vi "PRCBE 2600B Test Software V1.0.vi"() -> ()   [LabVIEW 2017]
doc: "Configures a sweep and takes voltage and current readings at each point."
uses:
  <vilib>/Platform/TimedLoop/XDataNode/timing_clust.ctl
  <vilib>/Platform/TimedLoop/XDataNode/nitl_modes.ctl
  <vilib>/Platform/TimedLoop/XDataNode/wakeup.ctl
  <vilib>/Utility/miscctls.llb/LVForegroundBackgroundColorsTypeDef.ctl
  <vilib>/Utility/miscctls.llb/LVSelectionTypeDef.ctl
  <vilib>/Utility/miscctls.llb/LVRowAndColumnUnsignedTypeDef.ctl
  SubVI/Global 1.vi
  <vilib>/Platform/TimedLoop/XDataNode/XDataNode.xnode
  <vilib>/Platform/TimedLoop/XDataNode/XDNodeRunTimeDep.lvlib
  <instrlib>/Keithley 2600 Series/Keithley 2600 Series.lvlib
panel:
  out "XY图":cluster{dbl[], dbl[]}(graph)
  in  "Channel":u16(ring) items=["Channel A", "Channel B"]
  in  "MOSFET CLUS":T1={"StepUnit"=1, "Gate Step"=1.0, "StoptUnit"=1, "StartUnit"=1, "Gate Stop"=10.0, "Gate Start"=-10.0, "Compliance"=0.1, "CompliancetUnit "=2, "Drain "=10.0} {"Drain" min=-200.0 max=200.0 step=0.001 format="%#.3f"; "CompliancetUnit" items=["μA", "mA", "A"]; "StepUnit" items=["mV", "V"]; "Gate Step" min=0.001 max=200.0 step=0.001 format="%#.3f"; "StoptUnit" items=["mV", "V"]; "StartUnit" items=["mV", "V"]; "Gate Stop" min=-200.0 max=200.0 step=0.001 format="%#.3f"; "Gate Start" min=-200.0 max=200.0 step=0.001 format="%#.3f"; "Compliance" min=0.1 max=10 step=1 format="%#.3f"}
  out "RES 4":dbl
  out "RES 3":dbl
  in  "pointsIT 2":u32=10 caption="DataPoints" min=3 max=50000 step=1
  in  "Delay time IT 2":u32=10 caption="Interval time" min=1 max=100000 step=1
  in  "delaytimeUnit IT 2":u16(ring) items=["μs", "ms", "s"]
  out "Sheet 23":string[][](table)
  in  "delaytimeUnit IT":u16(ring) items=["μs", "ms", "s"]
  in  "Delay time IT":u32=10 caption="Interval time" min=1 max=100000 step=1
  in  "pointsIT":u32=10 caption="DataPoints" min=3 max=50000 step=1
  in  "DataPoints":u32=21
  out "Sheet 22":string[][](table)
  out "RES 2":dbl
  in  "Vt CLUS":T2={"Current VT"=-10.0, "CurrUnit VT"=2, "Compliance"=0.1, "CompUnit VT"=1} {"CompUnit VT" items=["mV", "V"]; "Compliance" min=0.001 max=200 step=0.1 format="%#.3f"; "CurrUnit VT" items=["μA", "mA", "A"]; "Current VT" min=0.10000000149011612 max=10.0 step=0.001 format="%#.3f"}
  in  "It CLUS":T3={"VoltageUnit IT"=1, "Voltage IT"=-10.0, "CompCurrIT"=0.1, "CompUnit-IT"=2} {"CompUnit-IT" items=["μA", "mA", "A"]; "VoltageUnit IT" items=["mV", "V"]; "Voltage IT" min=0.001 max=200.0 step=0.001 format="%#.3f"; "CompCurrIT" min=0.1 max=10 step=0.001 format="%#.3f"}
  in  "IV CLUS":T4={"StepUnit"=1, "Step"=1.0, "StoptUnit"=1, "StartUnit"=1, "Stop"=10.0, "Start "=-10.0, "Compliance"=0.1, "CompliancetUnit "=2} {"CompliancetUnit" items=["μA", "mA", "A"]; "StepUnit" items=["mV", "V"]; "Step" min=0.001 max=200.0 step=0.001 format="%#.3f"; "StoptUnit" items=["mV", "V"]; "StartUnit" items=["mV", "V"]; "Stop" min=-200.0 max=200.0 step=0.001 format="%#.3f"; "Start" min=-200.0 max=200.0 step=0.001 format="%#.3f"; "Compliance" min=0.1 max=10 step=1 format="%#.3f"}
  in  "Test Type":enum32{"IV", "IT", "VT", "MOSFET"}(radio)
  in  "Series 2600B":u16(ring) items=["2601B  40V, 10A,100fA", "2602B  40V, 10A,100fA", "2604B  40V, 10A,100fA", "2611B  200V, 10A,100fA", "2612B  200V, 10A,100fA", "2614B  200V, 10A,100fA", "2634B  200V, 10A,1fA", "2635B  200V, 10A,0.1fA", "2636B  200V, 10A,0.1fA"]
  in  "Move All":bool
  in  "Save All":bool
  in  "Clear":bool
  in  "Append":bool
  in  "Stop But":bool
  in  "Repeat":bool
  in  "Save":bool
  in  "SetOK":bool
  in  "Tab Control":T5(tab)
  out "Sheet":string[][](table)
  out "Sheet 2":string[][](table) caption="Sheet"
  out "Sheet 3":string[][](table) caption="Sheet"
  out "Sheet 4":string[][](table) caption="Sheet"
  out "Sheet 5":string[][](table) caption="Sheet"
  out "Sheet 6":string[][](table) caption="Sheet"
  out "Sheet 7":string[][](table) caption="Sheet"
  out "Sheet 8":string[][](table) caption="Sheet"
  out "Sheet 9":string[][](table) caption="Sheet"
  out "Sheet 10":string[][](table) caption="Sheet"
  out "Sheet 11":string[][](table) caption="Sheet"
  out "Sheet 12":string[][](table) caption="Sheet"
  out "Sheet 13":string[][](table) caption="Sheet"
  out "Sheet 14":string[][](table) caption="Sheet"
  out "Sheet 15":string[][](table) caption="Sheet"
  out "Sheet 16":string[][](table) caption="Sheet"
  out "Sheet 17":string[][](table) caption="Sheet"
  out "Sheet 18":string[][](table) caption="Sheet"
  out "Sheet 19":string[][](table) caption="Sheet"
  out "Sheet 20":string[][](table) caption="Sheet"
  out "Sheet 21":string[][](table) caption="Sheet"
  out "RunState":cluster{"Boolean":bool}
  in  "XYConvert":bool
  out "test time":string
  out "Chart":cluster{dbl[], dbl[]}[](graph)
  in  "Source Mode  (0: Voltage)":u16(ring) items=["Voltage", "Current"]
  out "TempChart":cluster{sgl[], dbl[]}[](array[cluster])
  out "AppArray":bool[](array[boolean])
  out "test time":timestamp
  out "RES":dbl
  in  "EXIT":bool
  # "Test Function Parameters"
  # "Chart"
  # "PRCBE  2600B - I-V/I-t/V-t Test Software"
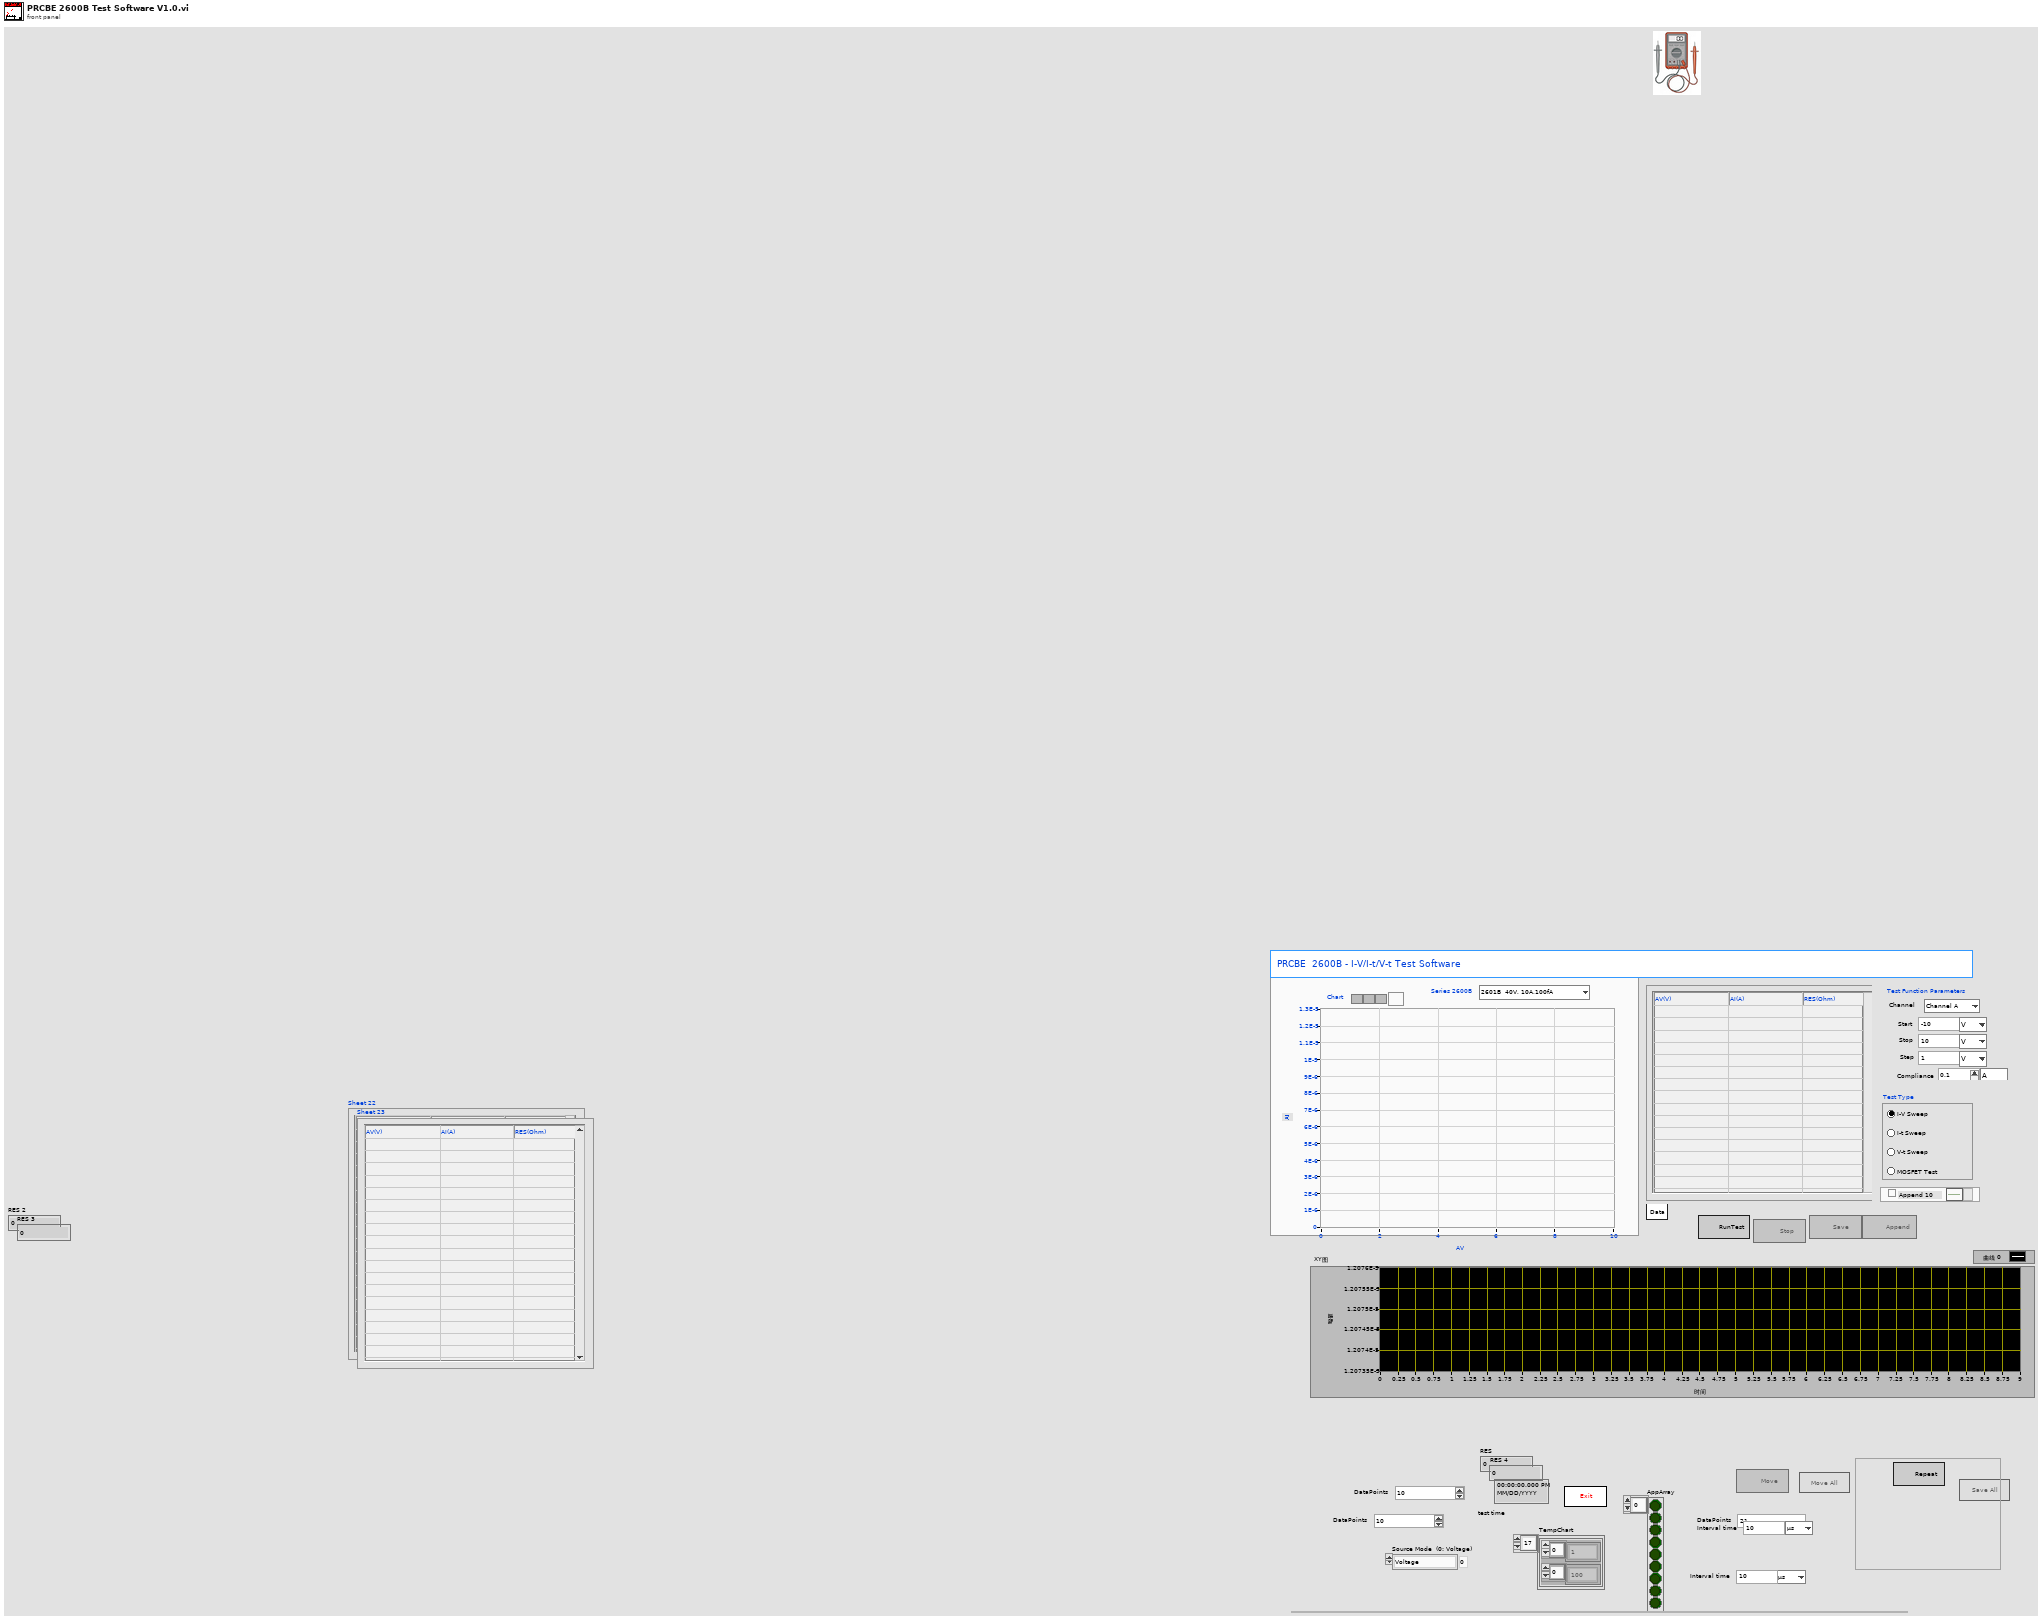
[diagram p1: front panel]
types:
  T1 = cluster{"StepUnit":u16, "Gate Step":dbl, "StoptUnit":u16, "StartUnit":u16, "Gate Stop":dbl, "Gate Start":dbl, "Compliance":sgl, "CompliancetUnit ":u16, "Drain ":dbl}
  T2 = cluster{"Current VT":dbl, "CurrUnit VT":u16, "Compliance":sgl, "CompUnit VT":u16}
  T3 = cluster{"VoltageUnit IT":u16, "Voltage IT":dbl, "CompCurrIT":sgl, "CompUnit-IT":u16}
  T4 = cluster{"StepUnit":u16, "Step":dbl, "StoptUnit":u16, "StartUnit":u16, "Stop":dbl, "Start ":dbl, "Compliance":sgl, "CompliancetUnit ":u16}
  T5 = enum32{"Data", "Append 1", "Append 2", "Append 3", "Append 4", "Append 5", "Append 6", "Append 7", "Append 8", "Append 9", "Append 10", "Append 11", "Append 12", "Append 13", "Append 14", "Append 15", "Append 16", "Append 17", "Append 18", "Append 19", "Append 20"}
  T6 = cluster{"Baud Rate":u32, "Parity":u16, "Data Bits":u16, "Stop Bits":u16, "Flow Control":u16}
  T7 = enum8{"Enabled", "Disabled", "Disabled and Grayed Out"}
  T8 = typedef "XDNodeRunTimeDep.lvlib/timing_clust.ctl" = cluster{"Expected End [f-1]":u64, "Actual End [f-1]":u64, "Finished Late? [f-1]":bool, "Expected End [i-1]":u64, "Actual End [i-1]":u64, "Finished Late? [i-1]":bool, "Expected Start [i]":u64, "Actual Start [i]":u64, "Expected Start [f]":u64, "Actual Start [f]":u64, "Source Name":string, "Structure Name":string, "Period":i64, "Deadline":i64, "Offset":i64, "Start":i64, "Priority":i32, "Timeout":i32, "Mode":T9, "Wakeup Reason":T10, "Error":errorcluster, "Source Type":string, "Secondary Source Type":string, "Global End Time":u64, "Global Start Time":u64, "Frame Duration":u64, "Iteration Duration":u64, "Assigned CPU":i32, "I/O Scan Engine Mode":u32}
  T9 = typedef "XDNodeRunTimeDep.lvlib/nitl_modes.ctl" = enum32{"No Change", "Process missed periods, maintain original phase", "Discard missed periods, maintain original phase", "Process missed periods, ignore original phase", "Discard missed periods, ignore original phase"}
  T10 = typedef "XDNodeRunTimeDep.lvlib/wakeup.ctl" = enum32{"Normal", "Aborted", "Asynchronous wakeup", "Timing source error", "Timed loop error", "Timeout"}
  T11 = cluster{"A 3":string[][], "A 4":string[][], "A 5":string[][], "A 6":string[][], "A 7":string[][], "A 8":string[][], "A 9":string[][], "A 10":string[][], "A 11":string[][], "A 12":string[][], "A 13":string[][], "A 14":string[][], "A 15":string[][], "A 16":string[][], "A 17":string[][], "A 18":string[][], "A 19":string[][], "A 20":string[][], "A 1":string[][], "A 2":string[][]}
  T12 = typedef "LVForegroundBackgroundColorsTypeDef.ctl" = cluster{"Foreground Color":u32, "Background Color":u32}
  T13 = typedef "LVSelectionTypeDef.ctl" = cluster{"Selection Start":u32, "Selection End":u32}
  T14 = enum32{"Current", "Voltage", "IV", "Resistance", "Power"}
  T15 = typedef "LVRowAndColumnUnsignedTypeDef.ctl" = cluster{"Row":u32, "Column":u32}
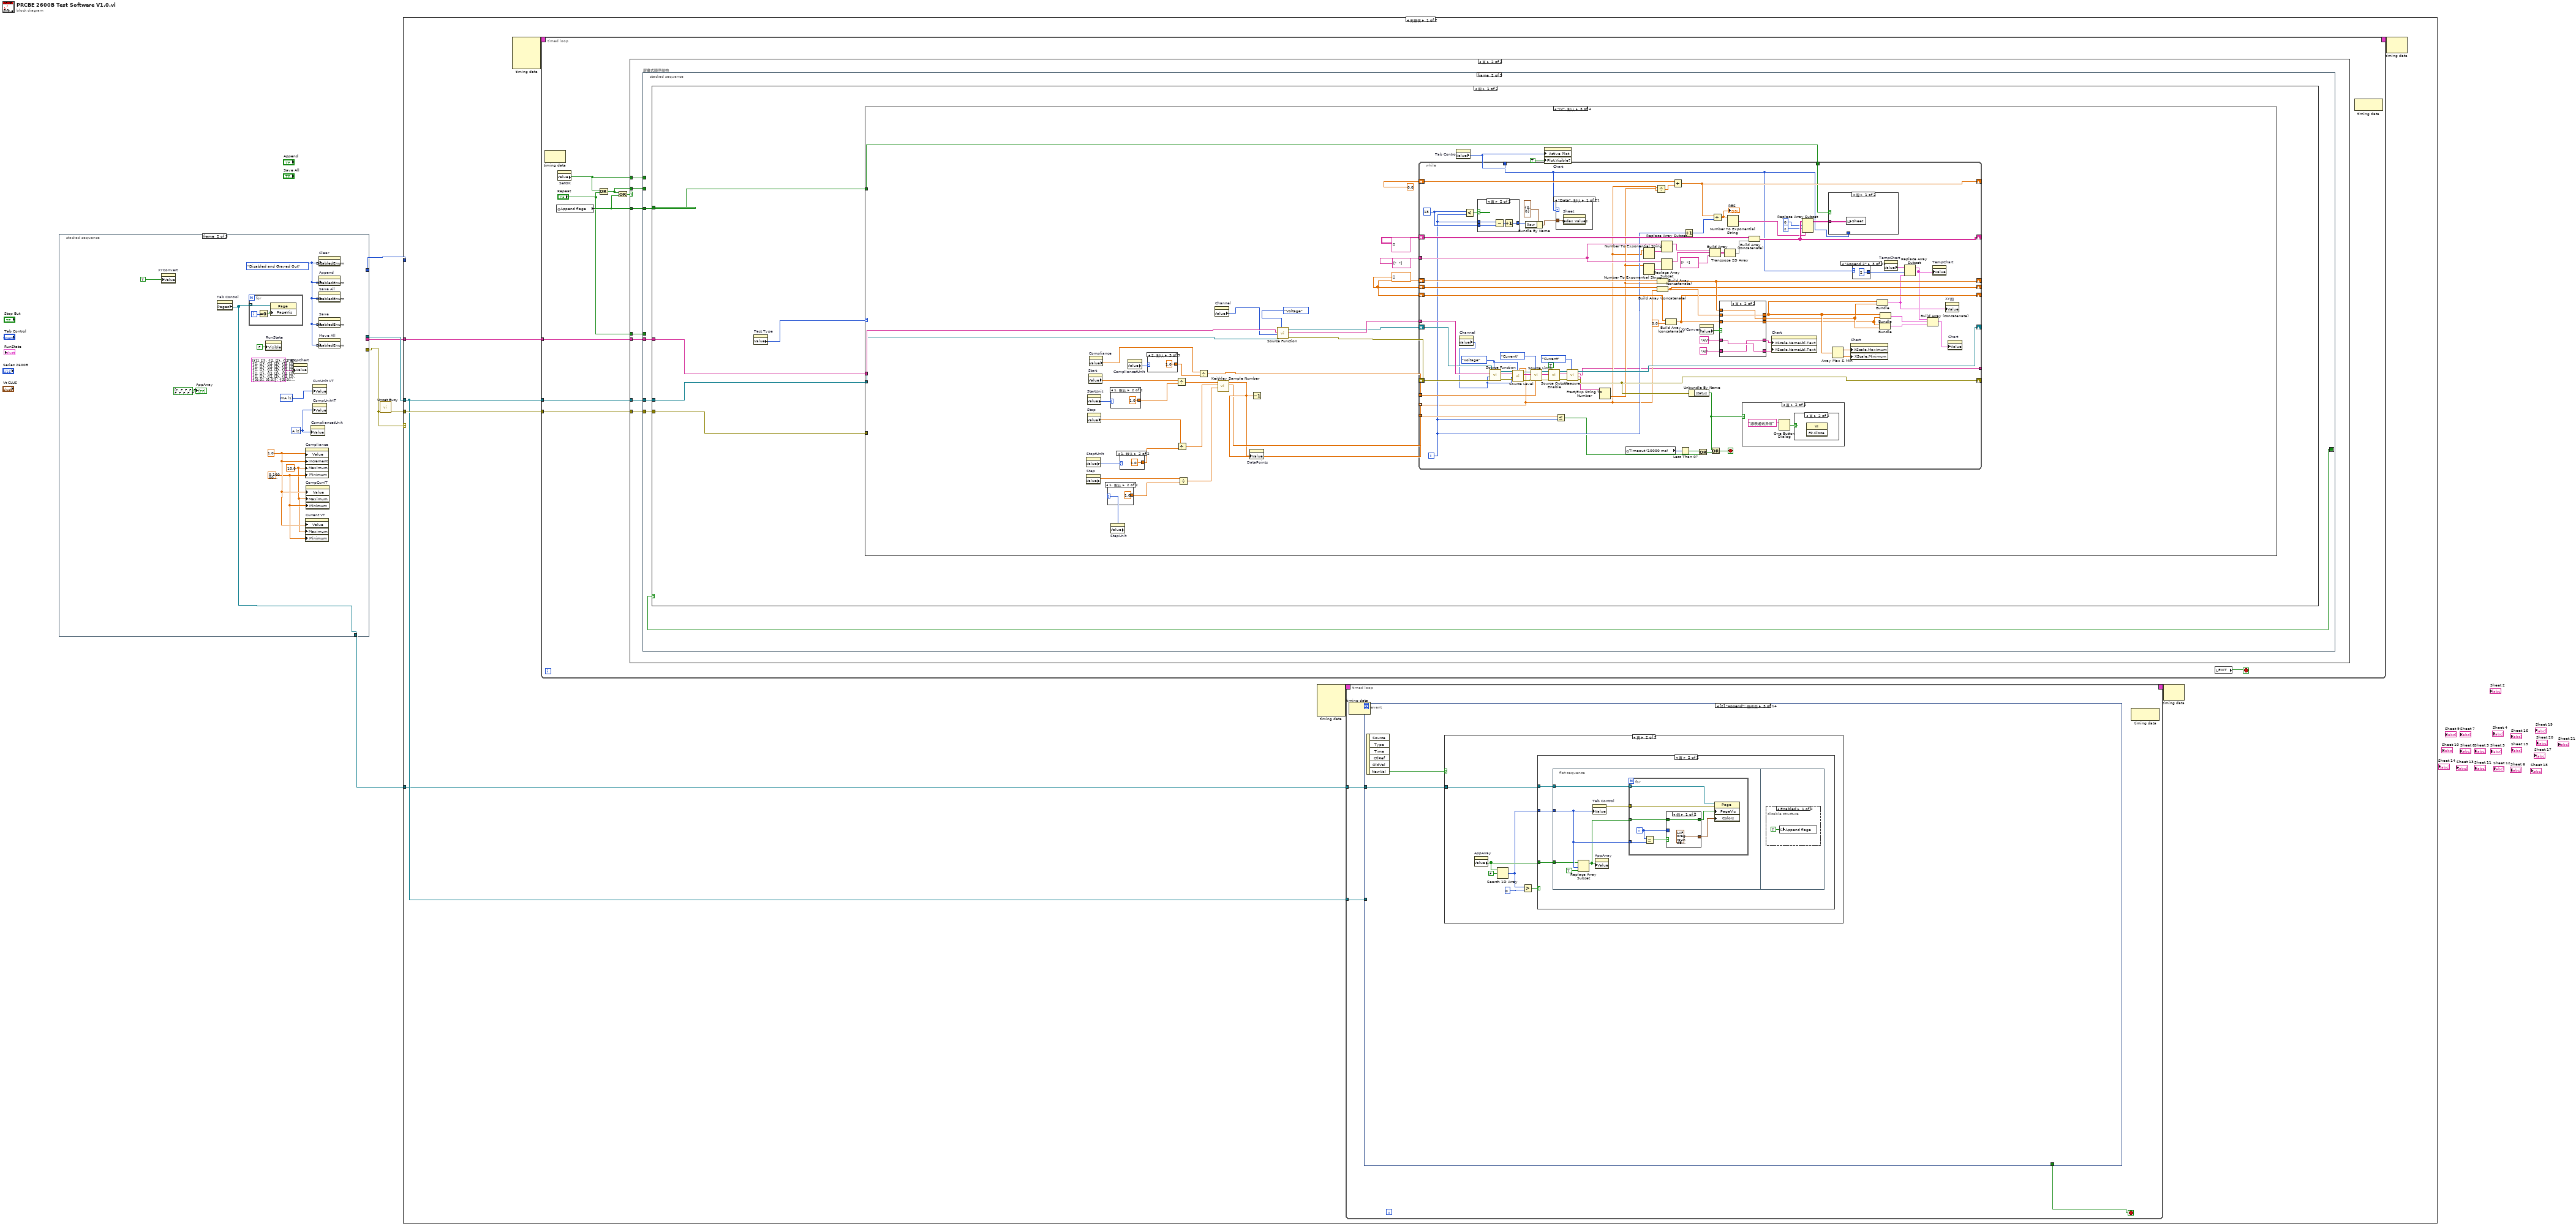
[diagram p0: block diagram]
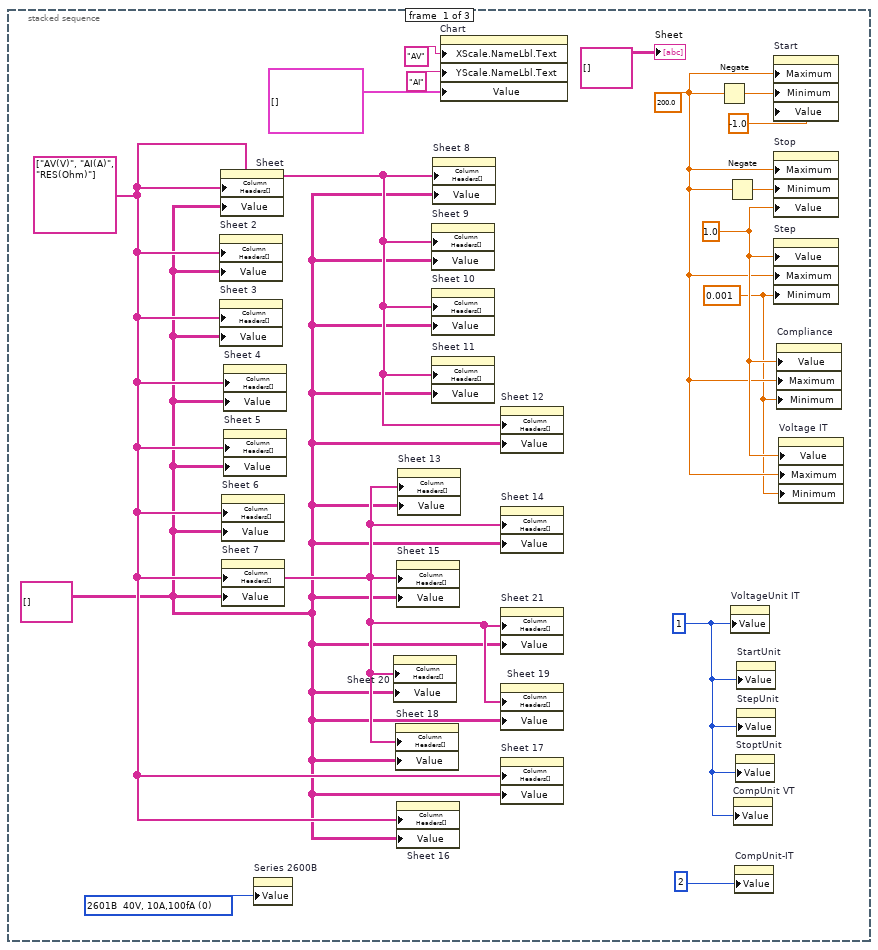
[diagram p2: hidden frame]
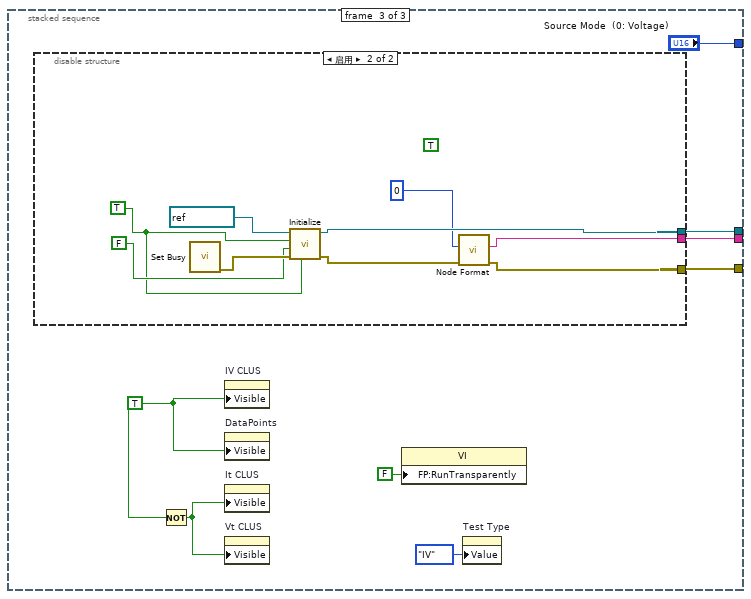
[diagram p3: hidden frame]
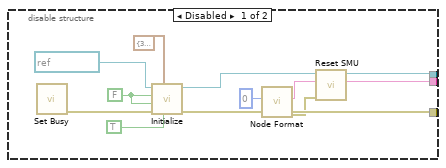
[diagram p4: hidden frame]
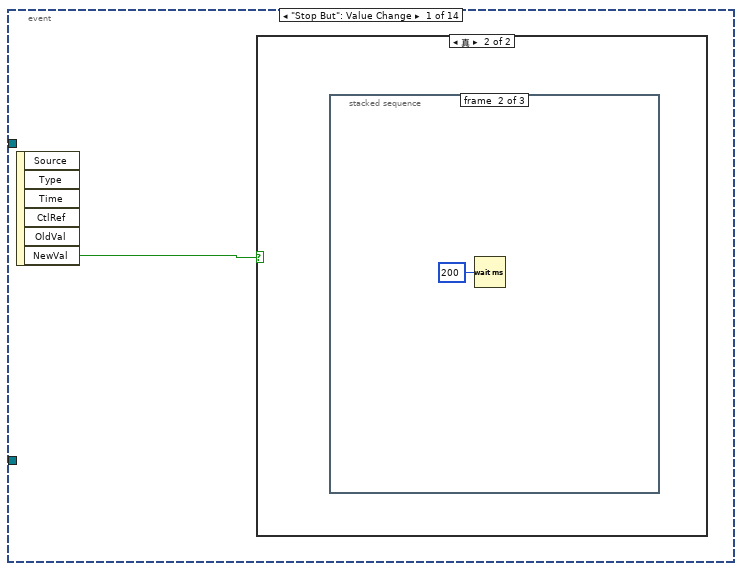
[diagram p5: hidden frame]
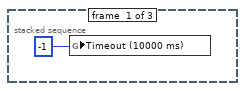
[diagram p7: hidden frame]
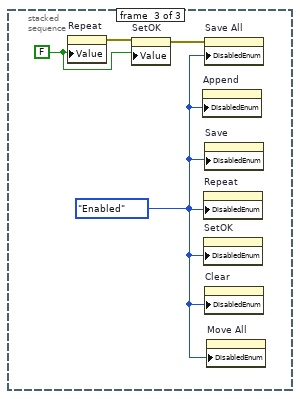
[diagram p8: hidden frame]
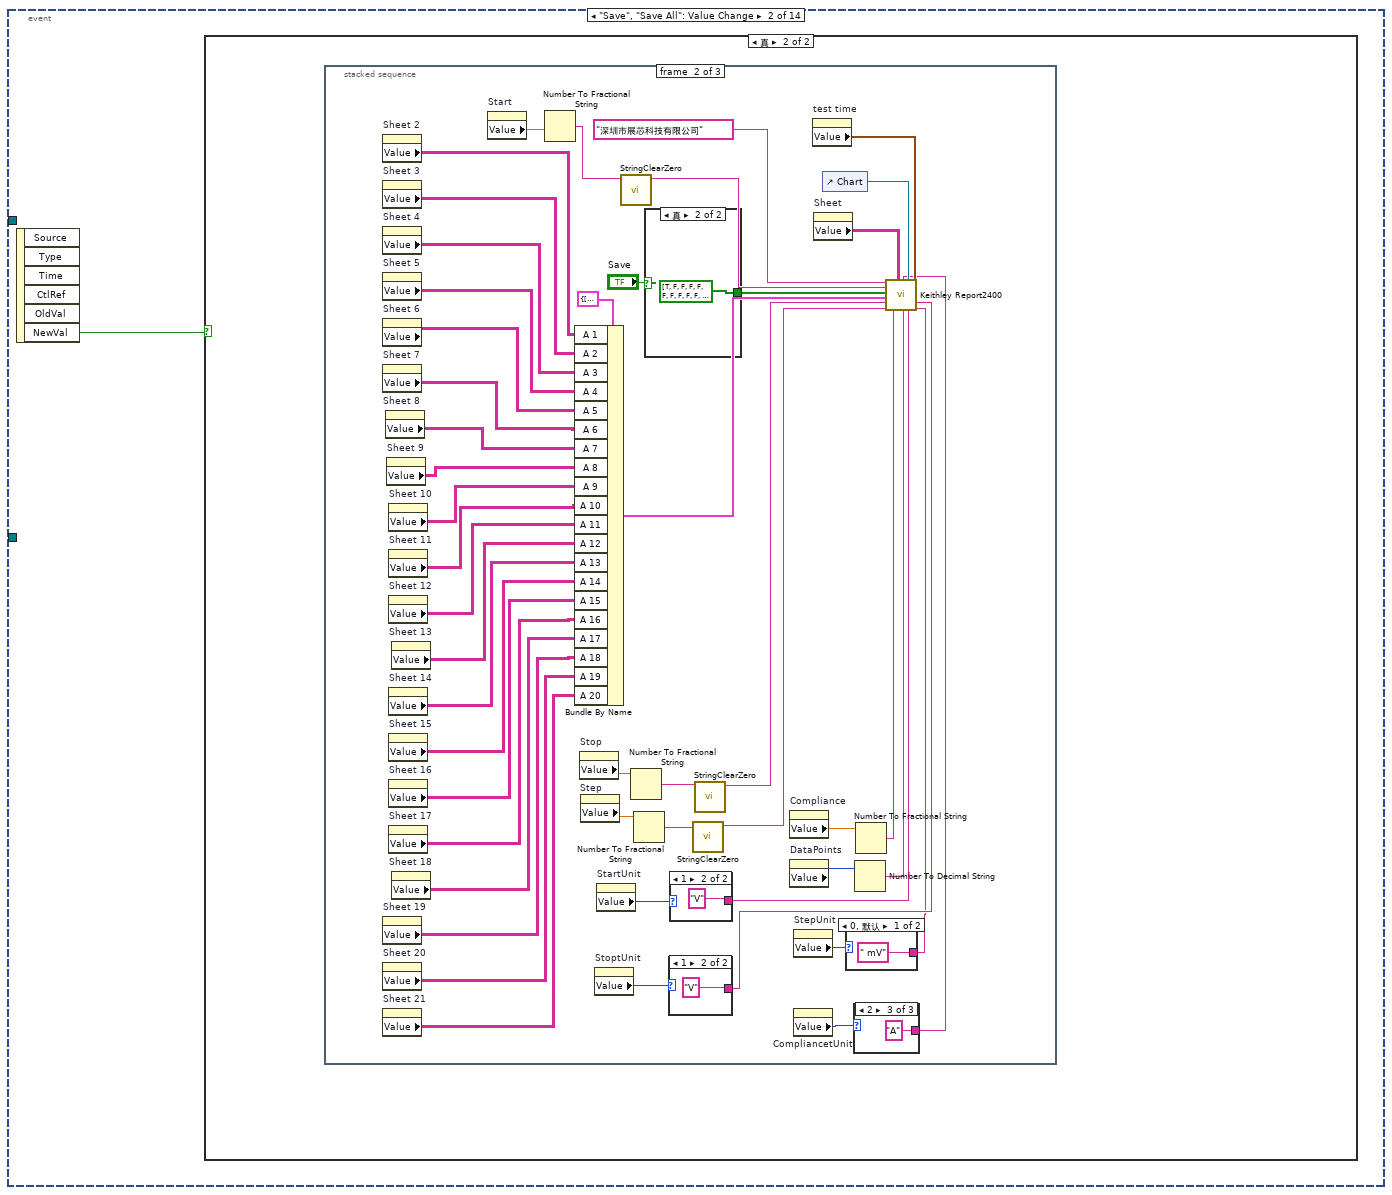
[diagram p9: hidden frame]
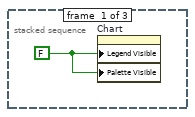
[diagram p11: hidden frame]
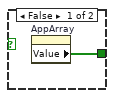
[diagram p12: hidden frame]
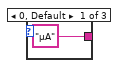
[diagram p13: hidden frame]
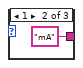
[diagram p14: hidden frame]
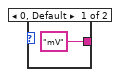
[diagram p15: hidden frame]
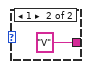
[diagram p16: hidden frame]
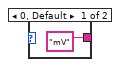
[diagram p17: hidden frame]
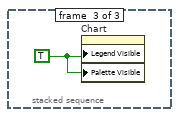
[diagram p18: hidden frame]
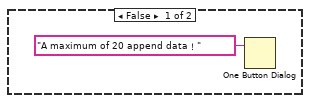
[diagram p20: hidden frame]
diagram:
  n1 = stacked-sequence {
    tunnel: [_ _ "Source Mode  (0: Voltage)"] -> w6
    tunnel: [_ _ w42] -> w5
    tunnel: [_ _ w41] -> w1
    tunnel: [_ w23 _] -> w3
    tunnel: [_ _ w39] -> w2
    frame #0 {
      w8 = u16 1 ("Value")
      w9 = u16 0 items=["2601B  40V, 10A,100fA", "2602B  40V, 10A,100fA", "2604B  40V, 10A,100fA", "2611B  200V, 10A,100fA", "2612B  200V, 10A,100fA", "2614B  200V, 10A,100fA", "2634B  200V, 10A,1fA", "2635B  200V, 10A,0.1fA", "2636B  200V, 10A,0.1fA"] ("Series 2600A")
      w13 = string[][] [] ("Sheet 7")
      w14 = string[] ["AV(V)", "AI(A)", "RES(Ohm)"] ("Column Header Strings[]")
      w10 = 0.001 ("Data Entry Limits:Minimum")
      w11 = 200.0 ("Data Entry Limits:Maximum")
      w12 = 1.0 ("Start")
      n2 = property on="Sheet 2" class="Tbl (严格)"("Column Headers[]"=w14, "Value"=w13) -> ()  [unwired: 2 in, 2 out]
      n3 = property on="Sheet 3" class="Tbl (严格)"("Column Headers[]"=w14, "Value"=w13) -> ()  [unwired: 2 in, 2 out]
      n4 = property on="Sheet" class="Tbl (严格)"("Column Headers[]"=w14, "Value"=w13) -> ()  [unwired: 2 in, 2 out]
      n5 = property on="Sheet 6" class="Tbl (严格)"("Column Headers[]"=w14, "Value"=w13) -> ()  [unwired: 2 in, 2 out]
      n6 = property on="Sheet 7" class="Tbl (严格)"("Column Headers[]"=w14, "Value"=w13) -> ()  [unwired: 2 in, 2 out]
      n7 = property on="Sheet 4" class="Tbl (严格)"("Column Headers[]"=w14, "Value"=w13) -> ()  [unwired: 2 in, 2 out]
      n8 = property on="Sheet 5" class="Tbl (严格)"("Column Headers[]"=w14, "Value"=w13) -> ()  [unwired: 2 in, 2 out]
      n9 = property on="Series 2600B" class="Ring (严格)"("Value"=w9) -> ()  [unwired: 2 in, 2 out]
      n10 = property on="Sheet 20" class="Tbl (严格)"("Column Headers[]"=w14, "Value"=w13) -> ()  [unwired: 2 in, 2 out]
      n11 = property on="Sheet 18" class="Tbl (严格)"("Column Headers[]"=w14, "Value"=w13) -> ()  [unwired: 2 in, 2 out]
      n12 = property on="Sheet 15" class="Tbl (严格)"("Column Headers[]"=w14, "Value"=w13) -> ()  [unwired: 2 in, 2 out]
      n13 = property on="Sheet 16" class="Tbl (严格)"("Column Headers[]"=w14, "Value"=w13) -> ()  [unwired: 2 in, 2 out]
      n14 = property on="Sheet 13" class="Tbl (严格)"("Column Headers[]"=w14, "Value"=w13) -> ()  [unwired: 2 in, 2 out]
      n15 = property on="Sheet 9" class="Tbl (严格)"("Column Headers[]"=w14, "Value"=w13) -> ()  [unwired: 2 in, 2 out]
      n16 = property on="Sheet 10" class="Tbl (严格)"("Column Headers[]"=w14, "Value"=w13) -> ()  [unwired: 2 in, 2 out]
      n17 = property on="Sheet 11" class="Tbl (严格)"("Column Headers[]"=w14, "Value"=w13) -> ()  [unwired: 2 in, 2 out]
      n18 = property on="Sheet 8" class="Tbl (严格)"("Column Headers[]"=w14, "Value"=w13) -> ()  [unwired: 2 in, 2 out]
      n19 = property on="Chart" class="XYGraph (严格)"("XScale.NameLbl.Text"="AV" ("X Scale.Name Label.Text"), "YScale.NameLbl.Text"="AI" ("Y Scale.Name Label.Text"), "Value"=cluster{dbl[], dbl[]}[] [] ("Chart")) -> ()  [unwired: 2 in, 2 out]
      n20 = property on="Sheet 12" class="Tbl (严格)"("Column Headers[]"=w14, "Value"=w13) -> ()  [unwired: 2 in, 2 out]
      n21 = property on="Sheet 14" class="Tbl (严格)"("Column Headers[]"=w14, "Value"=w13) -> ()  [unwired: 2 in, 2 out]
      n22 = property on="Sheet 21" class="Tbl (严格)"("Column Headers[]"=w14, "Value"=w13) -> ()  [unwired: 2 in, 2 out]
      n23 = property on="Sheet 19" class="Tbl (严格)"("Column Headers[]"=w14, "Value"=w13) -> ()  [unwired: 2 in, 2 out]
      n24 = property on="Sheet 17" class="Tbl (严格)"("Column Headers[]"=w14, "Value"=w13) -> ()  [unwired: 2 in, 2 out]
      n25 = Negate(x=w11) -> (-x=w19:dbl)
      n26 = Negate(x=w11) -> (-x=w18:dbl)
      n27 = property on="VoltageUnit IT" class="Ring (严格)"("Value"=w8) -> ()  [unwired: 2 in, 2 out]
      n28 = property on="CompUnit VT" class="Ring (严格)"("Value"=w8) -> ()  [unwired: 2 in, 2 out]
      n29 = property on="CompUnit-IT" class="Ring (严格)"("Value"=u16 2) -> ()  [unwired: 2 in, 2 out]
      n30 = property on="StoptUnit" class="Ring (严格)"("Value"=w8) -> ()  [unwired: 2 in, 2 out]
      n31 = property on="StartUnit" class="Ring (严格)"("Value"=w8) -> ()  [unwired: 2 in, 2 out]
      n32 = property on="StepUnit" class="Ring (严格)"("Value"=w8) -> ()  [unwired: 2 in, 2 out]
      n33 = property on="Start" class="DigNum (严格)"("Maximum"=w11, "Minimum"=w19, "Value"=-1.0 ("Start")) -> ()  [unwired: 2 in, 2 out]
      n34 = property on="Stop" class="DigNum (严格)"("Maximum"=w11, "Minimum"=w18, "Value"=w12) -> ()  [unwired: 2 in, 2 out]
      n35 = property on="Step" class="DigNum (严格)"("Value"=w12, "Maximum"=w11, "Minimum"=w10) -> ()  [unwired: 2 in, 2 out]
      n36 = property on="Compliance" class="DigNum (严格)"("Value"=w12, "Maximum"=w11, "Minimum"=w10) -> ()  [unwired: 2 in, 2 out]
      n37 = property on="Voltage IT" class="DigNum (严格)"("Value"=w12, "Maximum"=w11, "Minimum"=w10) -> ()  [unwired: 2 in, 2 out]
      "Sheet" <- string[][] [] ("Sheet")
    }
    frame #1 {
      w22 = u16 1 items=["μA", "mA", "A"] ("CompliancetUnit")
      w26 = sgl 0.1 ("Compliance")
      w25 = 10.0 ("Data Entry Limits:Maximum")
      w27 = sgl 1.0 ("Compliance")
      w28 = u16 2 items=["μA", "mA", "A"] ("CompliancetUnit")
      w29 = T7."Disabled and Grayed Out" ("Disabled")
      n38 = property on="XYConvert" class="Bool (严格)"("Value"=TRUE) -> ()  [unwired: 2 in, 2 out]
      n39 = property on="Tab Control" class="TabCtl (严格)"() -> ("Pages"=w23:refnum<vi>[])  [unwired: 2 in, 2 out]
      n40 = for {
        tunnel: w23 -> [w34] mode=indexing
        i -> [w35]
        n41 = Equal To 0?(x=w35) -> (x = 0?=w33:bool)
        n42 = property class="Page"(reference=w34, "PageVis"=w33) -> ()  [unwired: 1 in, 2 out]
      }
      n43 = property on="RunState" class="Clust (严格)"("Visible"=FALSE) -> ()  [unwired: 2 in, 2 out]
      n44 = property on="TempChart" class="Arr (严格)"("Value"=cluster{dbl[], sgl[]}[] [{[], []}, {[], []}, {[], []}, {[], []}, {[], []}, {[], []}, {[], []}, {[], []}, {[], []}, {[], []}, {[], []}, {[], []}, {[], []}, {[], []}, {[], []}, {[], []}, {[], []}, {[], []}, {[0.0], [0.0]}, {[0.0], [0.0]}, {[0.0], [0.0]}] ("TempChart")) -> ()  [unwired: 2 in, 2 out]
      n45 = property on="Compliance" class="DigNum (严格)"("Value"=w27, "Increment"=w27, "Maximum"=w25, "Minimum"=w26) -> ()  [unwired: 2 in, 2 out]
      n46 = property on="Current VT" class="DigNum (严格)"("Value"=w27, "Maximum"=w25, "Minimum"=w26) -> ()  [unwired: 2 in, 2 out]
      n47 = property on="CompCurrIT" class="DigNum (严格)"("Value"=w27, "Maximum"=w25, "Minimum"=w26) -> ()  [unwired: 2 in, 2 out]
      n48 = property on="CompliancetUnit" class="Ring (严格)"("Value"=w28) -> ()  [unwired: 2 in, 2 out]
      n49 = property on="CurrUnit VT" class="Ring (严格)"("Value"=w22) -> ()  [unwired: 2 in, 2 out]
      n50 = property on="CompUnit-IT" class="Ring (严格)"("Value"=w28) -> ()  [unwired: 2 in, 2 out]
      n51 = property on="Clear" class="Bool (严格)"("DisabledEnum"=w29) -> ()  [unwired: 2 in, 2 out]
      n52 = property on="Append" class="Bool (严格)"("DisabledEnum"=w29) -> ()  [unwired: 2 in, 2 out]
      n53 = property on="Save All" class="Bool (严格)"("DisabledEnum"=w29) -> ()  [unwired: 2 in, 2 out]
      n54 = property on="Save" class="Bool (严格)"("DisabledEnum"=w29) -> ()  [unwired: 2 in, 2 out]
      n55 = property on="Move All" class="Bool (严格)"("DisabledEnum"=w29) -> ()  [unwired: 2 in, 2 out]
      "AppArray" <- bool[] [TRUE, FALSE, FALSE, FALSE, FALSE, FALSE, FALSE, FALSE, FALSE, FALSE, FALSE, FALSE, FALSE, FALSE, FALSE, FALSE, FALSE, FALSE, FALSE, FALSE, FALSE] ("AppArray")
    }
    frame #2 {
      w36 = TRUE ("Visible")
      n56 = disable-structure shown="启用" {
        disable-tunnel: [w45 w61] -> w42
        disable-tunnel: [w50 w58] -> w41
        disable-tunnel: [w44 w59] -> w39
        frame Disabled {
          w53 = FALSE ("ID Query (True)")
          n57 = call <vilib>:"Set Busy.vi"() -> ("error out"=w55:errorcluster)  [unwired: 10 in, 1 out]
          n58 = call <instrlib>:"Initialize.vi"("Reset (True)"=TRUE, 7:T6 {"Baud Rate"=38400, "Parity"=0, "Data Bits"=7, "Stop Bits"=10, "Flow Control"=0} ("Serial Configuration"), "error in (no error)"=w55, "Error Query (False)"=w53, "ID Query (True)"=w53, "VISA resource name"=refnum<visa-resource-name> "COM1") -> ("error out"=w50:errorcluster, "VISA resource name out"=w47:refnum<visa-resource-name>)  [unwired: 4 out]
          n59 = call <instrlib>:"Node Format.vi"("Node (0-64)"=i8 0) -> ("error out"=w49:errorcluster, "Formatted Node"=w48:string)  [unwired: 1 in, 8 out]
          n60 = call <instrlib>:"Reset SMU.vi"("error in (no error)"=w49, "Node In"=w48, "VISA resource name"=w47) -> ("Node Out"=w44:string, "VISA resource name out"=w45:refnum<visa-resource-name>)  [unwired: 2 in, 5 out]
        }
        frame Enabled {
          w56 = TRUE
          (unwired) TRUE
          n61 = call <vilib>:"Set Busy.vi"() -> ("error out"=w64:errorcluster)  [unwired: 10 in, 1 out]
          n62 = call <instrlib>:"Initialize.vi"("Reset (True)"=w56, "error in (no error)"=w64, "Error Query (False)"=FALSE, "ID Query (True)"=w56, "VISA resource name"=refnum<visa-resource-name> "COM1") -> ("error out"=w62:errorcluster, "VISA resource name out"=w61:refnum<visa-resource-name>)  [unwired: 5 out]
          n63 = call <instrlib>:"Node Format.vi"("error in"=w62, "Node (0-64)"=0) -> ("error out"=w58:errorcluster, "Formatted Node"=w59:string)  [unwired: 8 in]
        }
      }
      n64 = Not(x=w36) -> (.not. x?=w37:bool)
      n65 = property on="IV CLUS" class="Clust (严格)"("Visible"=w36) -> ()  [unwired: 2 in, 2 out]
      n66 = property on="DataPoints" class="DigNum (严格)"("Visible"=w36) -> ()  [unwired: 2 in, 2 out]
      n67 = property on="It CLUS" class="Clust (严格)"("Visible"=w37) -> ()  [unwired: 2 in, 2 out]
      n68 = property on="Vt CLUS" class="Clust (严格)"("Visible"=w37) -> ()  [unwired: 2 in, 2 out]
      n69 = property class="VI"("FP:RunTransparently"=FALSE ("Front Panel Window:Run VI Transparently")) -> ()  [unwired: 2 in, 2 out]
      n70 = property on="Test Type" class="RadioBtnsControl (严格)"("Value"=enum32{"IV", "IT", "VT", "MOSFET"}."IV" ("Test Type")) -> ()  [unwired: 2 in, 2 out]
    }
  }
  n71 = call <vilib>:"Unset Busy.vi"("error in (no error)"=w1) -> ("error out"=w4:errorcluster)  [unwired: 10 in]
  n72 = case shown="无错误" w1 {
    tunnel: w6 -> [_ _]
    tunnel: w4 -> [w72 _]
    tunnel: w5 -> [w71 _]
    tunnel: w3 -> [w70 _]
    tunnel: w2 -> [w65 _]
    frame No Error {
      n73 = node-c288() -> (w69:T8)  [unwired: 4 in]
      n74 = timed-loop {
        tunnel: w71 -> [w632]
        tunnel: w72 -> [w631]
        timing: w69 -> [_]
        timing-out: [_] -> w68
        tunnel: w65 -> [w624]
        stop <- w630 stop-if-true
        n75 = node-c288() -> ()  [unwired: 1 in, 1 out]
        n76 = global read "Global 1.vi" "Append flage"() -> (w629:bool)
        n77 = property on="SetOK" class="Bool (严格)"() -> ("Value"=w625:bool)  [unwired: 2 in, 2 out]
        n78 = Compound Arithmetic op=OR(w625, "Repeat") -> (w627:bool)
        n79 = Compound Arithmetic op=OR(w627, w629) -> (w628:bool)
        n80 = case shown="真" w628 {
          tunnel: w632 -> [_ w646]
          tunnel: w631 -> [_ w645]
          tunnel: w625 -> [_ w644]
          tunnel: w629 -> [_ w643]
          tunnel: w627 -> [_ w642]
          tunnel: "Repeat" -> [_ w641]
          tunnel: w624 -> [_ w640]
          frame False {
            n81 = global read "Global 1.vi" "Timeout (10000 ms)"() -> (w636:i32)
            n82 = Greater Than 0?(x=w636) -> (x > 0?=w635:bool)
            n83 = case shown="真" w635 {
              frame False {
                w639 = T7."Enabled" ("Disabled")
                n84 = global write "Global 1.vi" "Timeout (10000 ms)"(100000 ("Timeout (10000 ms)")) -> ()
                n85 = property on="Append" class="Bool (严格)"("DisabledEnum"=w639) -> ()  [unwired: 2 in, 2 out]
                n86 = property on="Repeat" class="Bool (严格)"("DisabledEnum"=w639) -> ()  [unwired: 2 in, 2 out]
                n87 = property on="SetOK" class="Bool (严格)"("DisabledEnum"=w639) -> ()  [unwired: 2 in, 2 out]
                n88 = property on="Save All" class="Bool (严格)"("DisabledEnum"=w639) -> ()  [unwired: 2 in, 2 out]
                n89 = property on="Save" class="Bool (严格)"("DisabledEnum"=w639) -> ()  [unwired: 2 in, 2 out]
                n90 = property on="Clear" class="Bool (严格)"("DisabledEnum"=w639) -> ()  [unwired: 2 in, 2 out]
                n91 = property on="Move All" class="Bool (严格)"("DisabledEnum"=w639) -> ()  [unwired: 2 in, 2 out]
                n92 = property on="Stop But" class="Bool (严格)"("DisabledEnum"=T7."Disabled and Grayed Out" ("Disabled")) -> ()  [unwired: 2 in, 2 out]
              }
              frame True {
              }
            }
          }
          frame True {
            n93 = stacked-sequence "层叠式顺序结构" {
              seq-local: [w649 _ _] -> [_ w730 _]
              tunnel: w646 -> [_ w732 _]
              tunnel: w645 -> [_ w731 _]
              tunnel: w644 -> [_ _ w1588]
              tunnel: w643 -> [w647 w733 w1586]
              tunnel: w642 -> [w648 _ _]
              tunnel: w641 -> [_ _ w1584]
              tunnel: w640 -> [_ w729 _]
              frame #0 {
                n94 = property on="Start" class="DigNum (严格)"() -> ("Value"=w650:dbl)  [unwired: 2 in, 2 out]
                n95 = property on="StartUnit" class="Ring (严格)"() -> ("Value"=w656:u16)  [unwired: 2 in, 2 out]
                n96 = property on="StoptUnit" class="Ring (严格)"() -> ("Value"=w658:u16)  [unwired: 2 in, 2 out]
                n97 = case shown="1, 默认" w658 {
                  tunnel: [1000.0 ("Start") 1.0 ("Start")] -> w655
                  frame 0 {
                  }
                  frame 1, Default {
                  }
                }
                n98 = case shown="1, 默认" w656 {
                  tunnel: [1000.0 ("Start") 1.0 ("Start")] -> w653
                  frame 0 {
                  }
                  frame 1, Default {
                  }
                }
                n99 = property on="StepUnit" class="Ring (严格)"() -> ("Value"=w657:u16)  [unwired: 2 in, 2 out]
                n100 = property on="Step" class="DigNum (严格)"() -> ("Value"=w652:dbl)  [unwired: 2 in, 2 out]
                n101 = property on="Stop" class="DigNum (严格)"() -> ("Value"=w651:dbl)  [unwired: 2 in, 2 out]
                n102 = Divide(x=w650, y=w653) -> (x/y=w660:dbl)
                n103 = Divide(x=w651, y=w655) -> (x/y=w659:dbl)
                n104 = case shown="1, 默认" w657 {
                  tunnel: [1000.0 ("Start") 1.0 ("Start")] -> w654
                  frame 0 {
                  }
                  frame 1, Default {
                  }
                }
                n105 = Subtract(x=w659, y=w660) -> (x-y=w661:dbl)
                n106 = Divide(x=w652, y=w654) -> (x/y=w663:dbl)
                n107 = Absolute Value(x=w661) -> (abs(x)=w662:dbl)
                n108 = Less?(x=w662, y=w663) -> (x < y?=w664:bool)
                n109 = case shown="假" w664 {
                  selector: w664 -> [_ w721]
                  tunnel: w652 -> [w675 _]
                  tunnel: w651 -> [w674 _]
                  tunnel: w650 -> [w673 _]
                  tunnel: [w667 w721] -> w649
                  tunnel: w648 -> [w666 _]
                  tunnel: w647 -> [w665 _]
                  frame False {
                    n110 = Equal To 0?(x=w674) -> (x = 0?=w672:bool)
                    n111 = Equal To 0?(x=w673) -> (x = 0?=w671:bool)
                    n112 = Equal To 0?(x=w675) -> (x = 0?=w669:bool)
                    n113 = And(x=w672, y=w671) -> (x .and. y?=w670:bool)
                    n114 = Or(x=w670, y=w669) -> (x .or. y?=w668:bool)
                    n115 = case shown="假" w668 {
                      selector: w668 -> [w691 w718]
                      tunnel: [w691 w718] -> w667
                      tunnel: w666 -> [w677 _]
                      tunnel: w665 -> [w678 _]
                      frame False {
                        w676 = string[][] [] ("Sheet")
                        w690 = T7."Disabled and Grayed Out" ("Disabled")
                        n116 = Get Date/Time In Seconds() -> (seconds since 1Jan1904=w685:timestamp)
                        "test time" <- w685
                        n117 = case shown="假" w678 {
                          tunnel: w676 -> [w694 w696]
                          frame False {
                            n118 = local write "Sheet"(w694) -> ()
                          }
                          frame True {
                            n119 = property on="Tab Control" class="TabCtl (严格)"() -> ("Value"=w695:T5)  [unwired: 2 in, 2 out]
                            n120 = case shown="\"Append 3\"" w695 {
                              tunnel: w696 -> [_ w697 w698 w699 w700 w701 w702 w703 w704 w705 w706 w707 w708 w709 w710 w711 w712 w713 w714 w715 w716]
                              frame "Data", Default {
                              }
                              frame "Append 1" {
                                n121 = property on="Sheet 2" class="Tbl (严格)"("Value"=w697) -> ()  [unwired: 2 in, 2 out]
                              }
                              frame "Append 2" {
                                n122 = property on="Sheet 3" class="Tbl (严格)"("Value"=w698) -> ()  [unwired: 2 in, 2 out]
                              }
                              frame "Append 3" {
                                n123 = property on="Sheet 4" class="Tbl (严格)"("Value"=w699) -> ()  [unwired: 2 in, 2 out]
                              }
                              frame "Append 4" {
                                n124 = property on="Sheet 5" class="Tbl (严格)"("Value"=w700) -> ()  [unwired: 2 in, 2 out]
                              }
                              frame "Append 5" {
                                n125 = property on="Sheet 6" class="Tbl (严格)"("Value"=w701) -> ()  [unwired: 2 in, 2 out]
                              }
                              frame "Append 6" {
                                n126 = property on="Sheet 7" class="Tbl (严格)"("Value"=w702) -> ()  [unwired: 2 in, 2 out]
                              }
                              frame "Append 7" {
                                n127 = property on="Sheet 8" class="Tbl (严格)"("Value"=w703) -> ()  [unwired: 2 in, 2 out]
                              }
                              frame "Append 8" {
                                n128 = property on="Sheet 9" class="Tbl (严格)"("Value"=w704) -> ()  [unwired: 2 in, 2 out]
                              }
                              frame "Append 9" {
                                n129 = property on="Sheet 10" class="Tbl (严格)"("Value"=w705) -> ()  [unwired: 2 in, 2 out]
                              }
                              frame "Append 10" {
                                n130 = property on="Sheet 11" class="Tbl (严格)"("Value"=w706) -> ()  [unwired: 2 in, 2 out]
                              }
                              frame "Append 11" {
                                n131 = property on="Sheet 12" class="Tbl (严格)"("Value"=w707) -> ()  [unwired: 2 in, 2 out]
                              }
                              frame "Append 12" {
                                n132 = property on="Sheet 13" class="Tbl (严格)"("Value"=w708) -> ()  [unwired: 2 in, 2 out]
                              }
                              frame "Append 13" {
                                n133 = property on="Sheet 14" class="Tbl (严格)"("Value"=w709) -> ()  [unwired: 2 in, 2 out]
                              }
                              frame "Append 14" {
                                n134 = property on="Sheet 15" class="Tbl (严格)"("Value"=w710) -> ()  [unwired: 2 in, 2 out]
                              }
                              frame "Append 15" {
                                n135 = property on="Sheet 16" class="Tbl (严格)"("Value"=w711) -> ()  [unwired: 2 in, 2 out]
                              }
                              frame "Append 16" {
                                n136 = property on="Sheet 17" class="Tbl (严格)"("Value"=w712) -> ()  [unwired: 2 in, 2 out]
                              }
                              frame "Append 17" {
                                n137 = property on="Sheet 18" class="Tbl (严格)"("Value"=w713) -> ()  [unwired: 2 in, 2 out]
                              }
                              frame "Append 18" {
                                n138 = property on="Sheet 19" class="Tbl (严格)"("Value"=w714) -> ()  [unwired: 2 in, 2 out]
                              }
                              frame "Append 19" {
                                n139 = property on="Sheet 20" class="Tbl (严格)"("Value"=w715) -> ()  [unwired: 2 in, 2 out]
                              }
                              frame "Append 20" {
                                n140 = property on="Sheet 21" class="Tbl (严格)"("Value"=w716) -> ()  [unwired: 2 in, 2 out]
                              }
                            }
                          }
                        }
                        n141 = case shown="真" w677 {
                          tunnel: w676 -> [_ w693]
                          frame False {
                          }
                          frame True {
                            n142 = property on="Sheet" class="Tbl (严格)"("Value"=w693) -> ()  [unwired: 2 in, 2 out]
                            n143 = property on="Tab Control" class="TabCtl (严格)"("Value"=T5."Data" ("Tab Control")) -> ()  [unwired: 2 in, 2 out]
                          }
                        }
                        n144 = Get Date/Time String(date format (0)=enum16{"short", "long", "abbreviated"}."short", seconds (now)=w685, want seconds? (F)=TRUE) -> (date string=w683:string, time string=w687:string)
                        n145 = Concatenate Strings(w683, "  " ("string"), w687) -> (→"test time":string)
                        n146 = property on="Stop But" class="Bool (严格)"("DisabledEnum"=T7."Enabled" ("Disabled")) -> ()  [unwired: 2 in, 2 out]
                        n147 = global write "Global 1.vi" "Timeout (10000 ms)"(100000 ("Timeout (10000 ms)")) -> ()
                        n148 = property on="Clear" class="Bool (严格)"("DisabledEnum"=w690) -> ()  [unwired: 2 in, 2 out]
                        n149 = property on="Repeat" class="Bool (严格)"("DisabledEnum"=w690) -> ()  [unwired: 2 in, 2 out]
                        n150 = property on="SetOK" class="Bool (严格)"("DisabledEnum"=w690) -> ()  [unwired: 2 in, 2 out]
                        n151 = property on="Save" class="Bool (严格)"("DisabledEnum"=w690) -> ()  [unwired: 2 in, 2 out]
                        n152 = property on="Save All" class="Bool (严格)"("DisabledEnum"=w690) -> ()  [unwired: 2 in, 2 out]
                        n153 = property on="Append" class="Bool (严格)"("DisabledEnum"=w690) -> ()  [unwired: 2 in, 2 out]
                        n154 = property on="Move All" class="Bool (严格)"("DisabledEnum"=w690) -> ()  [unwired: 2 in, 2 out]
                        n155 = property on="Chart" class="XYGraph (严格)"("Value"=cluster{"Voltage":dbl[], "Current":dbl[]}[] [] ("Graph")) -> ()  [unwired: 2 in, 2 out]
                        n156 = property on="RunState" class="Clust (严格)"("Visible"=TRUE) -> ()  [unwired: 2 in, 2 out]
                      }
                      frame True {
                        w717 = FALSE ("Repeat")
                        n157 = property on="Repeat" class="Bool (严格)"("Value"=w717) -> ()  [unwired: 2 in, 2 out]
                        n158 = property on="SetOK" class="Bool (严格)"("Value"=w717) -> ()  [unwired: 2 in, 2 out]
                        n159 = One Button Dialog(message="Step is not zero or Start and Stop cannot both be zero ！") -> ()  [unwired: 1 in, 1 out]
                      }
                    }
                  }
                  frame True {
                    w720 = FALSE ("Repeat")
                    n160 = One Button Dialog(message="Value out of scan range!") -> ()  [unwired: 1 in, 1 out]
                    n161 = property on="Repeat" class="Bool (严格)"("Value"=w720) -> ()  [unwired: 2 in, 2 out]
                    n162 = property on="SetOK" class="Bool (严格)"("Value"=w720) -> ()  [unwired: 2 in, 2 out]
                  }
                }
              }
              frame #1 {
                n163 = case shown="假" w730 {
                  tunnel: w733 -> [w738 _]
                  tunnel: w732 -> [w736 _]
                  tunnel: w731 -> [w735 _]
                  tunnel: w729 -> [w737 _]
                  frame False {
                    n164 = property on="Test Type" class="RadioBtnsControl (严格)"() -> ("Value"=w734:enum32{"IV", "IT", "VT", "MOSFET"})  [unwired: 2 in, 2 out]
                    n165 = case shown="\"IV\", 默认" w734 {
                      tunnel: w738 -> [w773 w974 w1165 w1382]
                      tunnel: w737 -> [w763 w967 w1139 w1358]
                      tunnel: w736 -> [w764 w968 w1138 w1353]
                      tunnel: w735 -> [w762 w966 _ w1356]
                      frame "IT" {
                        w761 = TRUE
                        w772 = enum32{"Current", "Voltage"}."Voltage" ("Function (Current)")
                        w778 = sgl[] []
                        n166 = call <instrlib>:"Reset SMU.vi"("SMU B (No)"=w761, "SMU A (No)"=w761, "error in (no error)"=w762, "Node In"=w763, "VISA resource name"=w764) -> ("error out"=w758:errorcluster, "Node Out"=w759:string, "VISA resource name out"=w760:refnum<visa-resource-name>)  [unwired: 3 in, 1 out]
                        n167 = property on="Channel" class="Ring (严格)"() -> ("Value"=w739:u16)  [unwired: 2 in, 2 out]
                        n168 = property on="CompCurrIT" class="DigNum (严格)"() -> ("Value"=w752:sgl)  [unwired: 2 in, 2 out]
                        n169 = property on="CompUnit-IT" class="Ring (严格)"() -> ("Value"=w774:u16)  [unwired: 2 in, 2 out]
                        n170 = case shown="1, 默认" w774 {
                          tunnel: [1000000.0 ("Start") 1.0 ("Start") 1000.0 ("Start")] -> w775
                          frame 0 {
                          }
                          frame 1, Default {
                          }
                          frame 2 {
                          }
                        }
                        n171 = Divide(x=w752, y=w775) -> (x/y=w743:dbl)
                        n172 = property on="Voltage IT" class="DigNum (严格)"() -> ("Value"=w767:dbl)  [unwired: 2 in, 2 out]
                        n173 = property on="VoltageUnit IT" class="Ring (严格)"() -> ("Value"=w766:u16)  [unwired: 2 in, 2 out]
                        n174 = case shown="0" w766 {
                          tunnel: [1000.0 ("Start") 1.0 ("Start")] -> w768
                          frame 0 {
                          }
                          frame 1, Default {
                          }
                        }
                        n175 = call <instrlib>:"Source Function.vi"("Function (Current)"=w772, "error in (no error)"=w758, "Channel (Channel A)"=w739, "Node In"=w759, "VISA resource name"=w760) -> ("error out"=w771:errorcluster, "Node Out"=w770:string, "VISA resource name out"=w769:refnum<visa-resource-name>)  [unwired: 4 out]
                        n176 = Divide(x=w767, y=w768) -> (x/y=w765:dbl)
                        n177 = call <instrlib>:"Source Level.vi"("Level (0.000)"=w765, "Function (Current)"=w772, "error in (no error)"=w771, "Channel (Channel A)"=w739, "Node In"=w770, "VISA resource name"=w769) -> ("error out"=w744:errorcluster, "Node Out"=w745:string, "VISA resource name out"=w746:refnum<visa-resource-name>)  [unwired: 3 out]
                        n178 = call <instrlib>:"Source Limit.vi"("Limit (0.000)"=w743, "Function (Current)"=enum32{"Current", "Voltage"}."Current", "error in (no error)"=w744, "Channel (Channel A)"=w739, "Node In"=w745, "VISA resource name"=w746) -> ("error out"=w750:errorcluster, "Node Out"=w749:string, "VISA resource name out"=w748:refnum<visa-resource-name>)  [unwired: 3 out]
                        n179 = call <instrlib>:"Source Output Enable.vi"("Output (Off)"=TRUE, "error in (no error)"=w750, "Channel (Channel A)"=w739, "Node In"=w749, "VISA resource name"=w748) -> ("error out"=w740:errorcluster, "Node Out"=w742:string, "VISA resource name out"=w741:refnum<visa-resource-name>)  [unwired: 4 out]
                        n180 = property on="Tab Control" class="TabCtl (严格)"() -> ("Value"=w777:T5)  [unwired: 2 in, 2 out]
                        n181 = while {
                          tunnel: string[] ["  "] ("transposed array") -> [w803]
                          shift-right: [w804] -> _
                          shift-left: string[][] [] ("transposed array") -> [w850]
                          shift-right: [w843] -> _
                          shift-left: 0.0 ("Y") -> [w846]
                          shift-right: [w832] -> _
                          shift-left: w778 -> [w837]
                          shift-right: [w830] -> _
                          shift-left: w778 -> [w835]
                          shift-right: [w831] -> _
                          shift-left: w778 -> [w836]
                          tunnel: w773 -> [w819]
                          tunnel: w777 -> [w816]
                          tunnel: [w799] -> w756
                          tunnel: w765 -> [w798]
                          tunnel: [w797] -> w757
                          tunnel: [w796] -> w753
                          shift-right: [w795] -> _
                          shift-left: w743 -> [w795]
                          tunnel: w742 -> [w794]
                          tunnel: w741 -> [w793]
                          tunnel: w740 -> [w792]
                          i -> [w807]
                          stop <- w821 stop-if-true
                          w841 = 18 ("x")
                          n182 = property on="Channel" class="Ring (严格)"() -> ("Value"=w791:u16)  [unwired: 2 in, 2 out]
                          n183 = Equal?(x=0, y=w807) -> (x = y?=w806:bool)
                          n184 = Less?(x=w841, y=w807) -> (x < y?=w838:bool)
                          n185 = case shown="真" w838 {
                            tunnel: w807 -> [_ w937]
                            tunnel: w841 -> [_ w936]
                            tunnel: [0 w934] -> w839
                            frame False {
                            }
                            frame True {
                              n186 = Subtract(x=w937, y=w936) -> (x-y=w935:i32)
                              n187 = Increment(x=w935) -> (x+1=w934:i32)
                            }
                          }
                          n188 = call <instrlib>:"Measure.vi"("Function (Current)"=T14."Current", "error in (no error)"=w792, "Channel (Channel A)"=w791, "Node In"=w794, "VISA resource name"=w793) -> ("error out"=w799:errorcluster, "Output"=w811:string, "Node Out"=w797:string, "VISA resource name out"=w796:refnum<visa-resource-name>)  [unwired: 2 in, 1 out]
                          n189 = call "已用时间"("Reset"=w806) -> ("Elapsed Time (s)"=w805:dbl)  [unwired: 11 in, 7 out]
                          n190 = Bundle By Name(cluster=T15 {"Row"=0, "Column"=0} ("Index Values"), "Row"=w839) -> (w815:T15)
                          n191 = Fract/Exp String To Number(string=w811) -> (number=w810:dbl)  [unwired: 3 in, 1 out]
                          n192 = case shown="\"Data\", 默认" w816 {
                            tunnel: w815 -> [w856 w857 w858 w859 w860 w861 w862 w863 w864 w865 w866 w867 w868 w869 w870 w871 w872 w873 w874 w875 w876]
                            frame "Data", Default {
                              n193 = property on="Sheet" class="Tbl (严格)"("Index Values"=w856) -> ()  [unwired: 2 in, 2 out]
                            }
                            frame "Append 1" {
                              n194 = property on="Sheet 2" class="Tbl (严格)"("Index Values"=w857) -> ()  [unwired: 2 in, 2 out]
                            }
                            frame "Append 2" {
                              n195 = property on="Sheet 3" class="Tbl (严格)"("Index Values"=w858) -> ()  [unwired: 2 in, 2 out]
                            }
                            frame "Append 3" {
                              n196 = property on="Sheet 4" class="Tbl (严格)"("Index Values"=w859) -> ()  [unwired: 2 in, 2 out]
                            }
                            frame "Append 4" {
                              n197 = property on="Sheet 5" class="Tbl (严格)"("Index Values"=w860) -> ()  [unwired: 2 in, 2 out]
                            }
                            frame "Append 5" {
                              n198 = property on="Sheet 6" class="Tbl (严格)"("Index Values"=w861) -> ()  [unwired: 2 in, 2 out]
                            }
                            frame "Append 6" {
                              n199 = property on="Sheet 7" class="Tbl (严格)"("Index Values"=w862) -> ()  [unwired: 2 in, 2 out]
                            }
                            frame "Append 7" {
                              n200 = property on="Sheet 8" class="Tbl (严格)"("Index Values"=w863) -> ()  [unwired: 2 in, 2 out]
                            }
                            frame "Append 8" {
                              n201 = property on="Sheet 9" class="Tbl (严格)"("Index Values"=w864) -> ()  [unwired: 2 in, 2 out]
                            }
                            frame "Append 9" {
                              n202 = property on="Sheet 10" class="Tbl (严格)"("Index Values"=w865) -> ()  [unwired: 2 in, 2 out]
                            }
                            frame "Append 10" {
                              n203 = property on="Sheet 11" class="Tbl (严格)"("Index Values"=w866) -> ()  [unwired: 2 in, 2 out]
                            }
                            frame "Append 11" {
                              n204 = property on="Sheet 12" class="Tbl (严格)"("Index Values"=w867) -> ()  [unwired: 2 in, 2 out]
                            }
                            frame "Append 12" {
                              n205 = property on="Sheet 13" class="Tbl (严格)"("Index Values"=w868) -> ()  [unwired: 2 in, 2 out]
                            }
                            frame "Append 13" {
                              n206 = property on="Sheet 14" class="Tbl (严格)"("Index Values"=w869) -> ()  [unwired: 2 in, 2 out]
                            }
                            frame "Append 14" {
                              n207 = property on="Sheet 15" class="Tbl (严格)"("Index Values"=w870) -> ()  [unwired: 2 in, 2 out]
                            }
                            frame "Append 15" {
                              n208 = property on="Sheet 16" class="Tbl (严格)"("Index Values"=w871) -> ()  [unwired: 2 in, 2 out]
                            }
                            frame "Append 16" {
                              n209 = property on="Sheet 17" class="Tbl (严格)"("Index Values"=w872) -> ()  [unwired: 2 in, 2 out]
                            }
                            frame "Append 17" {
                              n210 = property on="Sheet 18" class="Tbl (严格)"("Index Values"=w873) -> ()  [unwired: 2 in, 2 out]
                            }
                            frame "Append 18" {
                              n211 = property on="Sheet 19" class="Tbl (严格)"("Index Values"=w874) -> ()  [unwired: 2 in, 2 out]
                            }
                            frame "Append 19" {
                              n212 = property on="Sheet 20" class="Tbl (严格)"("Index Values"=w875) -> ()  [unwired: 2 in, 2 out]
                            }
                            frame "Append 20" {
                              n213 = property on="Sheet 21" class="Tbl (严格)"("Index Values"=w876) -> ()  [unwired: 2 in, 2 out]
                            }
                          }
                          n214 = global read "Global 1.vi" "Timeout (10000 ms)"() -> (w848:i32)
                          n215 = Number To Exponential String(number=w810) -> (E-format string=w854:string)  [unwired: 3 in]
                          n216 = Number To Exponential String(number=w805) -> (E-format string=w855:string)  [unwired: 3 in]
                          n217 = Divide(x=w798, y=w810) -> (x/y=w845:dbl)
                          n218 = Build Array (concatenate)(w837, w810) -> (w832:dbl[])
                          n219 = Build Array (concatenate)(w836, w805) -> (w831:dbl[])
                          n220 = Replace Array Subset(array=w803, new element=w855) -> (w853:string[])  [unwired: 1 in]
                          n221 = Replace Array Subset(array=w803, new element=w854) -> (w852:string[])  [unwired: 1 in]
                          n222 = Build Array (concatenate)(w835, 0.0 ("Y")) -> (w830:dbl[])
                          n223 = property on="XYConvert" class="Bool (严格)"() -> ("Value"=w833:bool)  [unwired: 2 in, 2 out]
                          n224 = Add(x=w846, y=w845) -> (x+y=w843:dbl)
                          n225 = Less Than 0?(x=w848) -> (x < 0?=w847:bool)
                          n226 = Increment(x=w807) -> (x+1=w844:i32)
                          n227 = Unbundle By Name(w799) -> ("status"=w820:bool)
                          n228 = Or(x=w847, y=FALSE) -> (x .or. y?=w822:bool)
                          n229 = Divide(x=w843, y=w844) -> (x/y=w842:dbl)
                          "RES 2" <- w842
                          n230 = Or(x=w820, y=w822) -> (x .or. y?=w821:bool)
                          n231 = Number To Exponential String(number=w842) -> (E-format string=w802:string)  [unwired: 3 in]
                          n232 = case shown="真" w833 {
                            tunnel: w832 -> [w927 w931]
                            tunnel: w831 -> [w926 w932]
                            tunnel: w830 -> [w925 w930]
                            tunnel: [w927 w932] -> w823
                            tunnel: [w926 w931] -> w814
                            tunnel: [w925 w930] -> w813
                            tunnel: [w924 w928] -> w829
                            tunnel: [w923 w929] -> w828
                            tunnel: "AI" ("X Scale.Name Label.Text") -> [w924 w929]
                            tunnel: "t" ("X Scale.Name Label.Text") -> [w923 w928]
                            frame False {
                            }
                            frame True {
                            }
                          }
                          n233 = Replace Array Subset(array=w803, new element=w802) -> (w801:string[])  [unwired: 1 in]
                          n234 = Build Array(w853, w852, w801) -> (w851:string[][])
                          n235 = Transpose 2D Array(2D array=w851) -> (transposed array=w849:string[][])
                          n236 = case shown="真" w820 {
                            frame False {
                            }
                            frame True {
                              n237 = One Button Dialog(message="源表通讯异常") -> (true=w921:bool)  [unwired: 1 in]
                              n238 = case shown="真" w921 {
                                frame False {
                                }
                                frame True {
                                n239 = invoke class="VI" method="FP.Close"() -> ()  [unwired: 3 in, 3 out]
                                }
                              }
                            }
                          }
                          n240 = Build Array (concatenate)(w850, w849) -> (w804:string[][])
                          n241 = property on="Chart" class="XYGraph (严格)"("XScale.NameLbl.Text"=w829, "YScale.NameLbl.Text"=w828) -> ()  [unwired: 2 in, 2 out]
                          n242 = case shown="假" w819 {
                            tunnel: w804 -> [w898 w900]
                            tunnel: w816 -> [_ w899]
                            frame False {
                              n243 = local write "Sheet"(w898) -> ()
                            }
                            frame True {
                              n244 = case shown="\"Append 20\"" w899 {
                                tunnel: w900 -> [_ w901 w902 w903 w904 w905 w906 w907 w908 w909 w910 w911 w912 w913 w914 w915 w916 w917 w918 w919 w920]
                                frame "Data", Default {
                                }
                                frame "Append 1" {
                                n245 = property on="Sheet 2" class="Tbl (严格)"("Value"=w901) -> ()  [unwired: 2 in, 2 out]
                                }
                                frame "Append 2" {
                                n246 = property on="Sheet 3" class="Tbl (严格)"("Value"=w902) -> ()  [unwired: 2 in, 2 out]
                                }
                                frame "Append 3" {
                                n247 = property on="Sheet 4" class="Tbl (严格)"("Value"=w903) -> ()  [unwired: 2 in, 2 out]
                                }
                                frame "Append 4" {
                                n248 = property on="Sheet 5" class="Tbl (严格)"("Value"=w904) -> ()  [unwired: 2 in, 2 out]
                                }
                                frame "Append 5" {
                                n249 = property on="Sheet 6" class="Tbl (严格)"("Value"=w905) -> ()  [unwired: 2 in, 2 out]
                                }
                                frame "Append 6" {
                                n250 = property on="Sheet 7" class="Tbl (严格)"("Value"=w906) -> ()  [unwired: 2 in, 2 out]
                                }
                                frame "Append 7" {
                                n251 = property on="Sheet 8" class="Tbl (严格)"("Value"=w907) -> ()  [unwired: 2 in, 2 out]
                                }
                                frame "Append 8" {
                                n252 = property on="Sheet 9" class="Tbl (严格)"("Value"=w908) -> ()  [unwired: 2 in, 2 out]
                                }
                                frame "Append 9" {
                                n253 = property on="Sheet 10" class="Tbl (严格)"("Value"=w909) -> ()  [unwired: 2 in, 2 out]
                                }
                                frame "Append 10" {
                                n254 = property on="Sheet 11" class="Tbl (严格)"("Value"=w910) -> ()  [unwired: 2 in, 2 out]
                                }
                                frame "Append 11" {
                                n255 = property on="Sheet 12" class="Tbl (严格)"("Value"=w911) -> ()  [unwired: 2 in, 2 out]
                                }
                                frame "Append 12" {
                                n256 = property on="Sheet 13" class="Tbl (严格)"("Value"=w912) -> ()  [unwired: 2 in, 2 out]
                                }
                                frame "Append 13" {
                                n257 = property on="Sheet 14" class="Tbl (严格)"("Value"=w913) -> ()  [unwired: 2 in, 2 out]
                                }
                                frame "Append 14" {
                                n258 = property on="Sheet 15" class="Tbl (严格)"("Value"=w914) -> ()  [unwired: 2 in, 2 out]
                                }
                                frame "Append 15" {
                                n259 = property on="Sheet 16" class="Tbl (严格)"("Value"=w915) -> ()  [unwired: 2 in, 2 out]
                                }
                                frame "Append 16" {
                                n260 = property on="Sheet 17" class="Tbl (严格)"("Value"=w916) -> ()  [unwired: 2 in, 2 out]
                                }
                                frame "Append 17" {
                                n261 = property on="Sheet 18" class="Tbl (严格)"("Value"=w917) -> ()  [unwired: 2 in, 2 out]
                                }
                                frame "Append 18" {
                                n262 = property on="Sheet 19" class="Tbl (严格)"("Value"=w918) -> ()  [unwired: 2 in, 2 out]
                                }
                                frame "Append 19" {
                                n263 = property on="Sheet 20" class="Tbl (严格)"("Value"=w919) -> ()  [unwired: 2 in, 2 out]
                                }
                                frame "Append 20" {
                                n264 = property on="Sheet 21" class="Tbl (严格)"("Value"=w920) -> ()  [unwired: 2 in, 2 out]
                                }
                              }
                            }
                          }
                          n265 = Array Max & Min(array=w823) -> (max value=w825:dbl, min value=w824:dbl)  [unwired: 2 out]
                          n266 = property on="Chart" class="XYGraph (严格)"("XScale.Maximum"=w825, "XScale.Minimum"=w824) -> ()  [unwired: 2 in, 2 out]
                          n267 = case shown="\"Data\", 默认" w816 {
                            tunnel: [0 ("disabled index (row)") 1 ("disabled index (row)") 2 ("disabled index (row)") 3 ("disabled index (row)") 4 ("disabled index (row)") 5 ("disabled index (row)") 6 ("disabled index (row)") 7 ("disabled index (row)") 8 ("disabled index (row)") 9 ("disabled index (row)") 10 ("disabled index (row)") 11 ("disabled index (row)") 12 ("disabled index (row)") 13 ("disabled index (row)") 14 ("disabled index (row)") 15 ("disabled index (row)") 16 ("disabled index (row)") 17 ("disabled index (row)") 18 ("disabled index (row)") 19 ("disabled index (row)") 20 ("disabled index (row)")] -> w817
                            frame "Data", Default {
                            }
                            frame "Append 1" {
                            }
                            frame "Append 2" {
                            }
                            frame "Append 3" {
                            }
                            frame "Append 4" {
                            }
                            frame "Append 5" {
                            }
                            frame "Append 6" {
                            }
                            frame "Append 7" {
                            }
                            frame "Append 8" {
                            }
                            frame "Append 9" {
                            }
                            frame "Append 10" {
                            }
                            frame "Append 11" {
                            }
                            frame "Append 12" {
                            }
                            frame "Append 13" {
                            }
                            frame "Append 14" {
                            }
                            frame "Append 15" {
                            }
                            frame "Append 16" {
                            }
                            frame "Append 17" {
                            }
                            frame "Append 18" {
                            }
                            frame "Append 19" {
                            }
                            frame "Append 20" {
                            }
                          }
                          n268 = Bundle(w823, w814) -> (w787:cluster{dbl[], dbl[]})  [unwired: 1 in]
                          n269 = Bundle(w813, w814) -> (w812:cluster{dbl[], dbl[]})  [unwired: 1 in]
                          n270 = Bundle(w823, w813) -> (w788:cluster{dbl[], dbl[]})  [unwired: 1 in]
                          n271 = property on="TempChart" class="Arr (严格)"() -> ("Value"=w818:cluster{sgl[], dbl[]}[])  [unwired: 2 in, 2 out]
                          n272 = Replace Array Subset(array=w818, new element=w787, index=w817) -> (w789:cluster{sgl[], dbl[]}[])
                          n273 = Build Array (concatenate)(w789, w788, w812) -> (w790:cluster{dbl[], dbl[]}[])
                          n274 = property on="XY图" class="XYGraph (严格)"("Value"=w787) -> ()  [unwired: 2 in, 2 out]
                          n275 = property on="TempChart" class="Arr (严格)"("Value"=w789) -> ()  [unwired: 2 in, 2 out]
                          n276 = property on="Chart" class="XYGraph (严格)"("Value"=w790) -> ()  [unwired: 2 in, 2 out]
                        }
                        n277 = property on="Chart" class="XYGraph (严格)"("Active Plot"=w777, "Plot.Visible?"=TRUE ("Plot.Visible")) -> ()  [unwired: 2 in, 2 out]
                        n278 = property on="Channel" class="Ring (严格)"() -> ("Value"=w754:u16)  [unwired: 2 in, 2 out]
                        n279 = call <instrlib>:"Source Output Enable.vi"("Output (Off)"=FALSE, "error in (no error)"=w756, "Channel (Channel A)"=w754, "Node In"=w757, "VISA resource name"=w753) -> ()  [unwired: 7 out]
                      }
                      frame "VT" {
                        w942 = enum32{"Current", "Voltage"}."Current" ("Function (Current)")
                        w965 = TRUE
                        w977 = sgl[] []
                        n280 = call <instrlib>:"Reset SMU.vi"("SMU B (No)"=w965, "SMU A (No)"=w965, "error in (no error)"=w966, "Node In"=w967, "VISA resource name"=w968) -> ("error out"=w962:errorcluster, "Node Out"=w963:string, "VISA resource name out"=w964:refnum<visa-resource-name>)  [unwired: 3 in, 1 out]
                        n281 = property on="Channel" class="Ring (严格)"() -> ("Value"=w944:u16)  [unwired: 2 in, 2 out]
                        n282 = property on="Compliance" class="DigNum (严格)"() -> ("Value"=w956:sgl)  [unwired: 2 in, 2 out]
                        n283 = property on="CompUnit VT" class="Ring (严格)"() -> ("Value"=w939:u16)  [unwired: 2 in, 2 out]
                        n284 = case shown="1, 默认" w939 {
                          tunnel: [1000.0 ("Start") 1.0 ("Start")] -> w938
                          frame 0 {
                          }
                          frame 1, Default {
                          }
                        }
                        n285 = Divide(x=w956, y=w938) -> (x/y=w948:dbl)
                        n286 = property on="Current VT" class="DigNum (严格)"() -> ("Value"=w970:dbl)  [unwired: 2 in, 2 out]
                        n287 = property on="CurrUnit VT" class="Ring (严格)"() -> ("Value"=w941:u16)  [unwired: 2 in, 2 out]
                        n288 = call <instrlib>:"Source Function.vi"("Function (Current)"=w942, "error in (no error)"=w962, "Channel (Channel A)"=w944, "Node In"=w963, "VISA resource name"=w964) -> ("error out"=w973:errorcluster, "Node Out"=w972:string, "VISA resource name out"=w971:refnum<visa-resource-name>)  [unwired: 4 out]
                        n289 = case shown="0" w941 {
                          tunnel: [1000000.0 ("Start") 1.0 ("Start") 1000.0 ("Start")] -> w940
                          frame 0 {
                          }
                          frame 1 {
                          }
                          frame 2, Default {
                          }
                        }
                        n290 = Divide(x=w970, y=w940) -> (x/y=w969:dbl)
                        n291 = call <instrlib>:"Source Level.vi"("Level (0.000)"=w969, "Function (Current)"=w942, "error in (no error)"=w973, "Channel (Channel A)"=w944, "Node In"=w972, "VISA resource name"=w971) -> ("error out"=w949:errorcluster, "Node Out"=w950:string, "VISA resource name out"=w951:refnum<visa-resource-name>)  [unwired: 3 out]
                        n292 = call <instrlib>:"Source Limit.vi"("Limit (0.000)"=w948, "Function (Current)"=enum32{"Current", "Voltage"}."Voltage", "error in (no error)"=w949, "Channel (Channel A)"=w944, "Node In"=w950, "VISA resource name"=w951) -> ("error out"=w955:errorcluster, "Node Out"=w954:string, "VISA resource name out"=w953:refnum<visa-resource-name>)  [unwired: 3 out]
                        n293 = call <instrlib>:"Source Output Enable.vi"("Output (Off)"=TRUE, "error in (no error)"=w955, "Channel (Channel A)"=w944, "Node In"=w954, "VISA resource name"=w953) -> ("error out"=w945:errorcluster, "Node Out"=w947:string, "VISA resource name out"=w946:refnum<visa-resource-name>)  [unwired: 4 out]
                        n294 = property on="Tab Control" class="TabCtl (严格)"() -> ("Value"=w976:T5)  [unwired: 2 in, 2 out]
                        n295 = while {
                          tunnel: string[] ["  "] ("transposed array") -> [w999]
                          shift-right: [w1000] -> _
                          shift-left: string[][] [] ("transposed array") -> [w1049]
                          shift-right: [w1042] -> _
                          shift-left: 0.0 ("Y") -> [w1045]
                          shift-right: [w1030] -> _
                          shift-left: w977 -> [w1036]
                          shift-right: [w1028] -> _
                          shift-left: w977 -> [w1034]
                          shift-right: [w1029] -> _
                          shift-left: w977 -> [w1035]
                          tunnel: w974 -> [w1017]
                          tunnel: w976 -> [w1013]
                          tunnel: [w996] -> w960
                          tunnel: w969 -> [w995]
                          tunnel: [w994] -> w961
                          tunnel: [w993] -> w957
                          shift-right: [w992] -> _
                          shift-left: w948 -> [w992]
                          tunnel: w947 -> [w991]
                          tunnel: w946 -> [w990]
                          tunnel: w945 -> [w989]
                          i -> [w1003]
                          stop <- w1019 stop-if-true
                          w1040 = 18 ("x")
                          n296 = property on="Channel" class="Ring (严格)"() -> ("Value"=w988:u16)  [unwired: 2 in, 2 out]
                          n297 = Equal?(x=0, y=w1003) -> (x = y?=w1002:bool)
                          n298 = Less?(x=w1040, y=w1003) -> (x < y?=w1037:bool)
                          n299 = case shown="真" w1037 {
                            tunnel: w1003 -> [_ w1136]
                            tunnel: w1040 -> [_ w1135]
                            tunnel: [0 w1133] -> w1038
                            frame False {
                            }
                            frame True {
                              n300 = Subtract(x=w1136, y=w1135) -> (x-y=w1134:i32)
                              n301 = Increment(x=w1134) -> (x+1=w1133:i32)
                            }
                          }
                          n302 = call <instrlib>:"Measure.vi"("Function (Current)"=enum32{"Current", "Voltage"}."Voltage", "error in (no error)"=w989, "Channel (Channel A)"=w988, "Node In"=w991, "VISA resource name"=w990) -> ("error out"=w996:errorcluster, "Output"=w1007:string, "Node Out"=w994:string, "VISA resource name out"=w993:refnum<visa-resource-name>)  [unwired: 2 in, 1 out]
                          n303 = call "已用时间2"("Reset"=w1002) -> ("Elapsed Time (s)"=w1001:dbl)  [unwired: 11 in, 7 out]
                          n304 = Bundle By Name(cluster=T15 {"Row"=0, "Column"=0} ("Index Values"), "Row"=w1038) -> (w1012:T15)
                          n305 = Fract/Exp String To Number(string=w1007) -> (number=w1006:dbl)  [unwired: 3 in, 1 out]
                          n306 = case shown="\"Data\", 默认" w1013 {
                            tunnel: w1012 -> [w1055 w1056 w1057 w1058 w1059 w1060 w1061 w1062 w1063 w1064 w1065 w1066 w1067 w1068 w1069 w1070 w1071 w1072 w1073 w1074 w1075]
                            frame "Data", Default {
                              n307 = property on="Sheet" class="Tbl (严格)"("Index Values"=w1055) -> ()  [unwired: 2 in, 2 out]
                            }
                            frame "Append 1" {
                              n308 = property on="Sheet 2" class="Tbl (严格)"("Index Values"=w1056) -> ()  [unwired: 2 in, 2 out]
                            }
                            frame "Append 2" {
                              n309 = property on="Sheet 3" class="Tbl (严格)"("Index Values"=w1057) -> ()  [unwired: 2 in, 2 out]
                            }
                            frame "Append 3" {
                              n310 = property on="Sheet 4" class="Tbl (严格)"("Index Values"=w1058) -> ()  [unwired: 2 in, 2 out]
                            }
                            frame "Append 4" {
                              n311 = property on="Sheet 5" class="Tbl (严格)"("Index Values"=w1059) -> ()  [unwired: 2 in, 2 out]
                            }
                            frame "Append 5" {
                              n312 = property on="Sheet 6" class="Tbl (严格)"("Index Values"=w1060) -> ()  [unwired: 2 in, 2 out]
                            }
                            frame "Append 6" {
                              n313 = property on="Sheet 7" class="Tbl (严格)"("Index Values"=w1061) -> ()  [unwired: 2 in, 2 out]
                            }
                            frame "Append 7" {
                              n314 = property on="Sheet 8" class="Tbl (严格)"("Index Values"=w1062) -> ()  [unwired: 2 in, 2 out]
                            }
                            frame "Append 8" {
                              n315 = property on="Sheet 9" class="Tbl (严格)"("Index Values"=w1063) -> ()  [unwired: 2 in, 2 out]
                            }
                            frame "Append 9" {
                              n316 = property on="Sheet 10" class="Tbl (严格)"("Index Values"=w1064) -> ()  [unwired: 2 in, 2 out]
                            }
                            frame "Append 10" {
                              n317 = property on="Sheet 11" class="Tbl (严格)"("Index Values"=w1065) -> ()  [unwired: 2 in, 2 out]
                            }
                            frame "Append 11" {
                              n318 = property on="Sheet 12" class="Tbl (严格)"("Index Values"=w1066) -> ()  [unwired: 2 in, 2 out]
                            }
                            frame "Append 12" {
                              n319 = property on="Sheet 13" class="Tbl (严格)"("Index Values"=w1067) -> ()  [unwired: 2 in, 2 out]
                            }
                            frame "Append 13" {
                              n320 = property on="Sheet 14" class="Tbl (严格)"("Index Values"=w1068) -> ()  [unwired: 2 in, 2 out]
                            }
                            frame "Append 14" {
                              n321 = property on="Sheet 15" class="Tbl (严格)"("Index Values"=w1069) -> ()  [unwired: 2 in, 2 out]
                            }
                            frame "Append 15" {
                              n322 = property on="Sheet 16" class="Tbl (严格)"("Index Values"=w1070) -> ()  [unwired: 2 in, 2 out]
                            }
                            frame "Append 16" {
                              n323 = property on="Sheet 17" class="Tbl (严格)"("Index Values"=w1071) -> ()  [unwired: 2 in, 2 out]
                            }
                            frame "Append 17" {
                              n324 = property on="Sheet 18" class="Tbl (严格)"("Index Values"=w1072) -> ()  [unwired: 2 in, 2 out]
                            }
                            frame "Append 18" {
                              n325 = property on="Sheet 19" class="Tbl (严格)"("Index Values"=w1073) -> ()  [unwired: 2 in, 2 out]
                            }
                            frame "Append 19" {
                              n326 = property on="Sheet 20" class="Tbl (严格)"("Index Values"=w1074) -> ()  [unwired: 2 in, 2 out]
                            }
                            frame "Append 20" {
                              n327 = property on="Sheet 21" class="Tbl (严格)"("Index Values"=w1075) -> ()  [unwired: 2 in, 2 out]
                            }
                          }
                          n328 = global read "Global 1.vi" "Timeout (10000 ms)"() -> (w1047:i32)
                          n329 = Number To Exponential String(number=w1006) -> (E-format string=w1053:string)  [unwired: 3 in]
                          n330 = Number To Exponential String(number=w1001) -> (E-format string=w1054:string)  [unwired: 3 in]
                          n331 = Divide(x=w995, y=w1006) -> (x/y=w1044:dbl)
                          n332 = Build Array (concatenate)(w1036, w1006) -> (w1030:dbl[])
                          n333 = Build Array (concatenate)(w1035, w1001) -> (w1029:dbl[])
                          n334 = Replace Array Subset(array=w999, new element=w1054) -> (w1052:string[])  [unwired: 1 in]
                          n335 = Replace Array Subset(array=w999, new element=w1053) -> (w1051:string[])  [unwired: 1 in]
                          n336 = Build Array (concatenate)(w1034, 0.0 ("Y")) -> (w1028:dbl[])
                          n337 = property on="XYConvert" class="Bool (严格)"() -> ("Value"=w1031:bool)  [unwired: 2 in, 2 out]
                          n338 = Add(x=w1045, y=w1044) -> (x+y=w1042:dbl)
                          n339 = Less Than 0?(x=w1047) -> (x < 0?=w1046:bool)
                          n340 = Increment(x=w1003) -> (x+1=w1043:i32)
                          n341 = Unbundle By Name(w996) -> ("status"=w1018:bool)
                          n342 = Or(x=w1046, y=FALSE) -> (x .or. y?=w1020:bool)
                          n343 = Divide(x=w1042, y=w1043) -> (x/y=w1041:dbl)
                          "RES 3" <- w1041
                          n344 = Or(x=w1018, y=w1020) -> (x .or. y?=w1019:bool)
                          n345 = Number To Exponential String(number=w1041) -> (E-format string=w998:string)  [unwired: 3 in]
                          n346 = case shown="真" w1031 {
                            tunnel: w1030 -> [w1126 w1130]
                            tunnel: w1029 -> [w1125 w1131]
                            tunnel: w1028 -> [w1124 w1129]
                            tunnel: [w1126 w1131] -> w1021
                            tunnel: [w1125 w1130] -> w1011
                            tunnel: [w1124 w1129] -> w1010
                            tunnel: [w1123 w1127] -> w1027
                            tunnel: [w1122 w1128] -> w1026
                            tunnel: "AV" ("X Scale.Name Label.Text") -> [w1123 w1128]
                            tunnel: "t" ("X Scale.Name Label.Text") -> [w1122 w1127]
                            frame False {
                            }
                            frame True {
                            }
                          }
                          n347 = Replace Array Subset(array=w999, new element=w998) -> (w997:string[])  [unwired: 1 in]
                          n348 = Build Array(w1052, w1051, w997) -> (w1050:string[][])
                          n349 = Transpose 2D Array(2D array=w1050) -> (transposed array=w1048:string[][])
                          n350 = case shown="真" w1018 {
                            frame False {
                            }
                            frame True {
                              n351 = One Button Dialog(message="源表通讯异常") -> (true=w1120:bool)  [unwired: 1 in]
                              n352 = case shown="真" w1120 {
                                frame False {
                                }
                                frame True {
                                n353 = invoke class="VI" method="FP.Close"() -> ()  [unwired: 3 in, 3 out]
                                }
                              }
                            }
                          }
                          n354 = Build Array (concatenate)(w1049, w1048) -> (w1000:string[][])
                          n355 = property on="Chart" class="XYGraph (严格)"("XScale.NameLbl.Text"=w1027, "YScale.NameLbl.Text"=w1026) -> ()  [unwired: 2 in, 2 out]
                          n356 = case shown="真" w1017 {
                            tunnel: w1000 -> [w1097 w1099]
                            tunnel: w1013 -> [_ w1098]
                            frame False {
                              n357 = local write "Sheet"(w1097) -> ()
                            }
                            frame True {
                              n358 = case shown="\"Append 20\"" w1098 {
                                tunnel: w1099 -> [_ w1100 w1101 w1102 w1103 w1104 w1105 w1106 w1107 w1108 w1109 w1110 w1111 w1112 w1113 w1114 w1115 w1116 w1117 w1118 w1119]
                                frame "Data", Default {
                                }
                                frame "Append 1" {
                                n359 = property on="Sheet 2" class="Tbl (严格)"("Value"=w1100) -> ()  [unwired: 2 in, 2 out]
                                }
                                frame "Append 2" {
                                n360 = property on="Sheet 3" class="Tbl (严格)"("Value"=w1101) -> ()  [unwired: 2 in, 2 out]
                                }
                                frame "Append 3" {
                                n361 = property on="Sheet 4" class="Tbl (严格)"("Value"=w1102) -> ()  [unwired: 2 in, 2 out]
                                }
                                frame "Append 4" {
                                n362 = property on="Sheet 5" class="Tbl (严格)"("Value"=w1103) -> ()  [unwired: 2 in, 2 out]
                                }
                                frame "Append 5" {
                                n363 = property on="Sheet 6" class="Tbl (严格)"("Value"=w1104) -> ()  [unwired: 2 in, 2 out]
                                }
                                frame "Append 6" {
                                n364 = property on="Sheet 7" class="Tbl (严格)"("Value"=w1105) -> ()  [unwired: 2 in, 2 out]
                                }
                                frame "Append 7" {
                                n365 = property on="Sheet 8" class="Tbl (严格)"("Value"=w1106) -> ()  [unwired: 2 in, 2 out]
                                }
                                frame "Append 8" {
                                n366 = property on="Sheet 9" class="Tbl (严格)"("Value"=w1107) -> ()  [unwired: 2 in, 2 out]
                                }
                                frame "Append 9" {
                                n367 = property on="Sheet 10" class="Tbl (严格)"("Value"=w1108) -> ()  [unwired: 2 in, 2 out]
                                }
                                frame "Append 10" {
                                n368 = property on="Sheet 11" class="Tbl (严格)"("Value"=w1109) -> ()  [unwired: 2 in, 2 out]
                                }
                                frame "Append 11" {
                                n369 = property on="Sheet 12" class="Tbl (严格)"("Value"=w1110) -> ()  [unwired: 2 in, 2 out]
                                }
                                frame "Append 12" {
                                n370 = property on="Sheet 13" class="Tbl (严格)"("Value"=w1111) -> ()  [unwired: 2 in, 2 out]
                                }
                                frame "Append 13" {
                                n371 = property on="Sheet 14" class="Tbl (严格)"("Value"=w1112) -> ()  [unwired: 2 in, 2 out]
                                }
                                frame "Append 14" {
                                n372 = property on="Sheet 15" class="Tbl (严格)"("Value"=w1113) -> ()  [unwired: 2 in, 2 out]
                                }
                                frame "Append 15" {
                                n373 = property on="Sheet 16" class="Tbl (严格)"("Value"=w1114) -> ()  [unwired: 2 in, 2 out]
                                }
                                frame "Append 16" {
                                n374 = property on="Sheet 17" class="Tbl (严格)"("Value"=w1115) -> ()  [unwired: 2 in, 2 out]
                                }
                                frame "Append 17" {
                                n375 = property on="Sheet 18" class="Tbl (严格)"("Value"=w1116) -> ()  [unwired: 2 in, 2 out]
                                }
                                frame "Append 18" {
                                n376 = property on="Sheet 19" class="Tbl (严格)"("Value"=w1117) -> ()  [unwired: 2 in, 2 out]
                                }
                                frame "Append 19" {
                                n377 = property on="Sheet 20" class="Tbl (严格)"("Value"=w1118) -> ()  [unwired: 2 in, 2 out]
                                }
                                frame "Append 20" {
                                n378 = property on="Sheet 21" class="Tbl (严格)"("Value"=w1119) -> ()  [unwired: 2 in, 2 out]
                                }
                              }
                            }
                          }
                          n379 = Array Max & Min(array=w1021) -> (max value=w1023:dbl, min value=w1022:dbl)  [unwired: 2 out]
                          n380 = property on="Chart" class="XYGraph (严格)"("XScale.Maximum"=w1023, "XScale.Minimum"=w1022) -> ()  [unwired: 2 in, 2 out]
                          n381 = case shown="\"Data\", 默认" w1013 {
                            tunnel: [0 ("disabled index (row)") 1 ("disabled index (row)") 2 ("disabled index (row)") 3 ("disabled index (row)") 4 ("disabled index (row)") 5 ("disabled index (row)") 6 ("disabled index (row)") 7 ("disabled index (row)") 8 ("disabled index (row)") 9 ("disabled index (row)") 10 ("disabled index (row)") 11 ("disabled index (row)") 12 ("disabled index (row)") 13 ("disabled index (row)") 14 ("disabled index (row)") 15 ("disabled index (row)") 16 ("disabled index (row)") 17 ("disabled index (row)") 18 ("disabled index (row)") 19 ("disabled index (row)") 20 ("disabled index (row)")] -> w1014
                            frame "Data", Default {
                            }
                            frame "Append 1" {
                            }
                            frame "Append 2" {
                            }
                            frame "Append 3" {
                            }
                            frame "Append 4" {
                            }
                            frame "Append 5" {
                            }
                            frame "Append 6" {
                            }
                            frame "Append 7" {
                            }
                            frame "Append 8" {
                            }
                            frame "Append 9" {
                            }
                            frame "Append 10" {
                            }
                            frame "Append 11" {
                            }
                            frame "Append 12" {
                            }
                            frame "Append 13" {
                            }
                            frame "Append 14" {
                            }
                            frame "Append 15" {
                            }
                            frame "Append 16" {
                            }
                            frame "Append 17" {
                            }
                            frame "Append 18" {
                            }
                            frame "Append 19" {
                            }
                            frame "Append 20" {
                            }
                          }
                          n382 = Bundle(w1021, w1011) -> (w986:cluster{dbl[], dbl[]})  [unwired: 1 in]
                          n383 = Bundle(w1010, w1011) -> (w1009:cluster{dbl[], dbl[]})  [unwired: 1 in]
                          n384 = Bundle(w1021, w1010) -> (w1032:cluster{dbl[], dbl[]})  [unwired: 1 in]
                          n385 = property on="TempChart" class="Arr (严格)"() -> ("Value"=w1016:cluster{sgl[], dbl[]}[])  [unwired: 2 in, 2 out]
                          n386 = Replace Array Subset(array=w1016, new element=w986, index=w1014) -> (w1015:cluster{sgl[], dbl[]}[])
                          n387 = Build Array (concatenate)(w1015, w1032, w1009) -> (w1008:cluster{dbl[], dbl[]}[])
                          n388 = property on="TempChart" class="Arr (严格)"("Value"=w1015) -> ()  [unwired: 2 in, 2 out]
                          n389 = property on="Chart" class="XYGraph (严格)"("Value"=w1008) -> ()  [unwired: 2 in, 2 out]
                          n390 = property on="XY图" class="XYGraph (严格)"("Value"=w986) -> ()  [unwired: 2 in, 2 out]
                        }
                        n391 = property on="Chart" class="XYGraph (严格)"("Active Plot"=w976, "Plot.Visible?"=TRUE ("Plot.Visible")) -> ()  [unwired: 2 in, 2 out]
                        n392 = property on="Channel" class="Ring (严格)"() -> ("Value"=w958:u16)  [unwired: 2 in, 2 out]
                        n393 = call <instrlib>:"Source Output Enable.vi"("Output (Off)"=FALSE, "error in (no error)"=w960, "Channel (Channel A)"=w958, "Node In"=w961, "VISA resource name"=w957) -> ()  [unwired: 7 out]
                      }
                      frame "IV", Default {
                        w1166 = sgl[] []
                        n394 = property on="StoptUnit" class="Ring (严格)"() -> ("Value"=w1152:u16)  [unwired: 2 in, 2 out]
                        n395 = property on="Step" class="DigNum (严格)"() -> ("Value"=w1154:dbl)  [unwired: 2 in, 2 out]
                        n396 = property on="StartUnit" class="Ring (严格)"() -> ("Value"=w1150:u16)  [unwired: 2 in, 2 out]
                        n397 = property on="Stop" class="DigNum (严格)"() -> ("Value"=w1151:dbl)  [unwired: 2 in, 2 out]
                        n398 = property on="Start" class="DigNum (严格)"() -> ("Value"=w1149:dbl)  [unwired: 2 in, 2 out]
                        n399 = property on="Compliance" class="DigNum (严格)"() -> ("Value"=w1155:sgl)  [unwired: 2 in, 2 out]
                        n400 = case shown="1, 默认" w1150 {
                          tunnel: [1000.0 ("Start") 1.0 ("Start")] -> w1140
                          frame 0 {
                          }
                          frame 1, Default {
                          }
                        }
                        n401 = property on="StepUnit" class="Ring (严格)"() -> ("Value"=w1153:u16)  [unwired: 2 in, 2 out]
                        n402 = case shown="1, 默认" w1153 {
                          tunnel: [1000.0 ("Start") 1.0 ("Start")] -> w1144
                          frame 0 {
                          }
                          frame 1, Default {
                          }
                        }
                        n403 = case shown="1, 默认" w1152 {
                          tunnel: [1000.0 ("Start") 1.0 ("Start")] -> w1142
                          frame 0 {
                          }
                          frame 1, Default {
                          }
                        }
                        n404 = property on="CompliancetUnit" class="Ring (严格)"() -> ("Value"=w1145:u16)  [unwired: 2 in, 2 out]
                        n405 = case shown="2, 默认" w1145 {
                          tunnel: [1000000.0 ("Start") 1000.0 ("Start") 1.0 ("Start")] -> w1146
                          frame 0 {
                          }
                          frame 1 {
                          }
                          frame 2, Default {
                          }
                        }
                        n406 = Divide(x=w1149, y=w1140) -> (x/y=w1141:dbl)
                        n407 = Divide(x=w1151, y=w1142) -> (x/y=w1143:dbl)
                        n408 = Divide(x=w1154, y=w1144) -> (x/y=w1148:dbl)
                        n409 = Divide(x=w1155, y=w1146) -> (x/y=w1158:dbl)
                        n410 = property on="Channel" class="Ring (严格)"() -> ("Value"=w1137:u16)  [unwired: 2 in, 2 out]
                        n411 = call "Keithley Sample Number.vi"("Step"=w1148, "Stop"=w1143, "Start"=w1141) -> ("Array"=w1157:dbl[], "pointnumber"=w1147:dbl)  [unwired: 7 in]
                        n412 = property on="DataPoints" class="DigNum (严格)"("Value"=w1147) -> ()  [unwired: 2 in, 2 out]
                        n413 = Decrement(x=w1147) -> (x-1=w1159:dbl)
                        n414 = call <instrlib>:"Source Function.vi"("Function (Current)"=enum32{"Current", "Voltage"}."Voltage", "Channel (Channel A)"=w1137, "Node In"=w1139, "VISA resource name"=w1138) -> ("error out"=w1160:errorcluster, "Node Out"=w1162:string, "VISA resource name out"=w1161:refnum<visa-resource-name>)  [unwired: 1 in, 4 out]
                        n415 = property on="Tab Control" class="TabCtl (严格)"() -> ("Value"=w1164:T5)  [unwired: 2 in, 2 out]
                        n416 = while {
                          tunnel: w1158 -> [w1208]
                          shift-right: [w1205] -> _
                          shift-left: w1161 -> [w1209]
                          shift-right: [w1206] -> _
                          shift-left: w1160 -> [w1207]
                          tunnel: w1157 -> [w1182] mode=indexing
                          tunnel: string[] ["  "] ("transposed array") -> [w1262]
                          shift-right: [w1248] -> _
                          shift-left: string[][] [] ("transposed array") -> [w1257]
                          tunnel: w1159 -> [w1204]
                          shift-right: [w1250] -> _
                          shift-left: 0.0 ("Y") -> [w1253]
                          shift-right: [w1232] -> _
                          shift-left: w1166 -> [w1238]
                          shift-right: [w1230] -> _
                          shift-left: w1166 -> [w1236]
                          shift-right: [w1231] -> _
                          shift-left: w1166 -> [w1237]
                          tunnel: w1165 -> [w1219]
                          tunnel: w1164 -> [w1215]
                          tunnel: w1162 -> [w1210]
                          tunnel: [w1180] -> _
                          i -> [w1203]
                          stop <- w1221 stop-if-true
                          w1197 = enum32{"Current", "Voltage"}."Voltage" ("Function (Current)")
                          w1242 = 18 ("x")
                          n417 = property on="Channel" class="Ring (严格)"() -> ("Value"=w1181:u16)  [unwired: 2 in, 2 out]
                          n418 = Less?(x=w1242, y=w1203) -> (x < y?=w1239:bool)
                          n419 = case shown="真" w1239 {
                            tunnel: w1203 -> [_ w1345]
                            tunnel: w1242 -> [_ w1344]
                            tunnel: [0 w1342] -> w1240
                            frame False {
                            }
                            frame True {
                              n420 = Subtract(x=w1345, y=w1344) -> (x-y=w1343:i32)
                              n421 = Increment(x=w1343) -> (x+1=w1342:i32)
                            }
                          }
                          n422 = call <instrlib>:"Source Function.vi"("Function (Current)"=w1197, "error in (no error)"=w1207, "Channel (Channel A)"=w1181, "Node In"=w1210, "VISA resource name"=w1209) -> ("error out"=w1198:errorcluster, "Node Out"=w1199:string, "VISA resource name out"=w1200:refnum<visa-resource-name>)  [unwired: 4 out]
                          n423 = call <instrlib>:"Source Level.vi"("Level (0.000)"=w1182, "Function (Current)"=w1197, "error in (no error)"=w1198, "Channel (Channel A)"=w1181, "Node In"=w1199, "VISA resource name"=w1200) -> ("error out"=w1195:errorcluster, "Node Out"=w1194:string, "VISA resource name out"=w1196:refnum<visa-resource-name>)  [unwired: 3 out]
                          n424 = Bundle By Name(cluster=T15 {"Row"=0, "Column"=0} ("Index Values"), "Row"=w1240) -> (w1214:T15)
                          n425 = call <instrlib>:"Source Limit.vi"("Limit (0.000)"=w1208, "Function (Current)"=enum32{"Current", "Voltage"}."Current", "error in (no error)"=w1195, "Node In"=w1194, "VISA resource name"=w1196) -> ("error out"=w1192:errorcluster, "Node Out"=w1191:string, "VISA resource name out"=w1190:refnum<visa-resource-name>)  [unwired: 1 in, 3 out]
                          n426 = call <instrlib>:"Source Output Enable.vi"("Output (Off)"=TRUE, "error in (no error)"=w1192, "Node In"=w1191, "VISA resource name"=w1190) -> ("error out"=w1188:errorcluster, "Node Out"=w1187:string, "VISA resource name out"=w1189:refnum<visa-resource-name>)  [unwired: 1 in, 4 out]
                          n427 = Less Or Equal?(x=w1204, y=w1203) -> (x <= y?=w1202:bool)
                          n428 = case shown="\"Data\", 默认" w1215 {
                            tunnel: w1214 -> [w1264 w1265 w1266 w1267 w1268 w1269 w1270 w1271 w1272 w1273 w1274 w1275 w1276 w1277 w1278 w1279 w1280 w1281 w1282 w1283 w1284]
                            frame "Data", Default {
                              n429 = property on="Sheet" class="Tbl (严格)"("Index Values"=w1264) -> ()  [unwired: 2 in, 2 out]
                            }
                            frame "Append 1" {
                              n430 = property on="Sheet 2" class="Tbl (严格)"("Index Values"=w1265) -> ()  [unwired: 2 in, 2 out]
                            }
                            frame "Append 2" {
                              n431 = property on="Sheet 3" class="Tbl (严格)"("Index Values"=w1266) -> ()  [unwired: 2 in, 2 out]
                            }
                            frame "Append 3" {
                              n432 = property on="Sheet 4" class="Tbl (严格)"("Index Values"=w1267) -> ()  [unwired: 2 in, 2 out]
                            }
                            frame "Append 4" {
                              n433 = property on="Sheet 5" class="Tbl (严格)"("Index Values"=w1268) -> ()  [unwired: 2 in, 2 out]
                            }
                            frame "Append 5" {
                              n434 = property on="Sheet 6" class="Tbl (严格)"("Index Values"=w1269) -> ()  [unwired: 2 in, 2 out]
                            }
                            frame "Append 6" {
                              n435 = property on="Sheet 7" class="Tbl (严格)"("Index Values"=w1270) -> ()  [unwired: 2 in, 2 out]
                            }
                            frame "Append 7" {
                              n436 = property on="Sheet 8" class="Tbl (严格)"("Index Values"=w1271) -> ()  [unwired: 2 in, 2 out]
                            }
                            frame "Append 8" {
                              n437 = property on="Sheet 9" class="Tbl (严格)"("Index Values"=w1272) -> ()  [unwired: 2 in, 2 out]
                            }
                            frame "Append 9" {
                              n438 = property on="Sheet 10" class="Tbl (严格)"("Index Values"=w1273) -> ()  [unwired: 2 in, 2 out]
                            }
                            frame "Append 10" {
                              n439 = property on="Sheet 11" class="Tbl (严格)"("Index Values"=w1274) -> ()  [unwired: 2 in, 2 out]
                            }
                            frame "Append 11" {
                              n440 = property on="Sheet 12" class="Tbl (严格)"("Index Values"=w1275) -> ()  [unwired: 2 in, 2 out]
                            }
                            frame "Append 12" {
                              n441 = property on="Sheet 13" class="Tbl (严格)"("Index Values"=w1276) -> ()  [unwired: 2 in, 2 out]
                            }
                            frame "Append 13" {
                              n442 = property on="Sheet 14" class="Tbl (严格)"("Index Values"=w1277) -> ()  [unwired: 2 in, 2 out]
                            }
                            frame "Append 14" {
                              n443 = property on="Sheet 15" class="Tbl (严格)"("Index Values"=w1278) -> ()  [unwired: 2 in, 2 out]
                            }
                            frame "Append 15" {
                              n444 = property on="Sheet 16" class="Tbl (严格)"("Index Values"=w1279) -> ()  [unwired: 2 in, 2 out]
                            }
                            frame "Append 16" {
                              n445 = property on="Sheet 17" class="Tbl (严格)"("Index Values"=w1280) -> ()  [unwired: 2 in, 2 out]
                            }
                            frame "Append 17" {
                              n446 = property on="Sheet 18" class="Tbl (严格)"("Index Values"=w1281) -> ()  [unwired: 2 in, 2 out]
                            }
                            frame "Append 18" {
                              n447 = property on="Sheet 19" class="Tbl (严格)"("Index Values"=w1282) -> ()  [unwired: 2 in, 2 out]
                            }
                            frame "Append 19" {
                              n448 = property on="Sheet 20" class="Tbl (严格)"("Index Values"=w1283) -> ()  [unwired: 2 in, 2 out]
                            }
                            frame "Append 20" {
                              n449 = property on="Sheet 21" class="Tbl (严格)"("Index Values"=w1284) -> ()  [unwired: 2 in, 2 out]
                            }
                          }
                          n450 = call <instrlib>:"Measure.vi"("Function (Current)"=T14."Current", "error in (no error)"=w1188, "Node In"=w1187, "VISA resource name"=w1189) -> ("error out"=w1206:errorcluster, "Output"=w1184:string, "Node Out"=w1180:string, "VISA resource name out"=w1205:refnum<visa-resource-name>)  [unwired: 3 in, 1 out]
                          n451 = Fract/Exp String To Number(string=w1184) -> (number=w1183:dbl)  [unwired: 3 in, 1 out]
                          n452 = global read "Global 1.vi" "Timeout (10000 ms)"() -> (w1255:i32)
                          n453 = Number To Exponential String(number=w1183) -> (E-format string=w1261:string)  [unwired: 3 in]
                          n454 = Number To Exponential String(number=w1182) -> (E-format string=w1263:string)  [unwired: 3 in]
                          n455 = Divide(x=w1182, y=w1183) -> (x/y=w1252:dbl)
                          n456 = Build Array (concatenate)(w1238, w1183) -> (w1232:dbl[])
                          n457 = Build Array (concatenate)(w1237, w1182) -> (w1231:dbl[])
                          n458 = Replace Array Subset(array=w1262, new element=w1263) -> (w1260:string[])  [unwired: 1 in]
                          n459 = Replace Array Subset(array=w1262, new element=w1261) -> (w1259:string[])  [unwired: 1 in]
                          n460 = Build Array (concatenate)(w1236, 0.0 ("Y")) -> (w1230:dbl[])
                          n461 = Add(x=w1253, y=w1252) -> (x+y=w1250:dbl)
                          n462 = Less Than 0?(x=w1255) -> (x < 0?=w1254:bool)
                          n463 = Increment(x=w1203) -> (x+1=w1251:i32)
                          n464 = Unbundle By Name(w1206) -> ("status"=w1220:bool)
                          n465 = Or(x=w1254, y=w1202) -> (x .or. y?=w1222:bool)
                          n466 = property on="XYConvert" class="Bool (严格)"() -> ("Value"=w1233:bool)  [unwired: 2 in, 2 out]
                          n467 = Build Array(w1260, w1259, string[] ["  "] ("element")) -> (w1258:string[][])
                          n468 = Or(x=w1220, y=w1222) -> (x .or. y?=w1221:bool)
                          n469 = Divide(x=w1250, y=w1251) -> (x/y=w1249:dbl)
                          "RES" <- w1249
                          n470 = case shown="真" w1233 {
                            tunnel: w1232 -> [w1335 w1339]
                            tunnel: w1231 -> [w1334 w1340]
                            tunnel: w1230 -> [w1333 w1338]
                            tunnel: [w1335 w1340] -> w1223
                            tunnel: [w1334 w1339] -> w1213
                            tunnel: [w1333 w1338] -> w1212
                            tunnel: [w1332 w1336] -> w1229
                            tunnel: [w1331 w1337] -> w1228
                            tunnel: "AV" ("X Scale.Name Label.Text") -> [w1332 w1337]
                            tunnel: "AI" ("X Scale.Name Label.Text") -> [w1331 w1336]
                            frame False {
                            }
                            frame True {
                            }
                          }
                          n471 = Transpose 2D Array(2D array=w1258) -> (transposed array=w1256:string[][])
                          n472 = Number To Exponential String(number=w1249) -> (E-format string=w1243:string)  [unwired: 3 in]
                          n473 = case shown="真" w1220 {
                            frame False {
                            }
                            frame True {
                              n474 = One Button Dialog(message="源表通讯异常") -> (true=w1329:bool)  [unwired: 1 in]
                              n475 = case shown="真" w1329 {
                                frame False {
                                }
                                frame True {
                                n476 = invoke class="VI" method="FP.Close"() -> ()  [unwired: 3 in, 3 out]
                                }
                              }
                            }
                          }
                          n477 = Build Array (concatenate)(w1257, w1256) -> (w1248:string[][])
                          n478 = property on="Chart" class="XYGraph (严格)"("XScale.NameLbl.Text"=w1229, "YScale.NameLbl.Text"=w1228) -> ()  [unwired: 2 in, 2 out]
                          n479 = Replace Array Subset(array=w1248, new element=w1243, index (row)=0 ("disabled index (row)"), index (col)=2 ("disabled index (col)")) -> (w1246:string[][])
                          n480 = case shown="假" w1219 {
                            tunnel: w1246 -> [w1306 w1308]
                            tunnel: w1215 -> [_ w1307]
                            frame False {
                              n481 = local write "Sheet"(w1306) -> ()
                            }
                            frame True {
                              n482 = case shown="\"Data\", 默认" w1307 {
                                tunnel: w1308 -> [_ w1309 w1310 w1311 w1312 w1313 w1314 w1315 w1316 w1317 w1318 w1319 w1320 w1321 w1322 w1323 w1324 w1325 w1326 w1327 w1328]
                                frame "Data", Default {
                                }
                                frame "Append 1" {
                                n483 = property on="Sheet 2" class="Tbl (严格)"("Value"=w1309) -> ()  [unwired: 2 in, 2 out]
                                }
                                frame "Append 2" {
                                n484 = property on="Sheet 3" class="Tbl (严格)"("Value"=w1310) -> ()  [unwired: 2 in, 2 out]
                                }
                                frame "Append 3" {
                                n485 = property on="Sheet 4" class="Tbl (严格)"("Value"=w1311) -> ()  [unwired: 2 in, 2 out]
                                }
                                frame "Append 4" {
                                n486 = property on="Sheet 5" class="Tbl (严格)"("Value"=w1312) -> ()  [unwired: 2 in, 2 out]
                                }
                                frame "Append 5" {
                                n487 = property on="Sheet 6" class="Tbl (严格)"("Value"=w1313) -> ()  [unwired: 2 in, 2 out]
                                }
                                frame "Append 6" {
                                n488 = property on="Sheet 7" class="Tbl (严格)"("Value"=w1314) -> ()  [unwired: 2 in, 2 out]
                                }
                                frame "Append 7" {
                                n489 = property on="Sheet 8" class="Tbl (严格)"("Value"=w1315) -> ()  [unwired: 2 in, 2 out]
                                }
                                frame "Append 8" {
                                n490 = property on="Sheet 9" class="Tbl (严格)"("Value"=w1316) -> ()  [unwired: 2 in, 2 out]
                                }
                                frame "Append 9" {
                                n491 = property on="Sheet 10" class="Tbl (严格)"("Value"=w1317) -> ()  [unwired: 2 in, 2 out]
                                }
                                frame "Append 10" {
                                n492 = property on="Sheet 11" class="Tbl (严格)"("Value"=w1318) -> ()  [unwired: 2 in, 2 out]
                                }
                                frame "Append 11" {
                                n493 = property on="Sheet 12" class="Tbl (严格)"("Value"=w1319) -> ()  [unwired: 2 in, 2 out]
                                }
                                frame "Append 12" {
                                n494 = property on="Sheet 13" class="Tbl (严格)"("Value"=w1320) -> ()  [unwired: 2 in, 2 out]
                                }
                                frame "Append 13" {
                                n495 = property on="Sheet 14" class="Tbl (严格)"("Value"=w1321) -> ()  [unwired: 2 in, 2 out]
                                }
                                frame "Append 14" {
                                n496 = property on="Sheet 15" class="Tbl (严格)"("Value"=w1322) -> ()  [unwired: 2 in, 2 out]
                                }
                                frame "Append 15" {
                                n497 = property on="Sheet 16" class="Tbl (严格)"("Value"=w1323) -> ()  [unwired: 2 in, 2 out]
                                }
                                frame "Append 16" {
                                n498 = property on="Sheet 17" class="Tbl (严格)"("Value"=w1324) -> ()  [unwired: 2 in, 2 out]
                                }
                                frame "Append 17" {
                                n499 = property on="Sheet 18" class="Tbl (严格)"("Value"=w1325) -> ()  [unwired: 2 in, 2 out]
                                }
                                frame "Append 18" {
                                n500 = property on="Sheet 19" class="Tbl (严格)"("Value"=w1326) -> ()  [unwired: 2 in, 2 out]
                                }
                                frame "Append 19" {
                                n501 = property on="Sheet 20" class="Tbl (严格)"("Value"=w1327) -> ()  [unwired: 2 in, 2 out]
                                }
                                frame "Append 20" {
                                n502 = property on="Sheet 21" class="Tbl (严格)"("Value"=w1328) -> ()  [unwired: 2 in, 2 out]
                                }
                              }
                            }
                          }
                          n503 = Array Max & Min(array=w1223) -> (max value=w1225:dbl, min value=w1224:dbl)  [unwired: 2 out]
                          n504 = property on="Chart" class="XYGraph (严格)"("XScale.Maximum"=w1225, "XScale.Minimum"=w1224) -> ()  [unwired: 2 in, 2 out]
                          n505 = case shown="\"Append 2\"" w1215 {
                            tunnel: [0 ("disabled index (row)") 1 ("disabled index (row)") 2 ("disabled index (row)") 3 ("disabled index (row)") 4 ("disabled index (row)") 5 ("disabled index (row)") 6 ("disabled index (row)") 7 ("disabled index (row)") 8 ("disabled index (row)") 9 ("disabled index (row)") 10 ("disabled index (row)") 11 ("disabled index (row)") 12 ("disabled index (row)") 13 ("disabled index (row)") 14 ("disabled index (row)") 15 ("disabled index (row)") 16 ("disabled index (row)") 17 ("disabled index (row)") 18 ("disabled index (row)") 19 ("disabled index (row)") 20 ("disabled index (row)")] -> w1216
                            frame "Data", Default {
                            }
                            frame "Append 1" {
                            }
                            frame "Append 2" {
                            }
                            frame "Append 3" {
                            }
                            frame "Append 4" {
                            }
                            frame "Append 5" {
                            }
                            frame "Append 6" {
                            }
                            frame "Append 7" {
                            }
                            frame "Append 8" {
                            }
                            frame "Append 9" {
                            }
                            frame "Append 10" {
                            }
                            frame "Append 11" {
                            }
                            frame "Append 12" {
                            }
                            frame "Append 13" {
                            }
                            frame "Append 14" {
                            }
                            frame "Append 15" {
                            }
                            frame "Append 16" {
                            }
                            frame "Append 17" {
                            }
                            frame "Append 18" {
                            }
                            frame "Append 19" {
                            }
                            frame "Append 20" {
                            }
                          }
                          n506 = Bundle(w1223, w1213) -> (w1179:cluster{dbl[], dbl[]})  [unwired: 1 in]
                          n507 = Bundle(w1212, w1213) -> (w1211:cluster{dbl[], dbl[]})  [unwired: 1 in]
                          n508 = Bundle(w1223, w1212) -> (w1234:cluster{dbl[], dbl[]})  [unwired: 1 in]
                          n509 = property on="TempChart" class="Arr (严格)"() -> ("Value"=w1218:cluster{sgl[], dbl[]}[])  [unwired: 2 in, 2 out]
                          n510 = Replace Array Subset(array=w1218, new element=w1179, index=w1216) -> (w1217:cluster{sgl[], dbl[]}[])
                          n511 = Build Array (concatenate)(w1217, w1234, w1211) -> (w1201:cluster{dbl[], dbl[]}[])
                          n512 = property on="TempChart" class="Arr (严格)"("Value"=w1217) -> ()  [unwired: 2 in, 2 out]
                          n513 = property on="XY图" class="XYGraph (严格)"("Value"=w1179) -> ()  [unwired: 2 in, 2 out]
                          n514 = property on="Chart" class="XYGraph (严格)"("Value"=w1201) -> ()  [unwired: 2 in, 2 out]
                        }
                        n515 = property on="Chart" class="XYGraph (严格)"("Active Plot"=w1164, "Plot.Visible?"=TRUE ("Plot.Visible")) -> ()  [unwired: 2 in, 2 out]
                      }
                      frame "MOSFET" {
                        w1383 = sgl[] []
                        n516 = property on="StoptUnit" class="Ring (严格)"() -> ("Value"=w1371:u16)  [unwired: 2 in, 2 out]
                        n517 = property on="Gate Step" class="DigNum (严格)"() -> ("Value"=w1373:dbl)  [unwired: 2 in, 2 out]
                        n518 = property on="StartUnit" class="Ring (严格)"() -> ("Value"=w1369:u16)  [unwired: 2 in, 2 out]
                        n519 = property on="Gate Stop" class="DigNum (严格)"() -> ("Value"=w1370:dbl)  [unwired: 2 in, 2 out]
                        n520 = property on="Gate Start" class="DigNum (严格)"() -> ("Value"=w1368:dbl)  [unwired: 2 in, 2 out]
                        n521 = property on="Compliance" class="DigNum (严格)"() -> ("Value"=w1374:sgl)  [unwired: 2 in, 2 out]
                        n522 = case shown="1, 默认" w1369 {
                          tunnel: [1000.0 ("Start") 1.0 ("Start")] -> w1359
                          frame 0 {
                          }
                          frame 1, Default {
                          }
                        }
                        n523 = property on="StepUnit" class="Ring (严格)"() -> ("Value"=w1372:u16)  [unwired: 2 in, 2 out]
                        n524 = case shown="1, 默认" w1372 {
                          tunnel: [1000.0 ("Start") 1.0 ("Start")] -> w1363
                          frame 0 {
                          }
                          frame 1, Default {
                          }
                        }
                        n525 = case shown="1, 默认" w1371 {
                          tunnel: [1000.0 ("Start") 1.0 ("Start")] -> w1361
                          frame 0 {
                          }
                          frame 1, Default {
                          }
                        }
                        n526 = property on="CompliancetUnit" class="Ring (严格)"() -> ("Value"=w1364:u16)  [unwired: 2 in, 2 out]
                        n527 = case shown="2, 默认" w1364 {
                          tunnel: [1000000.0 ("Start") 1000.0 ("Start") 1.0 ("Start")] -> w1365
                          frame 0 {
                          }
                          frame 1 {
                          }
                          frame 2, Default {
                          }
                        }
                        n528 = Divide(x=w1368, y=w1359) -> (x/y=w1360:dbl)
                        n529 = Divide(x=w1370, y=w1361) -> (x/y=w1362:dbl)
                        n530 = Divide(x=w1373, y=w1363) -> (x/y=w1367:dbl)
                        n531 = Divide(x=w1374, y=w1365) -> (x/y=w1346:dbl)
                        n532 = property on="Channel" class="Ring (严格)"() -> ("Value"=w1351:u16)  [unwired: 2 in, 2 out]
                        n533 = call <instrlib>:"Node Format.vi"("error in"=w1356, "Node (0-64)"=1) -> ("error out"=w1354:errorcluster, "Formatted Node"=w1355:string)  [unwired: 8 in]
                        n534 = call "Keithley Sample Number.vi"("Step"=w1367, "Stop"=w1362, "Start"=w1360) -> ("Array"=w1348:dbl[], "pointnumber"=w1366:dbl)  [unwired: 7 in]
                        n535 = Subtract(x=1, y=w1351) -> (x-y=w1350:i32)
                        n536 = Decrement(x=w1366) -> (x-1=w1376:dbl)
                        n537 = call <instrlib>:"Source Function.vi"("error in (no error)"=w1354, "Channel (Channel A)"=w1350, "Node In"=w1355, "VISA resource name"=w1353) -> ("Node Out"=w1349:string)  [unwired: 1 in, 6 out]
                        n538 = call <instrlib>:"Source Function.vi"("Function (Current)"=enum32{"Current", "Voltage"}."Voltage", "error in (no error)"=w1356, "Channel (Channel A)"=w1351, "Node In"=w1358, "VISA resource name"=w1353) -> ("error out"=w1377:errorcluster, "Node Out"=w1379:string, "VISA resource name out"=w1378:refnum<visa-resource-name>)  [unwired: 4 out]
                        n539 = property on="Drain" class="DigNum (严格)"() -> ("Value"=w1347:dbl)  [unwired: 2 in, 2 out]
                        n540 = property on="Tab Control" class="TabCtl (严格)"() -> ("Value"=w1381:T5)  [unwired: 2 in, 2 out]
                        n541 = while {
                          shift-right: [w1437] -> _
                          shift-left: w1378 -> [w1409]
                          shift-right: [w1438] -> _
                          shift-left: w1377 -> [w1410]
                          tunnel: string[] ["  "] ("transposed array") -> [w1491]
                          shift-right: [w1477] -> _
                          shift-left: string[][] [] ("transposed array") -> [w1486]
                          tunnel: w1376 -> [w1408]
                          shift-right: [w1479] -> _
                          shift-left: 0.0 ("Y") -> [w1482]
                          shift-right: [w1461] -> _
                          shift-left: w1383 -> [w1467]
                          shift-right: [w1459] -> _
                          shift-left: w1383 -> [w1465]
                          shift-right: [w1460] -> _
                          shift-left: w1383 -> [w1466]
                          tunnel: w1382 -> [w1448]
                          tunnel: w1381 -> [w1444]
                          tunnel: w1379 -> [w1439]
                          tunnel: [w1416] -> _
                          tunnel: w1349 -> [w1411]
                          tunnel: w1348 -> [w1407] mode=indexing
                          tunnel: w1347 -> [w1406]
                          tunnel: w1346 -> [w1397]
                          i -> [w1436]
                          stop <- w1450 stop-if-true
                          w1398 = enum32{"Current", "Voltage"}."Voltage" ("Function (Current)")
                          w1405 = enum32{"Current", "Voltage"}."Voltage" ("Function (Current)")
                          w1471 = 18 ("x")
                          n542 = property on="Channel" class="Ring (严格)"() -> ("Value"=w1399:u16)  [unwired: 2 in, 2 out]
                          n543 = Less?(x=w1471, y=w1436) -> (x < y?=w1468:bool)
                          n544 = case shown="真" w1468 {
                            tunnel: w1436 -> [_ w1574]
                            tunnel: w1471 -> [_ w1573]
                            tunnel: [0 w1571] -> w1469
                            frame False {
                            }
                            frame True {
                              n545 = Subtract(x=w1574, y=w1573) -> (x-y=w1572:i32)
                              n546 = Increment(x=w1572) -> (x+1=w1571:i32)
                            }
                          }
                          n547 = Subtract(x=1, y=w1399) -> (x-y=w1400:i32)
                          n548 = call <instrlib>:"Source Function.vi"("Function (Current)"=w1405, "error in (no error)"=w1410, "Channel (Channel A)"=w1399, "Node In"=w1439, "VISA resource name"=w1409) -> ("error out"=w1431:errorcluster, "Node Out"=w1432:string, "VISA resource name out"=w1433:refnum<visa-resource-name>)  [unwired: 4 out]
                          n549 = call <instrlib>:"Source Level.vi"("Level (0.000)"=w1406, "Function (Current)"=w1405, "error in (no error)"=w1431, "Channel (Channel A)"=w1399, "Node In"=w1432, "VISA resource name"=w1433) -> ("error out"=w1429:errorcluster, "Node Out"=w1428:string, "VISA resource name out"=w1430:refnum<visa-resource-name>)  [unwired: 3 out]
                          n550 = call <instrlib>:"Source Function.vi"("Function (Current)"=w1398, "error in (no error)"=w1410, "Channel (Channel A)"=w1400, "Node In"=w1411, "VISA resource name"=w1409) -> ("error out"=w1413:errorcluster, "Node Out"=w1414:string, "VISA resource name out"=w1415:refnum<visa-resource-name>)  [unwired: 4 out]
                          n551 = Bundle By Name(cluster=T15 {"Row"=0, "Column"=0} ("Index Values"), "Row"=w1469) -> (w1443:T15)
                          n552 = call <instrlib>:"Source Limit.vi"("Limit (0.000)"=w1397, "Function (Current)"=enum32{"Current", "Voltage"}."Current", "error in (no error)"=w1429, "Node In"=w1428, "VISA resource name"=w1430) -> ("error out"=w1426:errorcluster, "Node Out"=w1425:string, "VISA resource name out"=w1424:refnum<visa-resource-name>)  [unwired: 1 in, 3 out]
                          n553 = call <instrlib>:"Source Level.vi"("Level (0.000)"=w1407, "Function (Current)"=w1398, "error in (no error)"=w1413, "Channel (Channel A)"=w1400, "Node In"=w1414, "VISA resource name"=w1415) -> ("error out"=w1402:errorcluster, "Node Out"=w1403:string, "VISA resource name out"=w1404:refnum<visa-resource-name>)  [unwired: 3 out]
                          n554 = call <instrlib>:"Source Output Enable.vi"("Output (Off)"=TRUE, "error in (no error)"=w1426, "Node In"=w1425, "VISA resource name"=w1424) -> ("error out"=w1422:errorcluster, "Node Out"=w1421:string, "VISA resource name out"=w1423:refnum<visa-resource-name>)  [unwired: 1 in, 4 out]
                          n555 = Less Or Equal?(x=w1408, y=w1436) -> (x <= y?=w1435:bool)
                          n556 = case shown="\"Data\", 默认" w1444 {
                            tunnel: w1443 -> [w1493 w1494 w1495 w1496 w1497 w1498 w1499 w1500 w1501 w1502 w1503 w1504 w1505 w1506 w1507 w1508 w1509 w1510 w1511 w1512 w1513]
                            frame "Data", Default {
                              n557 = property on="Sheet" class="Tbl (严格)"("Index Values"=w1493) -> ()  [unwired: 2 in, 2 out]
                            }
                            frame "Append 1" {
                              n558 = property on="Sheet 2" class="Tbl (严格)"("Index Values"=w1494) -> ()  [unwired: 2 in, 2 out]
                            }
                            frame "Append 2" {
                              n559 = property on="Sheet 3" class="Tbl (严格)"("Index Values"=w1495) -> ()  [unwired: 2 in, 2 out]
                            }
                            frame "Append 3" {
                              n560 = property on="Sheet 4" class="Tbl (严格)"("Index Values"=w1496) -> ()  [unwired: 2 in, 2 out]
                            }
                            frame "Append 4" {
                              n561 = property on="Sheet 5" class="Tbl (严格)"("Index Values"=w1497) -> ()  [unwired: 2 in, 2 out]
                            }
                            frame "Append 5" {
                              n562 = property on="Sheet 6" class="Tbl (严格)"("Index Values"=w1498) -> ()  [unwired: 2 in, 2 out]
                            }
                            frame "Append 6" {
                              n563 = property on="Sheet 7" class="Tbl (严格)"("Index Values"=w1499) -> ()  [unwired: 2 in, 2 out]
                            }
                            frame "Append 7" {
                              n564 = property on="Sheet 8" class="Tbl (严格)"("Index Values"=w1500) -> ()  [unwired: 2 in, 2 out]
                            }
                            frame "Append 8" {
                              n565 = property on="Sheet 9" class="Tbl (严格)"("Index Values"=w1501) -> ()  [unwired: 2 in, 2 out]
                            }
                            frame "Append 9" {
                              n566 = property on="Sheet 10" class="Tbl (严格)"("Index Values"=w1502) -> ()  [unwired: 2 in, 2 out]
                            }
                            frame "Append 10" {
                              n567 = property on="Sheet 11" class="Tbl (严格)"("Index Values"=w1503) -> ()  [unwired: 2 in, 2 out]
                            }
                            frame "Append 11" {
                              n568 = property on="Sheet 12" class="Tbl (严格)"("Index Values"=w1504) -> ()  [unwired: 2 in, 2 out]
                            }
                            frame "Append 12" {
                              n569 = property on="Sheet 13" class="Tbl (严格)"("Index Values"=w1505) -> ()  [unwired: 2 in, 2 out]
                            }
                            frame "Append 13" {
                              n570 = property on="Sheet 14" class="Tbl (严格)"("Index Values"=w1506) -> ()  [unwired: 2 in, 2 out]
                            }
                            frame "Append 14" {
                              n571 = property on="Sheet 15" class="Tbl (严格)"("Index Values"=w1507) -> ()  [unwired: 2 in, 2 out]
                            }
                            frame "Append 15" {
                              n572 = property on="Sheet 16" class="Tbl (严格)"("Index Values"=w1508) -> ()  [unwired: 2 in, 2 out]
                            }
                            frame "Append 16" {
                              n573 = property on="Sheet 17" class="Tbl (严格)"("Index Values"=w1509) -> ()  [unwired: 2 in, 2 out]
                            }
                            frame "Append 17" {
                              n574 = property on="Sheet 18" class="Tbl (严格)"("Index Values"=w1510) -> ()  [unwired: 2 in, 2 out]
                            }
                            frame "Append 18" {
                              n575 = property on="Sheet 19" class="Tbl (严格)"("Index Values"=w1511) -> ()  [unwired: 2 in, 2 out]
                            }
                            frame "Append 19" {
                              n576 = property on="Sheet 20" class="Tbl (严格)"("Index Values"=w1512) -> ()  [unwired: 2 in, 2 out]
                            }
                            frame "Append 20" {
                              n577 = property on="Sheet 21" class="Tbl (严格)"("Index Values"=w1513) -> ()  [unwired: 2 in, 2 out]
                            }
                          }
                          n578 = call <instrlib>:"Source Output Enable.vi"("Output (Off)"=TRUE, "error in (no error)"=w1402, "Node In"=w1403, "VISA resource name"=w1404) -> ()  [unwired: 1 in, 7 out]
                          n579 = call <instrlib>:"Measure.vi"("Function (Current)"=T14."Current", "error in (no error)"=w1422, "Node In"=w1421, "VISA resource name"=w1423) -> ("error out"=w1438:errorcluster, "Output"=w1418:string, "Node Out"=w1416:string, "VISA resource name out"=w1437:refnum<visa-resource-name>)  [unwired: 3 in, 1 out]
                          n580 = Fract/Exp String To Number(string=w1418) -> (number=w1417:dbl)  [unwired: 3 in, 1 out]
                          n581 = global read "Global 1.vi" "Timeout (10000 ms)"() -> (w1484:i32)
                          n582 = Number To Exponential String(number=w1417) -> (E-format string=w1490:string)  [unwired: 3 in]
                          n583 = Number To Exponential String(number=w1407) -> (E-format string=w1492:string)  [unwired: 3 in]
                          n584 = Divide(x=w1407, y=w1417) -> (x/y=w1481:dbl)
                          n585 = Build Array (concatenate)(w1467, w1417) -> (w1461:dbl[])
                          n586 = Build Array (concatenate)(w1466, w1407) -> (w1460:dbl[])
                          n587 = Replace Array Subset(array=w1491, new element=w1492) -> (w1489:string[])  [unwired: 1 in]
                          n588 = Replace Array Subset(array=w1491, new element=w1490) -> (w1488:string[])  [unwired: 1 in]
                          n589 = Build Array (concatenate)(w1465, 0.0 ("Y")) -> (w1459:dbl[])
                          n590 = Add(x=w1482, y=w1481) -> (x+y=w1479:dbl)
                          n591 = Less Than 0?(x=w1484) -> (x < 0?=w1483:bool)
                          n592 = Increment(x=w1436) -> (x+1=w1480:i32)
                          n593 = Unbundle By Name(w1438) -> ("status"=w1449:bool)
                          n594 = Or(x=w1483, y=w1435) -> (x .or. y?=w1451:bool)
                          n595 = property on="XYConvert" class="Bool (严格)"() -> ("Value"=w1462:bool)  [unwired: 2 in, 2 out]
                          n596 = Build Array(w1489, w1488, string[] ["  "] ("element")) -> (w1487:string[][])
                          n597 = Or(x=w1449, y=w1451) -> (x .or. y?=w1450:bool)
                          n598 = Divide(x=w1479, y=w1480) -> (x/y=w1478:dbl)
                          "RES 4" <- w1478
                          n599 = case shown="真" w1462 {
                            tunnel: w1461 -> [w1564 w1568]
                            tunnel: w1460 -> [w1563 w1569]
                            tunnel: w1459 -> [w1562 w1567]
                            tunnel: [w1564 w1569] -> w1452
                            tunnel: [w1563 w1568] -> w1442
                            tunnel: [w1562 w1567] -> w1441
                            tunnel: [w1561 w1565] -> w1458
                            tunnel: [w1560 w1566] -> w1457
                            tunnel: "Gate V" ("X Scale.Name Label.Text") -> [w1561 w1566]
                            tunnel: "Drain I" ("X Scale.Name Label.Text") -> [w1560 w1565]
                            frame False {
                            }
                            frame True {
                            }
                          }
                          n600 = Transpose 2D Array(2D array=w1487) -> (transposed array=w1485:string[][])
                          n601 = Number To Exponential String(number=w1478) -> (E-format string=w1472:string)  [unwired: 3 in]
                          n602 = case shown="真" w1449 {
                            frame False {
                            }
                            frame True {
                              n603 = One Button Dialog(message="源表通讯异常") -> (true=w1558:bool)  [unwired: 1 in]
                              n604 = case shown="真" w1558 {
                                frame False {
                                }
                                frame True {
                                n605 = invoke class="VI" method="FP.Close"() -> ()  [unwired: 3 in, 3 out]
                                }
                              }
                            }
                          }
                          n606 = Build Array (concatenate)(w1486, w1485) -> (w1477:string[][])
                          n607 = property on="Chart" class="XYGraph (严格)"("XScale.NameLbl.Text"=w1458, "YScale.NameLbl.Text"=w1457) -> ()  [unwired: 2 in, 2 out]
                          n608 = Replace Array Subset(array=w1477, new element=w1472, index (row)=0 ("disabled index (row)"), index (col)=2 ("disabled index (col)")) -> (w1475:string[][])
                          n609 = case shown="假" w1448 {
                            tunnel: w1475 -> [w1535 w1537]
                            tunnel: w1444 -> [_ w1536]
                            frame False {
                              n610 = local write "Sheet"(w1535) -> ()
                            }
                            frame True {
                              n611 = case shown="\"Data\", 默认" w1536 {
                                tunnel: w1537 -> [_ w1538 w1539 w1540 w1541 w1542 w1543 w1544 w1545 w1546 w1547 w1548 w1549 w1550 w1551 w1552 w1553 w1554 w1555 w1556 w1557]
                                frame "Data", Default {
                                }
                                frame "Append 1" {
                                n612 = property on="Sheet 2" class="Tbl (严格)"("Value"=w1538) -> ()  [unwired: 2 in, 2 out]
                                }
                                frame "Append 2" {
                                n613 = property on="Sheet 3" class="Tbl (严格)"("Value"=w1539) -> ()  [unwired: 2 in, 2 out]
                                }
                                frame "Append 3" {
                                n614 = property on="Sheet 4" class="Tbl (严格)"("Value"=w1540) -> ()  [unwired: 2 in, 2 out]
                                }
                                frame "Append 4" {
                                n615 = property on="Sheet 5" class="Tbl (严格)"("Value"=w1541) -> ()  [unwired: 2 in, 2 out]
                                }
                                frame "Append 5" {
                                n616 = property on="Sheet 6" class="Tbl (严格)"("Value"=w1542) -> ()  [unwired: 2 in, 2 out]
                                }
                                frame "Append 6" {
                                n617 = property on="Sheet 7" class="Tbl (严格)"("Value"=w1543) -> ()  [unwired: 2 in, 2 out]
                                }
                                frame "Append 7" {
                                n618 = property on="Sheet 8" class="Tbl (严格)"("Value"=w1544) -> ()  [unwired: 2 in, 2 out]
                                }
                                frame "Append 8" {
                                n619 = property on="Sheet 9" class="Tbl (严格)"("Value"=w1545) -> ()  [unwired: 2 in, 2 out]
                                }
                                frame "Append 9" {
                                n620 = property on="Sheet 10" class="Tbl (严格)"("Value"=w1546) -> ()  [unwired: 2 in, 2 out]
                                }
                                frame "Append 10" {
                                n621 = property on="Sheet 11" class="Tbl (严格)"("Value"=w1547) -> ()  [unwired: 2 in, 2 out]
                                }
                                frame "Append 11" {
                                n622 = property on="Sheet 12" class="Tbl (严格)"("Value"=w1548) -> ()  [unwired: 2 in, 2 out]
                                }
                                frame "Append 12" {
                                n623 = property on="Sheet 13" class="Tbl (严格)"("Value"=w1549) -> ()  [unwired: 2 in, 2 out]
                                }
                                frame "Append 13" {
                                n624 = property on="Sheet 14" class="Tbl (严格)"("Value"=w1550) -> ()  [unwired: 2 in, 2 out]
                                }
                                frame "Append 14" {
                                n625 = property on="Sheet 15" class="Tbl (严格)"("Value"=w1551) -> ()  [unwired: 2 in, 2 out]
                                }
                                frame "Append 15" {
                                n626 = property on="Sheet 16" class="Tbl (严格)"("Value"=w1552) -> ()  [unwired: 2 in, 2 out]
                                }
                                frame "Append 16" {
                                n627 = property on="Sheet 17" class="Tbl (严格)"("Value"=w1553) -> ()  [unwired: 2 in, 2 out]
                                }
                                frame "Append 17" {
                                n628 = property on="Sheet 18" class="Tbl (严格)"("Value"=w1554) -> ()  [unwired: 2 in, 2 out]
                                }
                                frame "Append 18" {
                                n629 = property on="Sheet 19" class="Tbl (严格)"("Value"=w1555) -> ()  [unwired: 2 in, 2 out]
                                }
                                frame "Append 19" {
                                n630 = property on="Sheet 20" class="Tbl (严格)"("Value"=w1556) -> ()  [unwired: 2 in, 2 out]
                                }
                                frame "Append 20" {
                                n631 = property on="Sheet 21" class="Tbl (严格)"("Value"=w1557) -> ()  [unwired: 2 in, 2 out]
                                }
                              }
                            }
                          }
                          n632 = Array Max & Min(array=w1452) -> (max value=w1454:dbl, min value=w1453:dbl)  [unwired: 2 out]
                          n633 = property on="Chart" class="XYGraph (严格)"("XScale.Maximum"=w1454, "XScale.Minimum"=w1453) -> ()  [unwired: 2 in, 2 out]
                          n634 = case shown="\"Append 2\"" w1444 {
                            tunnel: [0 ("disabled index (row)") 1 ("disabled index (row)") 2 ("disabled index (row)") 3 ("disabled index (row)") 4 ("disabled index (row)") 5 ("disabled index (row)") 6 ("disabled index (row)") 7 ("disabled index (row)") 8 ("disabled index (row)") 9 ("disabled index (row)") 10 ("disabled index (row)") 11 ("disabled index (row)") 12 ("disabled index (row)") 13 ("disabled index (row)") 14 ("disabled index (row)") 15 ("disabled index (row)") 16 ("disabled index (row)") 17 ("disabled index (row)") 18 ("disabled index (row)") 19 ("disabled index (row)") 20 ("disabled index (row)")] -> w1445
                            frame "Data", Default {
                            }
                            frame "Append 1" {
                            }
                            frame "Append 2" {
                            }
                            frame "Append 3" {
                            }
                            frame "Append 4" {
                            }
                            frame "Append 5" {
                            }
                            frame "Append 6" {
                            }
                            frame "Append 7" {
                            }
                            frame "Append 8" {
                            }
                            frame "Append 9" {
                            }
                            frame "Append 10" {
                            }
                            frame "Append 11" {
                            }
                            frame "Append 12" {
                            }
                            frame "Append 13" {
                            }
                            frame "Append 14" {
                            }
                            frame "Append 15" {
                            }
                            frame "Append 16" {
                            }
                            frame "Append 17" {
                            }
                            frame "Append 18" {
                            }
                            frame "Append 19" {
                            }
                            frame "Append 20" {
                            }
                          }
                          n635 = Bundle(w1452, w1442) -> (w1396:cluster{dbl[], dbl[]})  [unwired: 1 in]
                          n636 = Bundle(w1441, w1442) -> (w1440:cluster{dbl[], dbl[]})  [unwired: 1 in]
                          n637 = Bundle(w1452, w1441) -> (w1463:cluster{dbl[], dbl[]})  [unwired: 1 in]
                          n638 = property on="TempChart" class="Arr (严格)"() -> ("Value"=w1447:cluster{sgl[], dbl[]}[])  [unwired: 2 in, 2 out]
                          n639 = Replace Array Subset(array=w1447, new element=w1396, index=w1445) -> (w1446:cluster{sgl[], dbl[]}[])
                          n640 = Build Array (concatenate)(w1446, w1463, w1440) -> (w1434:cluster{dbl[], dbl[]}[])
                          n641 = property on="TempChart" class="Arr (严格)"("Value"=w1446) -> ()  [unwired: 2 in, 2 out]
                          n642 = property on="Chart" class="XYGraph (严格)"("Value"=w1434) -> ()  [unwired: 2 in, 2 out]
                          n643 = property on="XY图" class="XYGraph (严格)"("Value"=w1396) -> ()  [unwired: 2 in, 2 out]
                        }
                        n644 = property on="Chart" class="XYGraph (严格)"("Active Plot"=w1381, "Plot.Visible?"=TRUE ("Plot.Visible")) -> ()  [unwired: 2 in, 2 out]
                      }
                    }
                  }
                  frame True {
                  }
                }
              }
              frame #2 {
                n645 = case shown="假" w1584 {
                  tunnel: [T7."Disabled and Grayed Out" ("Disabled") T7."Enabled" ("Disabled")] -> w1585
                  tunnel: [T7."Enabled" ("Disabled") w1629] -> w1583
                  frame False {
                  }
                  frame True {
                    n646 = global read "Global 1.vi" "Timeout (10000 ms)"() -> (w1627:i32)
                    n647 = Greater Than 0?(x=w1627) -> (x > 0?=w1628:bool)
                    n648 = case shown="真" w1628 {
                      tunnel: [T7."Enabled" ("Disabled") T7."Disabled and Grayed Out" ("Disabled")] -> w1629
                      frame False {
                      }
                      frame True {
                        n649 = Wait (ms)(milliseconds to wait=u32 1000) -> ()  [unwired: 1 out]
                      }
                    }
                  }
                }
                n650 = case shown="假" w1586 {
                  frame False {
                  }
                  frame True {
                    w1634 = FALSE ("Append")
                    n651 = global write "Global 1.vi" "Append flage"(w1634) -> ()
                    n652 = property on="Append" class="Bool (严格)"("Value"=w1634) -> ()  [unwired: 2 in, 2 out]
                  }
                }
                n653 = case shown="真" w1588 {
                  frame False {
                  }
                  frame True {
                    n654 = property on="SetOK" class="Bool (严格)"("Value"=FALSE ("SetOK")) -> ()  [unwired: 2 in, 2 out]
                  }
                }
                n655 = property on="RunState" class="Clust (严格)"("Visible"=FALSE) -> ()  [unwired: 2 in, 2 out]
                n656 = property on="Stop But" class="Bool (严格)"("DisabledEnum"=w1585) -> ()  [unwired: 2 in, 2 out]
                n657 = property on="Save All" class="Bool (严格)"("DisabledEnum"=w1583) -> ()  [unwired: 2 in, 2 out]
                n658 = property on="Append" class="Bool (严格)"("DisabledEnum"=w1583) -> ()  [unwired: 2 in, 2 out]
                n659 = property on="Save" class="Bool (严格)"("DisabledEnum"=w1583) -> ()  [unwired: 2 in, 2 out]
                n660 = property on="Repeat" class="Bool (严格)"("DisabledEnum"=w1583) -> ()  [unwired: 2 in, 2 out]
                n661 = property on="SetOK" class="Bool (严格)"("DisabledEnum"=w1583) -> ()  [unwired: 2 in, 2 out]
                n662 = property on="Clear" class="Bool (严格)"("DisabledEnum"=w1583) -> ()  [unwired: 2 in, 2 out]
                n663 = property on="Move All" class="Bool (严格)"("DisabledEnum"=w1583) -> ()  [unwired: 2 in, 2 out]
                n664 = property on="Chart" class="XYGraph (严格)"() -> ("Value"=w1580:cluster{dbl[], dbl[]}[], "YScale.Maximum"=w1582:dbl, "YScale.Minimum"=w1581:dbl, "XScale.Maximum"=w1576:dbl, "XScale.Minimum"=w1575:dbl)  [unwired: 2 in, 2 out]
                n665 = for {
                  N: 2 -> [_]
                  tunnel: w1582 -> [w1597]
                  tunnel: w1581 -> [w1595]
                  shift-right: [w1601] -> w1579
                  shift-left: w1580 -> [w1603]
                  tunnel: 21 ("index") -> [w1600]
                  tunnel: w1576 -> [w1593]
                  tunnel: w1575 -> [w1592]
                  i -> [w1598]
                  n666 = Add(x=w1600, y=w1598) -> (x+y=w1599:i32)
                  n667 = Equal To 0?(x=w1598) -> (x = 0?=w1589:bool)
                  n668 = Index Array(array=w1603, index=w1599) -> (element=w1606:cluster{dbl[], dbl[]})
                  n669 = case shown="真" w1589 {
                    tunnel: w1597 -> [w1622 _]
                    tunnel: [w1622 w1624] -> w1596
                    tunnel: w1595 -> [w1621 _]
                    tunnel: [w1621 w1623] -> w1594
                    tunnel: w1593 -> [_ w1624]
                    tunnel: w1592 -> [_ w1623]
                    frame False {
                    }
                    frame True {
                    }
                  }
                  n670 = Unbundle(w1606) -> (w1591:dbl[], w1605:dbl[])
                  n671 = case shown="真" w1589 {
                    tunnel: w1605 -> [w1613 w1614]
                    tunnel: [w1610 w1614] -> w1604
                    tunnel: w1596 -> [w1609 w1618]
                    tunnel: w1594 -> [w1608 w1617]
                    tunnel: w1591 -> [w1607 w1616]
                    tunnel: [w1607 w1615] -> w1590
                    frame False {
                      n672 = Array Max & Min(array=w1613) -> (max index (indices)=w1612:i32, min index (indices)=w1611:i32)  [unwired: 2 out]
                      n673 = Replace Array Subset(array=w1613, new element #1=w1609, index #1=w1612, new element #2=w1608, index #2=w1611) -> (w1610:dbl[])
                    }
                    frame True {
                      n674 = Array Max & Min(array=w1616) -> (max index (indices)=w1620:i32, min index (indices)=w1619:i32)  [unwired: 2 out]
                      n675 = Replace Array Subset(array=w1616, new element #1=w1618, index #1=w1620, new element #2=w1617, index #2=w1619) -> (w1615:dbl[])
                    }
                  }
                  n676 = Bundle(cluster=w1606, w1590, w1604) -> (w1602:cluster{dbl[], dbl[]})
                  n677 = Replace Array Subset(array=w1603, new element=w1602, index=w1599) -> (w1601:cluster{dbl[], dbl[]}[])
                }
                n678 = property on="Chart" class="XYGraph (严格)"("Value"=w1579) -> ()  [unwired: 2 in, 2 out]
              }
            }
          }
        }
        n679 = local read "EXIT"() -> (w630:bool)
        n680 = node-c288() -> ()  [unwired: 1 in, 1 out]
      }
      n681 = node-c288() -> (w67:T8)  [unwired: 4 in]
      n682 = timed-loop {
        tunnel: w71 -> [w74]
        tunnel: w70 -> [w73]
        timing: w67 -> [_]
        timing-out: [_] -> w66
        stop <- w75 stop-if-true
        n683 = node-c288() -> ()  [unwired: 1 in, 1 out]
        n684 = event shown="[2] \"Append\": 值改变" {
          selector: _ -> [_ _ _ _ _ _ _ _ _ _ _ _ _ _]
          dyn-events: _ -> [_ _ _ _ _ _ _ _ _ _ _ _ _ _]
          timeout: _ -> [_ _ _ _ _ _ _ _ _ _ _ _ _ _]
          tunnel: [_ _ _ _ _ _ _ _ w363 _ _ _ _ _] -> w75
          tunnel: w74 -> [_ _ _ _ _ _ _ _ w364 _ _ _ _ _]
          tunnel: w73 -> [_ _ w148 w179 w198 w206 w276 _ _ _ _ _ _ _]
          event "Stop But": Value Change {
            n685 = event-data() -> ("NewVal"=w78:bool)  [unwired: 1 in, 5 out]
            n686 = case shown="真" w78 {
              frame False {
              }
              frame True {
                n687 = stacked-sequence {
                  frame #0 {
                    n688 = global write "Global 1.vi" "Timeout (10000 ms)"(-1 ("Timeout (10000 ms)")) -> ()
                  }
                  frame #1 {
                    n689 = Wait (ms)(milliseconds to wait=u32 200) -> ()  [unwired: 1 out]
                  }
                  frame #2 {
                    w82 = T7."Enabled" ("Disabled")
                    w83 = FALSE ("Repeat")
                    n690 = property on="Repeat" class="Bool (严格)"("Value"=w83) -> (error out=w84:errorcluster)  [unwired: 2 in, 1 out]
                    n691 = property on="SetOK" class="Bool (严格)"(error in=w84, "Value"=w83) -> (error out=w81:errorcluster)  [unwired: 1 in, 1 out]
                    n692 = property on="Append" class="Bool (严格)"("DisabledEnum"=w82) -> ()  [unwired: 2 in, 2 out]
                    n693 = property on="Repeat" class="Bool (严格)"("DisabledEnum"=w82) -> ()  [unwired: 2 in, 2 out]
                    n694 = property on="SetOK" class="Bool (严格)"("DisabledEnum"=w82) -> ()  [unwired: 2 in, 2 out]
                    n695 = property on="Save All" class="Bool (严格)"(error in=w81, "DisabledEnum"=w82) -> ()  [unwired: 1 in, 2 out]
                    n696 = property on="Save" class="Bool (严格)"("DisabledEnum"=w82) -> ()  [unwired: 2 in, 2 out]
                    n697 = property on="Clear" class="Bool (严格)"("DisabledEnum"=w82) -> ()  [unwired: 2 in, 2 out]
                    n698 = property on="Move All" class="Bool (严格)"("DisabledEnum"=w82) -> ()  [unwired: 2 in, 2 out]
                  }
                }
              }
            }
          }
          event "Save", "Save All": Value Change {
            n699 = event-data() -> ("NewVal"=w85:bool)  [unwired: 1 in, 5 out]
            n700 = case shown="真" w85 {
              frame False {
              }
              frame True {
                n701 = stacked-sequence {
                  frame #0 {
                    w86 = FALSE ("Legend:Visible")
                    n702 = property on="Chart" class="XYGraph (严格)"("Legend Visible"=w86, "Palette Visible"=w86) -> ()  [unwired: 2 in, 2 out]
                  }
                  frame #1 {
                    n703 = property on="Sheet 2" class="Tbl (严格)"() -> ("Value"=w107:string[][])  [unwired: 2 in, 2 out]
                    n704 = property on="Sheet 3" class="Tbl (严格)"() -> ("Value"=w106:string[][])  [unwired: 2 in, 2 out]
                    n705 = property on="Sheet 4" class="Tbl (严格)"() -> ("Value"=w105:string[][])  [unwired: 2 in, 2 out]
                    n706 = property on="Sheet 5" class="Tbl (严格)"() -> ("Value"=w104:string[][])  [unwired: 2 in, 2 out]
                    n707 = property on="Sheet 6" class="Tbl (严格)"() -> ("Value"=w103:string[][])  [unwired: 2 in, 2 out]
                    n708 = property on="Sheet 7" class="Tbl (严格)"() -> ("Value"=w102:string[][])  [unwired: 2 in, 2 out]
                    n709 = property on="Sheet 19" class="Tbl (严格)"() -> ("Value"=w90:string[][])  [unwired: 2 in, 2 out]
                    n710 = property on="Sheet 20" class="Tbl (严格)"() -> ("Value"=w89:string[][])  [unwired: 2 in, 2 out]
                    n711 = property on="Sheet 21" class="Tbl (严格)"() -> ("Value"=w88:string[][])  [unwired: 2 in, 2 out]
                    n712 = property on="Sheet 8" class="Tbl (严格)"() -> ("Value"=w101:string[][])  [unwired: 2 in, 2 out]
                    n713 = property on="Sheet 9" class="Tbl (严格)"() -> ("Value"=w100:string[][])  [unwired: 2 in, 2 out]
                    n714 = property on="Sheet 10" class="Tbl (严格)"() -> ("Value"=w99:string[][])  [unwired: 2 in, 2 out]
                    n715 = property on="Sheet 11" class="Tbl (严格)"() -> ("Value"=w98:string[][])  [unwired: 2 in, 2 out]
                    n716 = property on="Sheet 12" class="Tbl (严格)"() -> ("Value"=w97:string[][])  [unwired: 2 in, 2 out]
                    n717 = property on="Sheet 14" class="Tbl (严格)"() -> ("Value"=w95:string[][])  [unwired: 2 in, 2 out]
                    n718 = property on="Sheet 15" class="Tbl (严格)"() -> ("Value"=w94:string[][])  [unwired: 2 in, 2 out]
                    n719 = property on="Sheet 16" class="Tbl (严格)"() -> ("Value"=w93:string[][])  [unwired: 2 in, 2 out]
                    n720 = property on="Sheet 17" class="Tbl (严格)"() -> ("Value"=w92:string[][])  [unwired: 2 in, 2 out]
                    n721 = property on="Sheet 13" class="Tbl (严格)"() -> ("Value"=w96:string[][])  [unwired: 2 in, 2 out]
                    n722 = property on="Sheet 18" class="Tbl (严格)"() -> ("Value"=w91:string[][])  [unwired: 2 in, 2 out]
                    n723 = property on="Start" class="DigNum (严格)"() -> ("Value"=w135:dbl)  [unwired: 2 in, 2 out]
                    n724 = Number To Fractional String(number=w135) -> (F-format string=w124:string)  [unwired: 3 in]
                    n725 = Bundle By Name(cluster=T11 {"A 3"=[["100", "41.7", "38.5"], ["125", "41.7", "35.2"], ["160", "41.5", "37.5"], ["200", "42.3", "42.5"], ["250", "46.9", "46.8"], ["315", "51.9", "52.6"], ["400", "52.3", "46.7"], ["500  ", "46.5", "41.6"], ["630", "42.3", "35.9"], ["800", "41.1", "32.6"]], "A 4"=[["100", "41.7", "38.5"], ["125", "41.7", "35.2"], ["160", "41.5", "37.5"], ["200", "42.3", "42.5"], ["250", "46.9", "46.8"], ["315", "51.9", "52.6"], ["400", "52.3", "46.7"], ["500  ", "46.5", "41.6"], ["630", "42.3", "35.9"], ["800", "41.1", "32.6"]], "A 5"=[["100", "41.7", "38.5"], ["125", "41.7", "35.2"], ["160", "41.5", "37.5"], ["200", "42.3", "42.5"], ["250", "46.9", "46.8"], ["315", "51.9", "52.6"], ["400", "52.3", "46.7"], ["500  ", "46.5", "41.6"], ["630", "42.3", "35.9"], ["800", "41.1", "32.6"]], "A 6"=[["100", "41.7", "38.5"], ["125", "41.7", "35.2"], ["160", "41.5", "37.5"], ["200", "42.3", "42.5"], ["250", "46.9", "46.8"], ["315", "51.9", "52.6"], ["400", "52.3", "46.7"], ["500  ", "46.5", "41.6"], ["630", "42.3", "35.9"], ["800", "41.1", "32.6"]], "A 7"=[["100", "41.7", "38.5"], ["125", "41.7", "35.2"], ["160", "41.5", "37.5"], ["200", "42.3", "42.5"], ["250", "46.9", "46.8"], ["315", "51.9", "52.6"], ["400", "52.3", "46.7"], ["500  ", "46.5", "41.6"], ["630", "42.3", "35.9"], ["800", "41.1", "32.6"]], "A 8"=[["100", "41.7", "38.5"], ["125", "41.7", "35.2"], ["160", "41.5", "37.5"], ["200", "42.3", "42.5"], ["250", "46.9", "46.8"], ["315", "51.9", "52.6"], ["400", "52.3", "46.7"], ["500  ", "46.5", "41.6"], ["630", "42.3", "35.9"], ["800", "41.1", "32.6"]], "A 9"=[["100", "41.7", "38.5"], ["125", "41.7", "35.2"], ["160", "41.5", "37.5"], ["200", "42.3", "42.5"], ["250", "46.9", "46.8"], ["315", "51.9", "52.6"], ["400", "52.3", "46.7"], ["500  ", "46.5", "41.6"], ["630", "42.3", "35.9"], ["800", "41.1", "32.6"]], "A 10"=[["100", "41.7", "38.5"], ["125", "41.7", "35.2"], ["160", "41.5", "37.5"], ["200", "42.3", "42.5"], ["250", "46.9", "46.8"], ["315", "51.9", "52.6"], ["400", "52.3", "46.7"], ["500  ", "46.5", "41.6"], ["630", "42.3", "35.9"], ["800", "41.1", "32.6"]], "A 11"=[["100", "41.7", "38.5"], ["125", "41.7", "35.2"], ["160", "41.5", "37.5"], ["200", "42.3", "42.5"], ["250", "46.9", "46.8"], ["315", "51.9", "52.6"], ["400", "52.3", "46.7"], ["500  ", "46.5", "41.6"], ["630", "42.3", "35.9"], ["800", "41.1", "32.6"]], "A 12"=[["100", "41.7", "38.5"], ["125", "41.7", "35.2"], ["160", "41.5", "37.5"], ["200", "42.3", "42.5"], ["250", "46.9", "46.8"], ["315", "51.9", "52.6"], ["400", "52.3", "46.7"], ["500  ", "46.5", "41.6"], ["630", "42.3", "35.9"], ["800", "41.1", "32.6"]], "A 13"=[["100", "41.7", "38.5"], ["125", "41.7", "35.2"], ["160", "41.5", "37.5"], ["200", "42.3", "42.5"], ["250", "46.9", "46.8"], ["315", "51.9", "52.6"], ["400", "52.3", "46.7"], ["500  ", "46.5", "41.6"], ["630", "42.3", "35.9"], ["800", "41.1", "32.6"]], "A 14"=[["100", "41.7", "38.5"], ["125", "41.7", "35.2"], ["160", "41.5", "37.5"], ["200", "42.3", "42.5"], ["250", "46.9", "46.8"], ["315", "51.9", "52.6"], ["400", "52.3", "46.7"], ["500  ", "46.5", "41.6"], ["630", "42.3", "35.9"], ["800", "41.1", "32.6"]], "A 15"=[["100", "41.7", "38.5"], ["125", "41.7", "35.2"], ["160", "41.5", "37.5"], ["200", "42.3", "42.5"], ["250", "46.9", "46.8"], ["315", "51.9", "52.6"], ["400", "52.3", "46.7"], ["500  ", "46.5", "41.6"], ["630", "42.3", "35.9"], ["800", "41.1", "32.6"]], "A 16"=[["100", "41.7", "38.5"], ["125", "41.7", "35.2"], ["160", "41.5", "37.5"], ["200", "42.3", "42.5"], ["250", "46.9", "46.8"], ["315", "51.9", "52.6"], ["400", "52.3", "46.7"], ["500  ", "46.5", "41.6"], ["630", "42.3", "35.9"], ["800", "41.1", "32.6"]], "A 17"=[["100", "41.7", "38.5"], ["125", "41.7", "35.2"], ["160", "41.5", "37.5"], ["200", "42.3", "42.5"], ["250", "46.9", "46.8"], ["315", "51.9", "52.6"], ["400", "52.3", "46.7"], ["500  ", "46.5", "41.6"], ["630", "42.3", "35.9"], ["800", "41.1", "32.6"]], "A 18"=[["100", "41.7", "38.5"], ["125", "41.7", "35.2"], ["160", "41.5", "37.5"], ["200", "42.3", "42.5"], ["250", "46.9", "46.8"], ["315", "51.9", "52.6"], ["400", "52.3", "46.7"], ["500  ", "46.5", "41.6"], ["630", "42.3", "35.9"], ["800", "41.1", "32.6"]], "A 19"=[["100", "41.7", "38.5"], ["125", "41.7", "35.2"], ["160", "41.5", "37.5"], ["200", "42.3", "42.5"], ["250", "46.9", "46.8"], ["315", "51.9", "52.6"], ["400", "52.3", "46.7"], ["500  ", "46.5", "41.6"], ["630", "42.3", "35.9"], ["800", "41.1", "32.6"]], "A 20"=[["100", "41.7", "38.5"], ["125", "41.7", "35.2"], ["160", "41.5", "37.5"], ["200", "42.3", "42.5"], ["250", "46.9", "46.8"], ["315", "51.9", "52.6"], ["400", "52.3", "46.7"], ["500  ", "46.5", "41.6"], ["630", "42.3", "35.9"], ["800", "41.1", "32.6"]], "A 1"=[["100", "41.7", "38.5"], ["125", "41.7", "35.2"], ["160", "41.5", "37.5"], ["200", "42.3", "42.5"], ["250", "46.9", "46.8"], ["315", "51.9", "52.6"], ["400", "52.3", "46.7"], ["500  ", "46.5", "41.6"], ["630", "42.3", "35.9"], ["800", "41.1", "32.6"]], "A 2"=[["100", "41.7", "38.5"], ["125", "41.7", "35.2"], ["160", "41.5", "37.5"], ["200", "42.3", "42.5"], ["250", "46.9", "46.8"], ["315", "51.9", "52.6"], ["400", "52.3", "46.7"], ["500  ", "46.5", "41.6"], ["630", "42.3", "35.9"], ["800", "41.1", "32.6"]]} ("Cluster"), "A 1"=w107, "A 2"=w106, "A 3"=w105, "A 4"=w104, "A 5"=w103, "A 6"=w102, "A 7"=w101, "A 8"=w100, "A 9"=w99, "A 10"=w98, "A 11"=w97, "A 12"=w96, "A 13"=w95, "A 14"=w94, "A 15"=w93, "A 16"=w92, "A 17"=w91, "A 18"=w90, "A 19"=w89, "A 20"=w88) -> (w108:T11)
                    n726 = property on="Stop" class="DigNum (严格)"() -> ("Value"=w131:dbl)  [unwired: 2 in, 2 out]
                    n727 = property on="Step" class="DigNum (严格)"() -> ("Value"=w130:dbl)  [unwired: 2 in, 2 out]
                    n728 = property on="StoptUnit" class="Ring (严格)"() -> ("Value"=w132:u16)  [unwired: 2 in, 2 out]
                    n729 = property on="StartUnit" class="Ring (严格)"() -> ("Value"=w134:u16)  [unwired: 2 in, 2 out]
                    n730 = call "StringClearZero.vi"("String in"=w124) -> ("String out"=w121:string)  [unwired: 10 in]
                    n731 = Number To Fractional String(number=w131) -> (F-format string=w123:string)  [unwired: 3 in]
                    n732 = Number To Fractional String(number=w130) -> (F-format string=w122:string)  [unwired: 3 in]
                    n733 = case shown="真" "Save" {
                      tunnel: [w136 bool[] [TRUE, FALSE, FALSE, FALSE, FALSE, FALSE, FALSE, FALSE, FALSE, FALSE, FALSE, FALSE, FALSE, FALSE, FALSE, FALSE, FALSE, FALSE, FALSE, FALSE, FALSE] ("AppArray")] -> w110
                      frame False {
                        n734 = property on="AppArray" class="Arr (严格)"() -> ("Value"=w136:bool[])  [unwired: 2 in, 2 out]
                      }
                      frame True {
                      }
                    }
                    n735 = case shown="1" w132 {
                      tunnel: ["mV" "V"] -> w117
                      frame 0, Default {
                      }
                      frame 1 {
                      }
                    }
                    n736 = case shown="1" w134 {
                      tunnel: ["mV" "V"] -> w118
                      frame 0, Default {
                      }
                      frame 1 {
                      }
                    }
                    n737 = call "StringClearZero.vi"("String in"=w122) -> ("String out"=w120:string)  [unwired: 10 in]
                    n738 = call "StringClearZero.vi"("String in"=w123) -> ("String out"=w119:string)  [unwired: 10 in]
                    n739 = property on="Compliance" class="DigNum (严格)"() -> ("Value"=w129:sgl)  [unwired: 2 in, 2 out]
                    n740 = property on="DataPoints" class="DigNum (严格)"() -> ("Value"=w113:u32)  [unwired: 2 in, 2 out]
                    n741 = property on="StepUnit" class="Ring (严格)"() -> ("Value"=w133:u16)  [unwired: 2 in, 2 out]
                    n742 = property on="CompliancetUnit" class="Ring (严格)"() -> ("Value"=w114:u16)  [unwired: 2 in, 2 out]
                    n743 = property on="test time" class="AbsTime (严格)"() -> ("Value"=w115:timestamp)  [unwired: 2 in, 2 out]
                    n744 = property on="Sheet" class="Tbl (严格)"() -> ("Value"=w126:string[][])  [unwired: 2 in, 2 out]
                    n745 = control-ref of="Chart"() -> (w125:refnum<vi>)
                    n746 = case shown="0, 默认" w133 {
                      tunnel: [" mV" "V"] -> w116
                      frame 0, Default {
                      }
                      frame 1 {
                      }
                    }
                    n747 = case shown="2" w114 {
                      tunnel: ["μA" "mA" "A"] -> w112
                      frame 0, Default {
                      }
                      frame 1 {
                      }
                      frame 2 {
                      }
                    }
                    n748 = Number To Decimal String(number=w113) -> (decimal integer string=w111:string)  [unwired: 1 in]
                    n749 = Number To Fractional String(number=w129) -> (F-format string=w128:string)  [unwired: 3 in]
                    n750 = call "Keithley Report2400.vi"("Test operator"="深圳市展芯科技有限公司", "Start"=w121, "AppArray"=w110, "Cluster"=w108, "Stop"=w119, "Step"=w120, "Compliance"=w128, "Data"=w126, "Comp Unit"=w112, "DataPoints"=w111, "Ctl Refnum"=w125, "Start unit"=w118, "test time"=w115, "Stop Unit"=w117, "StepUnit"=w116) -> ()  [unwired: 5 in]
                  }
                  frame #2 {
                    w147 = TRUE ("Legend:Visible")
                    n751 = property on="Chart" class="XYGraph (严格)"("Legend Visible"=w147, "Palette Visible"=w147) -> ()  [unwired: 2 in, 2 out]
                  }
                }
              }
            }
          }
          event "Append": Value Change {
            n752 = event-data() -> ("NewVal"=w149:bool)  [unwired: 1 in, 5 out]
            n753 = case shown="真" w149 {
              tunnel: w148 -> [_ w155]
              frame False {
              }
              frame True {
                n754 = property on="AppArray" class="Arr (严格)"() -> ("Value"=w152:bool[])  [unwired: 2 in, 2 out]
                n755 = Search 1D Array(1D array=w152, element=FALSE) -> (index of element=w150:i32)  [unwired: 1 in]
                n756 = Greater?(x=w150, y=0) -> (0:w153:bool)
                n757 = case shown="真" w153 {
                  tunnel: w155 -> [_ w159]
                  tunnel: w150 -> [_ w158]
                  tunnel: w152 -> [_ w157]
                  frame False {
                    n758 = One Button Dialog(message="A maximum of 20 append data！") -> ()  [unwired: 1 in, 1 out]
                  }
                  frame True {
                    n759 = flat-sequence {
                      tunnel: w159 -> [w165]
                      tunnel: w158 -> [w164]
                      tunnel: w157 -> [w160]
                      frame #0 {
                        n760 = Replace Array Subset(array=w160, new element=TRUE ("element"), index=w164) -> (w161:bool[])
                        n761 = property on="Tab Control" class="TabCtl (严格)"("Value"=w164) -> (error out=w162:errorcluster)  [unwired: 2 in, 1 out]
                        n762 = property on="AppArray" class="Arr (严格)"("Value"=w161) -> ()  [unwired: 2 in, 2 out]
                        n763 = for {
                          tunnel: w165 -> [w171] mode=indexing
                          tunnel: w164 -> [w169]
                          tunnel: w162 -> [w170]
                          tunnel: w161 -> [w166] mode=indexing
                          i -> [w167]
                          n764 = Equal?(x=w167, y=w169) -> (x = y?=w168:bool)
                          n765 = case shown="假" w168 {
                            selector: w168 -> [_ w176]
                            tunnel: [w174 w176] -> w173
                            tunnel: [T12 {"Foreground Color"=263172, "Background Color"=14869218} ("Colors") T12 {"Foreground Color"=16860, "Background Color"=16777215} ("Colors")] -> w172
                            tunnel: w167 -> [_ _]
                            tunnel: w166 -> [w174 _]
                            frame False {
                            }
                            frame True {
                            }
                          }
                          n766 = property class="Page"(reference=w171, error in=w170, "PageVis"=w173, "Colors"=w172) -> ()  [unwired: 2 out]
                        }
                      }
                      frame #1 {
                        n767 = disable-structure shown="Enabled" {
                          frame Enabled {
                            n768 = global write "Global 1.vi" "Append flage"(TRUE ("Append flage")) -> ()
                          }
                          frame Disabled {
                          }
                        }
                      }
                    }
                  }
                }
              }
            }
          }
          event "SetOK": Value Change {
            n769 = event-data() -> ("NewVal"=w180:bool)  [unwired: 1 in, 5 out]
            n770 = case shown="真" w180 {
              tunnel: w179 -> [_ w184]
              frame False {
              }
              frame True {
                w182 = 0 ("index of element")
                n771 = property on="AppArray" class="Arr (严格)"() -> ("Value"=w181:bool[])  [unwired: 2 in, 2 out]
                n772 = property on="Tab Control" class="TabCtl (严格)"("Value"=w182) -> (error out=w183:errorcluster)  [unwired: 2 in, 1 out]
                n773 = for {
                  tunnel: w184 -> [w190] mode=indexing
                  tunnel: w182 -> [w188]
                  tunnel: w183 -> [w189]
                  tunnel: w181 -> [w185] mode=indexing
                  i -> [w186]
                  n774 = Equal?(x=w186, y=w188) -> (x = y?=w187:bool)
                  n775 = case shown="真" w187 {
                    selector: w187 -> [_ w195]
                    tunnel: [w193 w195] -> w192
                    tunnel: [T12 {"Foreground Color"=263172, "Background Color"=14869218} ("Colors") T12 {"Foreground Color"=16860, "Background Color"=16777215} ("Colors")] -> w191
                    tunnel: w186 -> [_ _]
                    tunnel: w185 -> [w193 _]
                    frame False {
                    }
                    frame True {
                    }
                  }
                  n776 = property class="Page"(reference=w190, error in=w189, "PageVis"=w192, "Colors"=w191) -> ()  [unwired: 2 out]
                }
              }
            }
          }
          event "Tab Control": Value Change {
            n777 = event-data() -> ("NewVal"=w197:T5)  [unwired: 1 in, 5 out]
            n778 = for {
              tunnel: w198 -> [w202] mode=indexing
              tunnel: w197 -> [w199]
              i -> [w200]
              n779 = Equal?(x=w200, y=w199) -> (x = y?=w201:bool)
              n780 = case shown="真" w201 {
                tunnel: [T12 {"Foreground Color"=263172, "Background Color"=14869218} ("Colors") T12 {"Foreground Color"=16860, "Background Color"=16777215} ("Colors")] -> w203
                tunnel: w200 -> [_ _]
                frame False {
                }
                frame True {
                }
              }
              n781 = property class="Page"(reference=w202, "Colors"=w203) -> ()  [unwired: 1 in, 2 out]
            }
          }
          event "Clear": Value Change {
            n782 = event-data() -> ("NewVal"=w207:bool)  [unwired: 1 in, 5 out]
            n783 = case shown="真" w207 {
              tunnel: w206 -> [_ w210]
              frame False {
              }
              frame True {
                n784 = property on="Tab Control" class="TabCtl (严格)"() -> ("Value"=w209:T5)  [unwired: 2 in, 2 out]
                n785 = Equal To 0?(x=w209) -> (x = 0?=w208:bool)
                n786 = case shown="假" w208 {
                  tunnel: w209 -> [w212 _]
                  tunnel: w210 -> [w211 _]
                  frame False {
                    n787 = Number To Decimal String(number=w212) -> (decimal integer string=w217:string)  [unwired: 1 in]
                    n788 = Concatenate Strings("Are you sure you want to move the Append" ("message"), w217, " data?" ("string")) -> (w218:string)
                    n789 = Two Button Dialog(message=w218, 1:"No" ("F button name (\"Cancel\")"), 2:"Yes" ("T button name (\"OK\")")) -> (T button?=w213:bool)
                    n790 = case shown="真" w213 {
                      tunnel: w212 -> [_ w223]
                      tunnel: w211 -> [_ w231]
                      frame False {
                      }
                      frame True {
                        n791 = property on="AppArray" class="Arr (严格)"() -> ("Value"=w242:bool[])  [unwired: 2 in, 2 out]
                        n792 = property on="Chart" class="XYGraph (严格)"("Active Plot"=w223, "Plot.Visible?"=FALSE ("Plot.Visible")) -> ()  [unwired: 2 in, 2 out]
                        n793 = Replace Array Subset(array=w242, new element=FALSE ("element"), index=w223) -> (w233:bool[])
                        n794 = property on="TempChart" class="Arr (严格)"() -> ("Value"=w226:cluster{sgl[], dbl[]}[])  [unwired: 2 in, 2 out]
                        n795 = case shown="\"Append 1\"" w223 {
                          tunnel: string[][] [] ("Sheet 2") -> [_ w243 w244 w245 w246 w247 w248 w249 w250 w251 w252 w253 w254 w255 w256 w257 w258 w259 w260 w261 w262]
                          frame "Data", Default {
                          }
                          frame "Append 1" {
                            n796 = property on="Sheet 2" class="Tbl (严格)"("Value"=w243) -> ()  [unwired: 2 in, 2 out]
                          }
                          frame "Append 2" {
                            n797 = property on="Sheet 3" class="Tbl (严格)"("Value"=w244) -> ()  [unwired: 2 in, 2 out]
                          }
                          frame "Append 3" {
                            n798 = property on="Sheet 4" class="Tbl (严格)"("Value"=w245) -> ()  [unwired: 2 in, 2 out]
                          }
                          frame "Append 4" {
                            n799 = property on="Sheet 5" class="Tbl (严格)"("Value"=w246) -> ()  [unwired: 2 in, 2 out]
                          }
                          frame "Append 5" {
                            n800 = property on="Sheet 6" class="Tbl (严格)"("Value"=w247) -> ()  [unwired: 2 in, 2 out]
                          }
                          frame "Append 6" {
                            n801 = property on="Sheet 7" class="Tbl (严格)"("Value"=w248) -> ()  [unwired: 2 in, 2 out]
                          }
                          frame "Append 7" {
                            n802 = property on="Sheet 8" class="Tbl (严格)"("Value"=w249) -> ()  [unwired: 2 in, 2 out]
                          }
                          frame "Append 8" {
                            n803 = property on="Sheet 9" class="Tbl (严格)"("Value"=w250) -> ()  [unwired: 2 in, 2 out]
                          }
                          frame "Append 9" {
                            n804 = property on="Sheet 10" class="Tbl (严格)"("Value"=w251) -> ()  [unwired: 2 in, 2 out]
                          }
                          frame "Append 10" {
                            n805 = property on="Sheet 11" class="Tbl (严格)"("Value"=w252) -> ()  [unwired: 2 in, 2 out]
                          }
                          frame "Append 11" {
                            n806 = property on="Sheet 12" class="Tbl (严格)"("Value"=w253) -> ()  [unwired: 2 in, 2 out]
                          }
                          frame "Append 12" {
                            n807 = property on="Sheet 13" class="Tbl (严格)"("Value"=w254) -> ()  [unwired: 2 in, 2 out]
                          }
                          frame "Append 13" {
                            n808 = property on="Sheet 14" class="Tbl (严格)"("Value"=w255) -> ()  [unwired: 2 in, 2 out]
                          }
                          frame "Append 14" {
                            n809 = property on="Sheet 15" class="Tbl (严格)"("Value"=w256) -> ()  [unwired: 2 in, 2 out]
                          }
                          frame "Append 15" {
                            n810 = property on="Sheet 16" class="Tbl (严格)"("Value"=w257) -> ()  [unwired: 2 in, 2 out]
                          }
                          frame "Append 16" {
                            n811 = property on="Sheet 17" class="Tbl (严格)"("Value"=w258) -> ()  [unwired: 2 in, 2 out]
                          }
                          frame "Append 17" {
                            n812 = property on="Sheet 18" class="Tbl (严格)"("Value"=w259) -> ()  [unwired: 2 in, 2 out]
                          }
                          frame "Append 18" {
                            n813 = property on="Sheet 19" class="Tbl (严格)"("Value"=w260) -> ()  [unwired: 2 in, 2 out]
                          }
                          frame "Append 19" {
                            n814 = property on="Sheet 20" class="Tbl (严格)"("Value"=w261) -> ()  [unwired: 2 in, 2 out]
                          }
                          frame "Append 20" {
                            n815 = property on="Sheet 21" class="Tbl (严格)"("Value"=w262) -> ()  [unwired: 2 in, 2 out]
                          }
                        }
                        n816 = property on="AppArray" class="Arr (严格)"("Value"=w233) -> (error out=w237:errorcluster)  [unwired: 2 in, 1 out]
                        n817 = Search 1D Array(1D array=w233, element=TRUE, start index (0)=w223) -> (index of element=w228:i32)
                        n818 = Greater Than 0?(x=w228) -> (x > 0?=w235:bool)
                        n819 = Index Array(array=w231, index=w223) -> (element=w240:refnum<vi>)
                        n820 = Replace Array Subset(array=w226, new element=cluster{sgl[], dbl[]} {[], []} ("new element/subarray"), index=w223) -> (w221:cluster{sgl[], dbl[]}[])
                        n821 = property class="Page"(reference=w240, error in=w237, "PageVis"=FALSE ("Page Visible"), "Colors"=T12 {"Foreground Color"=263172, "Background Color"=14869218}) -> (error out=w234:errorcluster)  [unwired: 1 out]
                        n822 = property on="Chart" class="XYGraph (严格)"() -> ("Value"=w222:cluster{dbl[], dbl[]}[])  [unwired: 2 in, 2 out]
                        n823 = property on="TempChart" class="Arr (严格)"("Value"=w221) -> ()  [unwired: 2 in, 2 out]
                        n824 = Replace Array Subset(array=w222, new element=w221) -> (w220:cluster{dbl[], dbl[]}[])  [unwired: 1 in]
                        n825 = case shown="假" w235 {
                          tunnel: w234 -> [_ _]
                          tunnel: w228 -> [_ w274]
                          tunnel: w233 -> [w268 _]
                          tunnel: [w264 w274] -> w229
                          tunnel: w223 -> [w263 _]
                          frame False {
                            n826 = Decrement(x=w263) -> (x-1=w266:T5)
                            n827 = Array Subset(array=w268, index=0, length=w263) -> (w265:bool[])
                            n828 = while {
                              tunnel: w266 -> [w272]
                              tunnel: w265 -> [w271]
                              tunnel: [w269] -> w264
                              i -> [w273]
                              stop <- w270 stop-if-true
                              n829 = Subtract(x=w272, y=w273) -> (x-y=w269:u32)
                              n830 = Index Array(array=w271, index=w269) -> (element=w270:bool)
                            }
                          }
                          frame True {
                          }
                        }
                        n831 = property on="Chart" class="XYGraph (严格)"("Value"=w220) -> ()  [unwired: 2 in, 2 out]
                        n832 = Index Array(array=w231, index=w229) -> (element=w230:refnum<vi>)
                        n833 = property on="Tab Control" class="TabCtl (严格)"("Value"=w229) -> ()  [unwired: 2 in, 2 out]
                        n834 = property class="Page"(reference=w230, "Colors"=T12 {"Foreground Color"=16860, "Background Color"=16777215}) -> ()  [unwired: 1 in, 2 out]
                      }
                    }
                  }
                  frame True {
                    n835 = One Button Dialog(message="Please selecet the append datasheet to clear！") -> ()  [unwired: 1 in, 1 out]
                  }
                }
              }
            }
          }
          event "Move All": Value Change {
            n836 = event-data() -> ("NewVal"=w277:bool)  [unwired: 1 in, 5 out]
            n837 = case shown="真" w277 {
              tunnel: w276 -> [_ w282]
              frame False {
              }
              frame True {
                n838 = Two Button Dialog(message="Are you sure you want to move all the Append?", 1:"No" ("F button name (\"Cancel\")"), 2:"Yes" ("T button name (\"OK\")")) -> (T button?=w279:bool)
                n839 = case shown="真" w279 {
                  tunnel: w282 -> [_ w283]
                  frame False {
                  }
                  frame True {
                    n840 = for {
                      tunnel: w283 -> [w295]
                      tunnel: [w292] -> _
                      tunnel: [w291] -> w287
                      tunnel: w283 -> [_] mode=indexing
                      i -> [w293]
                      n841 = Equal To 0?(x=w293) -> (x = 0?=w294:bool)
                      n842 = case shown="假" w294 {
                        tunnel: w295 -> [w296 w333]
                        tunnel: w293 -> [w301 _]
                        tunnel: [w297 _] -> w292
                        tunnel: [w296 w333] -> w291
                        frame False {
                          n843 = property on="AppArray" class="Arr (严格)"() -> ("Value"=w312:bool[])  [unwired: 2 in, 2 out]
                          n844 = property on="Chart" class="XYGraph (严格)"("Active Plot"=w301, "Plot.Visible?"=FALSE ("Plot.Visible")) -> ()  [unwired: 2 in, 2 out]
                          n845 = Replace Array Subset(array=w312, new element=FALSE ("element"), index=w301) -> (w306:bool[])
                          n846 = property on="TempChart" class="Arr (严格)"() -> ("Value"=w304:cluster{sgl[], dbl[]}[])  [unwired: 2 in, 2 out]
                          n847 = case shown="1" w301 {
                            tunnel: string[][] [] ("Sheet 2") -> [_ w313 w314 w315 w316 w317 w318 w319 w320 w321 w322 w323 w324 w325 w326 w327 w328 w329 w330 w331 w332]
                            frame 0, Default {
                            }
                            frame 1 {
                              n848 = property on="Sheet 2" class="Tbl (严格)"("Value"=w313) -> ()  [unwired: 2 in, 2 out]
                            }
                            frame 2 {
                              n849 = property on="Sheet 3" class="Tbl (严格)"("Value"=w314) -> ()  [unwired: 2 in, 2 out]
                            }
                            frame 3 {
                              n850 = property on="Sheet 4" class="Tbl (严格)"("Value"=w315) -> ()  [unwired: 2 in, 2 out]
                            }
                            frame 4 {
                              n851 = property on="Sheet 5" class="Tbl (严格)"("Value"=w316) -> ()  [unwired: 2 in, 2 out]
                            }
                            frame 5 {
                              n852 = property on="Sheet 6" class="Tbl (严格)"("Value"=w317) -> ()  [unwired: 2 in, 2 out]
                            }
                            frame 6 {
                              n853 = property on="Sheet 7" class="Tbl (严格)"("Value"=w318) -> ()  [unwired: 2 in, 2 out]
                            }
                            frame 7 {
                              n854 = property on="Sheet 8" class="Tbl (严格)"("Value"=w319) -> ()  [unwired: 2 in, 2 out]
                            }
                            frame 8 {
                              n855 = property on="Sheet 9" class="Tbl (严格)"("Value"=w320) -> ()  [unwired: 2 in, 2 out]
                            }
                            frame 9 {
                              n856 = property on="Sheet 10" class="Tbl (严格)"("Value"=w321) -> ()  [unwired: 2 in, 2 out]
                            }
                            frame 10 {
                              n857 = property on="Sheet 11" class="Tbl (严格)"("Value"=w322) -> ()  [unwired: 2 in, 2 out]
                            }
                            frame 11 {
                              n858 = property on="Sheet 12" class="Tbl (严格)"("Value"=w323) -> ()  [unwired: 2 in, 2 out]
                            }
                            frame 12 {
                              n859 = property on="Sheet 13" class="Tbl (严格)"("Value"=w324) -> ()  [unwired: 2 in, 2 out]
                            }
                            frame 13 {
                              n860 = property on="Sheet 14" class="Tbl (严格)"("Value"=w325) -> ()  [unwired: 2 in, 2 out]
                            }
                            frame 14 {
                              n861 = property on="Sheet 15" class="Tbl (严格)"("Value"=w326) -> ()  [unwired: 2 in, 2 out]
                            }
                            frame 15 {
                              n862 = property on="Sheet 16" class="Tbl (严格)"("Value"=w327) -> ()  [unwired: 2 in, 2 out]
                            }
                            frame 16 {
                              n863 = property on="Sheet 17" class="Tbl (严格)"("Value"=w328) -> ()  [unwired: 2 in, 2 out]
                            }
                            frame 17 {
                              n864 = property on="Sheet 18" class="Tbl (严格)"("Value"=w329) -> ()  [unwired: 2 in, 2 out]
                            }
                            frame 18 {
                              n865 = property on="Sheet 19" class="Tbl (严格)"("Value"=w330) -> ()  [unwired: 2 in, 2 out]
                            }
                            frame 19 {
                              n866 = property on="Sheet 20" class="Tbl (严格)"("Value"=w331) -> ()  [unwired: 2 in, 2 out]
                            }
                            frame 20 {
                              n867 = property on="Sheet 21" class="Tbl (严格)"("Value"=w332) -> ()  [unwired: 2 in, 2 out]
                            }
                          }
                          n868 = property on="AppArray" class="Arr (严格)"("Value"=w306) -> (error out=w307:errorcluster)  [unwired: 2 in, 1 out]
                          n869 = Index Array(array=w296, index=w301) -> (element=w310:refnum<vi>)
                          n870 = Replace Array Subset(array=w304, new element=cluster{sgl[], dbl[]} {[], []} ("new element/subarray"), index=w301) -> (w299:cluster{sgl[], dbl[]}[])
                          n871 = property on="Chart" class="XYGraph (严格)"() -> ("Value"=w300:cluster{dbl[], dbl[]}[])  [unwired: 2 in, 2 out]
                          n872 = property class="Page"(reference=w310, error in=w307, "PageVis"=FALSE ("Page Visible"), "Colors"=T12 {"Foreground Color"=263172, "Background Color"=14869218}) -> ()  [unwired: 2 out]
                          n873 = property on="TempChart" class="Arr (严格)"("Value"=w299) -> ()  [unwired: 2 in, 2 out]
                          n874 = Replace Array Subset(array=w300, new element=w299) -> (w298:cluster{dbl[], dbl[]}[])  [unwired: 1 in]
                          n875 = property on="Chart" class="XYGraph (严格)"("Value"=w298) -> (error out=w297:errorcluster)  [unwired: 2 in, 1 out]
                        }
                        frame True {
                        }
                      }
                    }
                    n876 = Index Array(array=w287, index=0) -> (element=w288:refnum<vi>)
                    n877 = property class="Page"(reference=w288, "PageVis"=TRUE ("Page Visible"), "Colors"=T12 {"Foreground Color"=16860, "Background Color"=16777215}) -> (error out=w285:errorcluster)  [unwired: 1 in, 1 out]
                    n878 = property on="Tab Control" class="TabCtl (严格)"(error in=w285, "Value"=T5."Data" ("Tab Control")) -> ()  [unwired: 1 in, 2 out]
                  }
                }
              }
            }
          }
          event "IV CLUS.StartUnit", "IV CLUS.StoptUnit", "IV CLUS.StepUnit", "It CLUS.VoltageUnit IT", "Vt CLUS.CompUnit VT": Value Change {
            n879 = event-data() -> ("CtlRef"=w338:refnum<vi>, "NewVal"=w336:u16)  [unwired: 1 in, 4 out]
            n880 = property on="Series 2600B" class="Ring (严格)"() -> ("Value"=w334:u16)  [unwired: 2 in, 2 out]
            n881 = case shown="1" w336 {
              tunnel: [900.0 ("Data Entry Limits:Maximum") w340] -> w335
              tunnel: w334 -> [_ w341]
              frame 0, Default {
              }
              frame 1 {
                n882 = case shown="0, 默认" w341 {
                  tunnel: [40.0 ("Data Entry Limits:Maximum") 40.0 ("Data Entry Limits:Maximum") 40.0 ("Data Entry Limits:Maximum") 200.0 ("Data Entry Limits:Maximum") 200.0 ("Data Entry Limits:Maximum") 200.0 ("Data Entry Limits:Maximum") 200.0 ("Data Entry Limits:Maximum") 200.0 ("Data Entry Limits:Maximum") 200.0 ("Data Entry Limits:Maximum")] -> w340
                  frame 0, Default {
                  }
                  frame 1 {
                  }
                  frame 2 {
                  }
                  frame 3 {
                  }
                  frame 4 {
                  }
                  frame 5 {
                  }
                  frame 6 {
                  }
                  frame 7 {
                  }
                  frame 8 {
                  }
                }
              }
            }
            n883 = property class="Ring (严格)"(reference=w338) -> ("Label.Text"=w337:string)  [unwired: 1 in, 2 out]
            n884 = case shown="\"VoltageUnit IT\"" w337 {
              tunnel: w335 -> [w351 w353 w356 w358 w360]
              frame "StartUnit", Default {
                n885 = Negate(x=w351) -> (-x=w352:dbl)
                n886 = property on="Start" class="DigNum (严格)"("Maximum"=w351, "Minimum"=w352) -> ()  [unwired: 2 in, 2 out]
              }
              frame "StoptUnit" {
                n887 = Negate(x=w353) -> (-x=w354:dbl)
                n888 = property on="Stop" class="DigNum (严格)"("Maximum"=w353, "Minimum"=w354) -> ()  [unwired: 2 in, 2 out]
              }
              frame "StepUnit" {
                n889 = property on="Step" class="DigNum (严格)"("Maximum"=w356, "Minimum"=0.001 ("Data Entry Limits:Minimum")) -> ()  [unwired: 2 in, 2 out]
              }
              frame "VoltageUnit IT" {
                n890 = property on="Voltage IT" class="DigNum (严格)"("Maximum"=w358, "Minimum"=0.001 ("Data Entry Limits:Minimum")) -> ()  [unwired: 2 in, 2 out]
              }
              frame "CompUnit VT" {
                n891 = property on="CompUnit VT" class="Ring (严格)"("Maximum"=w360, "Minimum"=0.001 ("Data Entry Limits:Minimum")) -> ()  [unwired: 2 in, 2 out]
              }
            }
          }
          event "EXIT": Value Change; Panel Close {
            w363 = TRUE ("NewVal")
            n892 = event-data() -> ()  [unwired: 1 in, 3 out]
            n893 = property on="EXIT" class="Bool (严格)"("Value"=w363) -> (error out=w362:errorcluster)  [unwired: 2 in, 1 out]
            n894 = flat-sequence {
              tunnel: w362 -> [w367]
              tunnel: [w367] -> w361
              frame #0 {
                n895 = Wait (ms)(milliseconds to wait=u32 50) -> ()  [unwired: 1 out]
              }
            }
            n896 = call <instrlib>:"Close.vi"("error in (no error)"=w361, "VISA resource name"=w364) -> ("error out"=w365:errorcluster)  [unwired: 9 in]
            n897 = call <vilib>:"Simple Error Handler.vi"("error in (no error)"=w365) -> ()  [unwired: 4 in, 5 out]
          }
          event "XYConvert": Value Change {
            n898 = event-data() -> ("NewVal"=w379:bool)  [unwired: 1 in, 5 out]
            n899 = property on="Test Type" class="RadioBtnsControl (严格)"() -> ("Value"=w368:enum32{"IV", "IT", "VT", "MOSFET"})  [unwired: 2 in, 2 out]
            n900 = case shown="\"VT\"" w368 {
              tunnel: ["AV" ("X Scale.Name Label.Text") "Time" ("X Scale.Name Label.Text") "Time" ("X Scale.Name Label.Text")] -> w378
              tunnel: ["AI" ("X Scale.Name Label.Text") "I" ("X Scale.Name Label.Text") "V" ("X Scale.Name Label.Text")] -> w377
              frame "IV", Default {
              }
              frame "IT" {
              }
              frame "VT" {
              }
            }
            n901 = case shown="假" w379 {
              tunnel: w378 -> [w401 w403]
              tunnel: w377 -> [w400 w402]
              tunnel: [w401 w402] -> w376
              tunnel: [w400 w403] -> w375
              frame False {
              }
              frame True {
              }
            }
            n902 = property on="Chart" class="XYGraph (严格)"("XScale.NameLbl.Text"=w376, "YScale.NameLbl.Text"=w375) -> ("Value"=w374:cluster{dbl[], dbl[]}[])  [unwired: 2 in, 2 out]
            n903 = for {
              shift-right: [w390] -> w372
              shift-left: w374 -> [w393]
              tunnel: w374 -> [_] mode=indexing
              i -> [w389]
              n904 = Index Array(array=w393, index=w389) -> (element=w392:cluster{dbl[], dbl[]})
              n905 = Equal To 0?(x=w389) -> (x = 0?=w388:bool)
              n906 = Unbundle(w392) -> (w386:dbl[], w387:dbl[])
              n907 = case shown="真" w388 {
                tunnel: w387 -> [_ w399]
                tunnel: w386 -> [_ w398]
                frame False {
                }
                frame True {
                  n908 = Array Max & Min(array=w398) -> (max value=w395:dbl, min value=w394:dbl)  [unwired: 2 out]
                  n909 = Array Max & Min(array=w399) -> (max value=w397:dbl, min value=w396:dbl)  [unwired: 2 out]
                  n910 = property on="Chart" class="XYGraph (严格)"("XScale.Maximum"=w397, "XScale.Minimum"=w396, "YScale.Maximum"=w395, "YScale.Minimum"=w394) -> ()  [unwired: 2 in, 2 out]
                }
              }
              n911 = Bundle(w387, w386) -> (w391:cluster{dbl[], dbl[]})  [unwired: 1 in]
              n912 = Replace Array Subset(array=w393, new element=w391, index=w389) -> (w390:cluster{dbl[], dbl[]}[])
            }
            n913 = property on="Chart" class="XYGraph (严格)"("Value"=w372) -> ()  [unwired: 2 in, 2 out]
            n914 = Array Subset(array=w372, length=21) -> (w370:cluster{dbl[], dbl[]}[])  [unwired: 1 in]
            n915 = property on="TempChart" class="Arr (严格)"() -> ("Value"=w373:cluster{sgl[], dbl[]}[])  [unwired: 2 in, 2 out]
            n916 = Replace Array Subset(array=w373, new element=w370) -> (w369:cluster{sgl[], dbl[]}[])  [unwired: 1 in]
            n917 = property on="TempChart" class="Arr (严格)"("Value"=w369) -> ()  [unwired: 2 in, 2 out]
          }
          event "Test Type": Value Change {
            w408 = string[][] [] ("Sheet 7")
            n918 = event-data() -> ("NewVal"=w416:enum32{"IV", "IT", "VT", "MOSFET"})  [unwired: 1 in, 5 out]
            n919 = case shown="\"VT\"" w416 {
              tunnel: ["AV" ("X Scale.Name Label.Text") _ "Time" ("X Scale.Name Label.Text") "Time" ("X Scale.Name Label.Text")] -> w414
              tunnel: ["AI" ("Y Scale.Name Label.Text") _ "I" ("Y Scale.Name Label.Text") "V" ("Y Scale.Name Label.Text")] -> w412
              tunnel: [string[] ["AV(V)", "AI(A)", "RES(Ohm)"] ("Column Header Strings[]") string[] ["GateV(V)", "Drain(A)", "RES(Ohm)"] ("Column Header Strings[]") string[] ["Time(s)", "I(A)", "R"] ("Column Header Strings[]") string[] ["Time(s)", "V(V)", ""] ("Column Header Strings[]")] -> w409
              tunnel: [TRUE ("Visible") w428 w429 w434] -> w407
              tunnel: [w421 w428 TRUE ("Visible") w434] -> w406
              tunnel: [w421 w428 w429 TRUE ("Visible")] -> w405
              tunnel: [w421 TRUE w429 w434] -> w404
              frame "IV", Default {
                w421 = FALSE ("Visible")
              }
              frame "MOSFET" {
                w428 = FALSE
              }
              frame "IT" {
                w429 = FALSE ("Visible")
              }
              frame "VT" {
                w434 = FALSE ("Visible")
              }
            }
            n920 = property on="XYConvert" class="Bool (严格)"() -> ("Value"=w415:bool)  [unwired: 2 in, 2 out]
            n921 = property on="IV CLUS" class="Clust (严格)"("Visible"=w407) -> ()  [unwired: 2 in, 2 out]
            n922 = property on="DataPoints" class="DigNum (严格)"("Visible"=w407) -> ()  [unwired: 2 in, 2 out]
            n923 = property on="It CLUS" class="Clust (严格)"("Visible"=w406) -> ()  [unwired: 2 in, 2 out]
            n924 = property on="Vt CLUS" class="Clust (严格)"("Visible"=w405) -> ()  [unwired: 2 in, 2 out]
            n925 = case shown="真" w415 {
              tunnel: [w418 w419] -> w413
              tunnel: w414 -> [w418 w420]
              tunnel: w412 -> [w417 w419]
              tunnel: [w417 w420] -> w411
              frame False {
              }
              frame True {
              }
            }
            n926 = property on="Sheet 2" class="Tbl (严格)"("Column Headers[]"=w409, "Value"=w408) -> ()  [unwired: 2 in, 2 out]
            n927 = property on="Sheet 3" class="Tbl (严格)"("Column Headers[]"=w409, "Value"=w408) -> ()  [unwired: 2 in, 2 out]
            n928 = property on="Sheet" class="Tbl (严格)"("Column Headers[]"=w409, "Value"=w408) -> ()  [unwired: 2 in, 2 out]
            n929 = property on="Sheet 6" class="Tbl (严格)"("Column Headers[]"=w409, "Value"=w408) -> ()  [unwired: 2 in, 2 out]
            n930 = property on="Sheet 7" class="Tbl (严格)"("Column Headers[]"=w409, "Value"=w408) -> ()  [unwired: 2 in, 2 out]
            n931 = property on="Sheet 4" class="Tbl (严格)"("Column Headers[]"=w409, "Value"=w408) -> ()  [unwired: 2 in, 2 out]
            n932 = property on="Sheet 5" class="Tbl (严格)"("Column Headers[]"=w409, "Value"=w408) -> ()  [unwired: 2 in, 2 out]
            n933 = property on="MOSFET CLUS" class="Clust (严格)"("Visible"=w404) -> ()  [unwired: 2 in, 2 out]
            n934 = property on="Sheet 18" class="Tbl (严格)"("Column Headers[]"=w409, "Value"=w408) -> ()  [unwired: 2 in, 2 out]
            n935 = property on="Sheet 20" class="Tbl (严格)"("Column Headers[]"=w409, "Value"=w408) -> ()  [unwired: 2 in, 2 out]
            n936 = property on="Chart" class="XYGraph (严格)"("XScale.NameLbl.Text"=w413, "YScale.NameLbl.Text"=w411, "Value"=cluster{dbl[], dbl[]}[] [] ("Chart")) -> ()  [unwired: 2 in, 2 out]
            n937 = property on="Sheet 16" class="Tbl (严格)"("Column Headers[]"=w409, "Value"=w408) -> ()  [unwired: 2 in, 2 out]
            n938 = property on="Sheet 9" class="Tbl (严格)"("Column Headers[]"=w409, "Value"=w408) -> ()  [unwired: 2 in, 2 out]
            n939 = property on="Sheet 8" class="Tbl (严格)"("Column Headers[]"=w409, "Value"=w408) -> ()  [unwired: 2 in, 2 out]
            n940 = property on="Sheet 13" class="Tbl (严格)"("Column Headers[]"=w409, "Value"=w408) -> ()  [unwired: 2 in, 2 out]
            n941 = property on="Sheet 10" class="Tbl (严格)"("Column Headers[]"=w409, "Value"=w408) -> ()  [unwired: 2 in, 2 out]
            n942 = property on="Sheet 11" class="Tbl (严格)"("Column Headers[]"=w409, "Value"=w408) -> ()  [unwired: 2 in, 2 out]
            n943 = property on="Sheet 15" class="Tbl (严格)"("Column Headers[]"=w409, "Value"=w408) -> ()  [unwired: 2 in, 2 out]
            n944 = property on="Sheet 12" class="Tbl (严格)"("Column Headers[]"=w409, "Value"=w408) -> ()  [unwired: 2 in, 2 out]
            n945 = property on="Sheet 21" class="Tbl (严格)"("Column Headers[]"=w409, "Value"=w408) -> ()  [unwired: 2 in, 2 out]
            n946 = property on="Sheet 19" class="Tbl (严格)"("Column Headers[]"=w409, "Value"=w408) -> ()  [unwired: 2 in, 2 out]
            n947 = property on="Sheet 17" class="Tbl (严格)"("Column Headers[]"=w409, "Value"=w408) -> ()  [unwired: 2 in, 2 out]
            n948 = property on="Sheet 14" class="Tbl (严格)"("Column Headers[]"=w409, "Value"=w408) -> ()  [unwired: 2 in, 2 out]
          }
          event "IV CLUS.Step": Value Change {
            n949 = event-data() -> ("NewVal"=w442:dbl)  [unwired: 1 in, 5 out]
            n950 = property on="Start" class="DigNum (严格)"() -> ("Value"=w450:dbl)  [unwired: 2 in, 2 out]
            n951 = property on="StartUnit" class="Ring (严格)"() -> ("Value"=w449:u16)  [unwired: 2 in, 2 out]
            n952 = property on="Stop" class="DigNum (严格)"() -> ("Value"=w446:dbl)  [unwired: 2 in, 2 out]
            n953 = property on="StoptUnit" class="Ring (严格)"() -> ("Value"=w447:u16)  [unwired: 2 in, 2 out]
            n954 = property on="StepUnit" class="Ring (严格)"() -> ("Value"=w448:u16)  [unwired: 2 in, 2 out]
            n955 = case shown="0" w448 {
              tunnel: [1000.0 ("Start") 1.0 ("Start")] -> w452
              frame 0 {
              }
              frame 1, Default {
              }
            }
            n956 = case shown="1, 默认" w447 {
              tunnel: [1000.0 ("Start") 1.0 ("Start")] -> w451
              frame 0 {
              }
              frame 1, Default {
              }
            }
            n957 = case shown="0" w449 {
              tunnel: [1000.0 ("Start") 1.0 ("Start")] -> w453
              frame 0 {
              }
              frame 1, Default {
              }
            }
            n958 = Divide(x=w442, y=w452) -> (x/y=w439:dbl)
            n959 = Divide(x=w450, y=w453) -> (x/y=w441:dbl)
            n960 = Divide(x=w446, y=w451) -> (x/y=w440:dbl)
            n961 = Subtract(x=w440, y=w441) -> (x-y=w445:dbl)
            n962 = Absolute Value(x=w445) -> (abs(x)=w444:dbl)
            n963 = Less?(x=w444, y=w439) -> (x < y?=w443:bool)
            n964 = case shown="假" w443 {
              tunnel: w441 -> [w456 _]
              tunnel: w440 -> [w454 _]
              tunnel: w439 -> [w455 _]
              frame False {
                n965 = call "Keithley Sample Number.vi"("Step"=w455, "Stop"=w454, "Start"=w456) -> ("pointnumber"=w457:dbl)  [unwired: 7 in, 1 out]
                n966 = property on="DataPoints" class="DigNum (严格)"("Value"=w457) -> ()  [unwired: 2 in, 2 out]
              }
              frame True {
                n967 = flat-sequence {
                  tunnel: [w459] -> w458
                  tunnel: w458 -> [_]
                  frame #0 {
                    n968 = One Button Dialog(message="Parameter data out of range!") -> (true=w459:bool)  [unwired: 1 in]
                  }
                  frame #1 {
                    n969 = property on="Step" class="DigNum (严格)"("Key Focus"=TRUE, "NumText.Selection"=T13 {"Selection Start"=0, "Selection End"=10} ("Numeric Text.Selection")) -> ()  [unwired: 2 in, 2 out]
                  }
                }
              }
            }
          }
          event "IV CLUS.CompliancetUnit", "It CLUS.CompUnit-IT", "Vt CLUS.CurrUnit VT": Value Change {
            n970 = event-data() -> ("NewVal"=w473:u16)  [unwired: 1 in, 5 out]
            n971 = case shown="2, 默认" w473 {
              tunnel: [1.0 ("Data Entry Limits:Minimum") 900.0 ("Data Entry Limits:Minimum") 900.0 ("Data Entry Limits:Minimum")] -> w469
              tunnel: [0.1 ("Data Entry Limits:Minimum") 0.001 ("Data Entry Limits:Minimum") 0.1 ("Data Entry Limits:Minimum")] -> w471
              tunnel: [0.1 ("Data Entry Limits:Minimum") 0.001 ("Data Entry Limits:Minimum") 0.05 ("Data Entry Limits:Minimum")] -> w472
              frame 2, Default {
                # "A"
              }
              frame 0 {
                # "uA"
              }
              frame 1 {
                # "MA"
              }
            }
            n972 = Negate(x=w469) -> (-x=w470:dbl)
            n973 = property on="Current VT" class="DigNum (严格)"("Maximum"=w469, "Minimum"=w470) -> ()  [unwired: 2 in, 2 out]
            n974 = property on="CompCurrIT" class="DigNum (严格)"("Increment"=w472, "Maximum"=w469, "Minimum"=w471) -> ()  [unwired: 2 in, 2 out]
            n975 = property on="Compliance" class="DigNum (严格)"("Increment"=w472, "Maximum"=w469, "Minimum"=w471) -> ()  [unwired: 2 in, 2 out]
          }
          event "Series 2600B": Value Change {
            n976 = event-data() -> ("NewVal"=w483:u16)  [unwired: 1 in, 5 out]
            n977 = stacked-sequence {
              tunnel: w483 -> [w489 w499]
              frame #0 {
                w484 = u16 0 items=["Channel A", "Channel B"] ("Channel")
                n978 = Equal?(x=w489, y=u16 0) -> (x = y?=w486:bool)
                n979 = Equal?(x=w489, y=u16 3) -> (x = y?=w488:bool)
                n980 = Equal?(x=w489, y=u16 7) -> (x = y?=w487:bool)
                n981 = Compound Arithmetic op=OR(w486, w488, w487) -> (w485:bool)
                n982 = case shown="假" w485 {
                  tunnel: [i32[] [] ("Disabled Items []") i32[] [1] ("Disabled Items []")] -> w493
                  frame False {
                  }
                  frame True {
                  }
                }
                n983 = property on="Channel" class="Ring (严格)"("Value"=w484, "Disabled Items []"=w493) -> ()  [unwired: 2 in, 2 out]
              }
              frame #1 {
                w500 = sgl 0.1 ("Compliance")
                w517 = 1.0 ("Start")
                # "2636B  200V, 10A,0.1fA"
                # "2635B  200V, 10A,0.1fA"
                # "2634B  200V, 10A,1fA"
                # "2614B  200V, 10A,100fA"
                # "2611B  200V, 10A,100fA"
                # "2604B  40V, 10A,100fA"
                # "2602B  40V, 10A,100fA"
                # "2601B  40V, 10A,100fA"
                # "2612B  200V, 10A,100fA"
                n984 = property on="VoltageUnit IT" class="Ring (严格)"() -> ("Value"=w512:u16)  [unwired: 2 in, 2 out]
                n985 = property on="CompIUnit-IT" class="Ring (严格)"() -> ("Value"=w511:u16)  [unwired: 2 in, 2 out]
                n986 = property on="CurrUnit VT" class="Ring (严格)"() -> ("Value"=w510:u16)  [unwired: 2 in, 2 out]
                n987 = property on="CompUnit VT" class="Ring (严格)"() -> ("Value"=w509:u16)  [unwired: 2 in, 2 out]
                n988 = property on="StoptUnit" class="Ring (严格)"() -> ("Value"=w527:u16)  [unwired: 2 in, 2 out]
                n989 = property on="StartUnit" class="Ring (严格)"() -> ("Value"=w526:u16)  [unwired: 2 in, 2 out]
                n990 = property on="StepUnit" class="Ring (严格)"() -> ("Value"=w525:u16)  [unwired: 2 in, 2 out]
                n991 = In Range and Coerce(upper limit=u16 0, x=w499, lower limit=u16 2) -> (In Range?=w496:bool)  [unwired: 1 out]
                n992 = property on="ComplianceUnit" class="Ring (严格)"() -> ("Value"=w516:u16)  [unwired: 2 in, 2 out]
                n993 = case shown="假" w496 {
                  tunnel: w527 -> [w542 w589]
                  tunnel: w526 -> [w543 w590]
                  tunnel: w525 -> [w541 w588]
                  tunnel: [w546 w593] -> w523
                  tunnel: [w545 w592] -> w521
                  tunnel: [w544 w591] -> w520
                  tunnel: [w539 w586] -> w519
                  tunnel: [w540 w587] -> w514
                  tunnel: w516 -> [w538 w585]
                  tunnel: w512 -> [w537 w584]
                  tunnel: w511 -> [w534 w581]
                  tunnel: w510 -> [w531 w578]
                  tunnel: w509 -> [w535 w582]
                  tunnel: [w536 w583] -> w507
                  tunnel: [w533 w580] -> w505
                  tunnel: [w532 w579] -> w506
                  tunnel: [w530 w577] -> w504
                  tunnel: [w529 w576] -> w502
                  tunnel: [w528 w575] -> w501
                  frame True {
                    n994 = case shown="2" w531 {
                      tunnel: [0.001 ("Data Entry Limits:Maximum") 0.005 ("Data Entry Limits:Maximum") 5e-05 ("Data Entry Limits:Maximum")] -> w530
                      tunnel: [900.0 ("Data Entry Limits:Maximum") 900.0 ("Data Entry Limits:Maximum") 10.0 ("Data Entry Limits:Maximum")] -> w529
                      frame 0, Default {
                      }
                      frame 1 {
                      }
                      frame 2 {
                      }
                    }
                    n995 = case shown="2" w534 {
                      tunnel: [0.001 ("Data Entry Limits:Maximum") 0.005 ("Data Entry Limits:Maximum") 5e-05 ("Data Entry Limits:Maximum")] -> w532
                      tunnel: [900.0 ("Data Entry Limits:Maximum") 900.0 ("Data Entry Limits:Maximum") 10.0 ("Data Entry Limits:Maximum")] -> w533
                      frame 0, Default {
                      }
                      frame 1 {
                      }
                      frame 2 {
                      }
                    }
                    n996 = case shown="1" w535 {
                      tunnel: [900.0 ("Data Entry Limits:Maximum") 40.0 ("Data Entry Limits:Maximum")] -> w528
                      frame 0, Default {
                      }
                      frame 1 {
                      }
                    }
                    n997 = case shown="2" w538 {
                      tunnel: [0.001 ("Data Entry Limits:Maximum") 0.005 ("Data Entry Limits:Maximum") 5e-05 ("Data Entry Limits:Maximum")] -> w539
                      tunnel: [900.0 ("Data Entry Limits:Maximum") 900.0 ("Data Entry Limits:Maximum") 10.0 ("Data Entry Limits:Maximum")] -> w540
                      frame 0, Default {
                      }
                      frame 1 {
                      }
                      frame 2 {
                      }
                    }
                    n998 = case shown="1" w537 {
                      tunnel: [900.0 ("Data Entry Limits:Maximum") 40.0 ("Data Entry Limits:Maximum")] -> w536
                      frame 0, Default {
                      }
                      frame 1 {
                      }
                    }
                    n999 = case shown="1" w542 {
                      tunnel: [900.0 ("Data Entry Limits:Maximum") 40.0 ("Data Entry Limits:Maximum")] -> w545
                      frame 0, Default {
                      }
                      frame 1 {
                      }
                    }
                    n1000 = case shown="1" w541 {
                      tunnel: [900.0 ("Data Entry Limits:Maximum") 40.0 ("Data Entry Limits:Maximum")] -> w544
                      frame 0, Default {
                      }
                      frame 1 {
                      }
                    }
                    n1001 = case shown="0, 默认" w543 {
                      tunnel: [900.0 ("Data Entry Limits:Maximum") 40.0 ("Data Entry Limits:Maximum")] -> w546
                      frame 0, Default {
                      }
                      frame 1 {
                      }
                    }
                  }
                  frame False {
                    n1002 = case shown="2" w578 {
                      tunnel: [0.001 ("Data Entry Limits:Maximum") 0.005 ("Data Entry Limits:Maximum") 5e-05 ("Data Entry Limits:Maximum")] -> w577
                      tunnel: [900.0 ("Data Entry Limits:Maximum") 900.0 ("Data Entry Limits:Maximum") 10.0 ("Data Entry Limits:Maximum")] -> w576
                      frame 0, Default {
                      }
                      frame 1 {
                      }
                      frame 2 {
                      }
                    }
                    n1003 = case shown="0, 默认" w581 {
                      tunnel: [0.001 ("Data Entry Limits:Maximum") 0.005 ("Data Entry Limits:Maximum") 5e-05 ("Data Entry Limits:Maximum")] -> w579
                      tunnel: [900.0 ("Data Entry Limits:Maximum") 900.0 ("Data Entry Limits:Maximum") 10.0 ("Data Entry Limits:Maximum")] -> w580
                      frame 0, Default {
                      }
                      frame 1 {
                      }
                      frame 2 {
                      }
                    }
                    n1004 = case shown="1" w582 {
                      tunnel: [900.0 ("Data Entry Limits:Maximum") 200.0 ("Data Entry Limits:Maximum")] -> w575
                      frame 0, Default {
                      }
                      frame 1 {
                      }
                    }
                    n1005 = case shown="2" w585 {
                      tunnel: [0.001 ("Data Entry Limits:Maximum") 0.005 ("Data Entry Limits:Maximum") 5e-05 ("Data Entry Limits:Maximum")] -> w586
                      tunnel: [900.0 ("Data Entry Limits:Maximum") 900.0 ("Data Entry Limits:Maximum") 10.0 ("Data Entry Limits:Maximum")] -> w587
                      frame 0, Default {
                      }
                      frame 1 {
                      }
                      frame 2 {
                      }
                    }
                    n1006 = case shown="0, 默认" w584 {
                      tunnel: [900.0 ("Data Entry Limits:Maximum") 200.0 ("Data Entry Limits:Maximum")] -> w583
                      frame 0, Default {
                      }
                      frame 1 {
                      }
                    }
                    n1007 = case shown="0, 默认" w589 {
                      tunnel: [900.0 ("Data Entry Limits:Maximum") 200.0 ("Data Entry Limits:Maximum")] -> w592
                      frame 0, Default {
                      }
                      frame 1 {
                      }
                    }
                    n1008 = case shown="0, 默认" w588 {
                      tunnel: [900.0 ("Data Entry Limits:Maximum") 200.0 ("Data Entry Limits:Maximum")] -> w591
                      frame 0, Default {
                      }
                      frame 1 {
                      }
                    }
                    n1009 = case shown="1" w590 {
                      tunnel: [900.0 ("Data Entry Limits:Maximum") 200.0 ("Data Entry Limits:Maximum")] -> w593
                      frame 0, Default {
                      }
                      frame 1 {
                      }
                    }
                  }
                }
                n1010 = Negate(x=w502) -> (-x=w503:dbl)
                n1011 = Negate(x=w507) -> (-x=w508:dbl)
                n1012 = Negate(x=w523) -> (-x=w524:dbl)
                n1013 = Negate(x=w514) -> (-x=w515:dbl)
                n1014 = Negate(x=w521) -> (-x=w522:dbl)
                n1015 = property on="Start" class="DigNum (严格)"("Maximum"=w523, "Minimum"=w524, "Value"=-1.0 ("Start")) -> ()  [unwired: 2 in, 2 out]
                n1016 = property on="Stop" class="DigNum (严格)"("Maximum"=w521, "Minimum"=w522, "Value"=w517) -> ()  [unwired: 2 in, 2 out]
                n1017 = property on="Step" class="DigNum (严格)"("Value"=w517, "Maximum"=w520, "Minimum"=0.001 ("Data Entry Limits:Minimum")) -> ()  [unwired: 2 in, 2 out]
                n1018 = property on="Current VT" class="DigNum (严格)"("Increment"=w504, "Maximum"=w502, "Minimum"=w503) -> ()  [unwired: 2 in, 2 out]
                n1019 = property on="Voltage IT" class="DigNum (严格)"("Maximum"=w507, "Minimum"=w508) -> ()  [unwired: 2 in, 2 out]
                n1020 = property on="CompCurrIT" class="DigNum (严格)"("Increment"=w506, "Maximum"=w505, "Minimum"=w500) -> ()  [unwired: 2 in, 2 out]
                n1021 = property on="Compliance" class="DigNum (严格)"("Increment"=w519, "Maximum"=w514, "Minimum"=w515, "Value"=w500) -> ()  [unwired: 2 in, 2 out]
                n1022 = property on="Compliance" class="DigNum (严格)"("Maximum"=w501, "Minimum"=w500) -> ()  [unwired: 2 in, 2 out]
              }
            }
          }
        }
        n1023 = node-c288() -> ()  [unwired: 1 in, 1 out]
      }
      n1024 = node-c288(w66) -> ()  [unwired: 1 out]
      n1025 = node-c288(w68) -> ()  [unwired: 1 out]
    }
    frame Error {
      n1026 = One Button Dialog(message="KEITHLEY2600源表通讯异常，请检查源表是否正常打开或者接线是否正常？") -> (true=w1638:bool)  [unwired: 1 in]
      n1027 = case shown="真" w1638 {
        selector: w1638 -> [_ w1640]
        frame False {
        }
        frame True {
          n1028 = Quit LabVIEW(quit? (T)=w1640) -> ()
        }
      }
    }
  }
